vi "Beampointing_Multi_HTU_TRA_diode.vi"() -> ()   [LabVIEW 2013]
uses:
  Shared/GUI_Template/GUI_master/tcp_new_data_event.ctl
  Shared/GUI_Template/GUI_master/tcp new data cluster.ctl
  Ctrs/beam detection.ctl
  GUI_Beampointing_single_TRA/Ctrs/move.ctl
  General GUIs/Device GUIs/GUI_Cameras/Controls/Crosshair type def.ctl
  <vilib>/Utility/file.llb/Read From Spreadsheet File (string).vi
  <userlib>/_OpenG.lib/array/array.llb/Filter 1D Array with Scalar (String)__ogtk.vi
  <vilib>/Analysis/NI_AALBase.lvlib
  <vilib>/vision/NI_Vision_Development_Module.lvlib
  <vilib>/Utility/file.llb/Write To Spreadsheet File (string).vi
panel:
  in  "Position.Axis 5::98":dbl=3.9798 caption="Motor Axis 1" min=0.0 max=6.0 format="%#_6f"
  in  "Position.Axis 6::98":dbl=1.14981 caption="Motor Axis 1" min=0.0 max=6.0 format="%#_6f"
  in  "Position.Axis 5::99":dbl=-0.0 caption="Motor Axis 1" min=0.0 max=6.0 format="%#_6f"
  in  "Position.Axis 6::99":dbl=-0.0 caption="Motor Axis 1" min=0.0 max=6.0 format="%#_6f"
  in  "Position.Axis 6::97":dbl=2.92108 caption="Motor Axis 1" min=0.0 max=6.0 format="%#_6f"
  in  "Position.Axis 4::97":dbl=2.91162 caption="Motor Axis 1" min=0.0 max=6.0 format="%#_6f"
  in  "Position.Axis 5::97":dbl=5.23276 caption="Motor Axis 1" min=0.0 max=6.0 format="%#_6f"
  in  "Position.Axis 4::98":dbl=1.88847 caption="Motor Axis 1" min=0.0 max=6.0 format="%#_6f"
  in  "Position.Axis 3::99":dbl=3.28064 caption="Motor Axis 1" min=0.0 max=6.0 format="%#_6f"
  in  "Position.Axis 4::99":dbl=5.63109 caption="Motor Axis 1" min=0.0 max=6.0 format="%#_6f"
  out "error out 3":errorcluster
  out "Array 3":sgl[](array[numeric])=[7.892375, 6.4410686, 0.40833333, 2.2805147, 5.7728376, 8.5543, 6.1752, 41.382236, 0.0, 0.0, 0.0, 0.0]
  in  "GUIdevice 97":string="U_TRAServer02"
  in  "GUIdevice 98":string="U_TRAServer03"
  in  "Position.Axis 1::97":dbl=2.68788 caption="Motor Axis 1" min=0.0 max=6.0 format="%#_6f"
  in  "Position.Axis 2::97":dbl=2.50302 caption="Motor Axis 1" min=0.0 max=6.0 format="%#_6f"
  in  "Position.Axis 3::97":dbl=3.44716 caption="Motor Axis 1" min=0.0 max=6.0 format="%#_6f"
  in  "Position.Axis 1::98":dbl=2.61382 caption="Motor Axis 1" min=0.0 max=6.0 format="%#_6f"
  in  "Position.Axis 2::98":dbl=0.97888 caption="Motor Axis 1" min=0.0 max=6.0 format="%#_6f"
  in  "Position.Axis 3::98":dbl=5.18289 caption="Motor Axis 1" min=0.0 max=6.0 format="%#_6f"
  in  "save path":path=path "W:/BP_DATA"
  out "size(s) 6":i32=12
  out "config path":string="C:\\GEECS\\Developers Version\\source\\Bella center GUIs\\GUI_Beampointing_multi\\20190502_HTU_diode.cfg"
  out "motor refs 7":refnum<vi>[](array[refnum])
  out "Moving Y":string
  out "Moving X":string
  out "particles":T1(array[cluster])=[{"Area"=1173.0, "Number of Holes"=0.0, "Bounding Rect"={"Left"=82.0, "Top"=87.0, "Right"=120.0, "Bottom"=129.0}, "Center of Mass"={"X"=99.91133844842285, "Y"=109.06734867860187}, "Orientation"=119.37802063554284, "Dimensions"={"Width"=38.0, "Height"=42.0}}]
  out "motor refs 6":refnum<vi>[](array[refnum])
  out "millisecond timer value":u32=1735081648
  out "motor refs 5":refnum<vi>[](array[refnum])
  out "appended path":path=path "C:/GEECS/Developers Version/source/Bella center GUIs/GUI_Beampointing_multi/defaultDevices_ HTU_diode.txt"
  out "motor refs 4":refnum<vi>[](array[refnum])
  in  "active Axis ref 3":cluster{"Ref X":refnum<vi>, "Ref Y":refnum<vi>}
  out "motor refs 3":refnum<vi>[](array[refnum])
  in  "active man refs":cluster{"Ref X":refnum<vi>, "Ref Y":refnum<vi>}
  out "motor refs 2":refnum<vi>[](array[refnum])
  in  "Numeric":dbl=1.0
  out "Current State":string="Exit"
  in  "output cluster 2":T5 {"detection para"."smal para"."Measurement Parameter" items=["Center of Mass X", "Center of Mass Y", "First Pixel X", "First Pixel Y", "Bounding Rect Left", "Bounding Rect Top", "Bounding Rect Right", "Bounding Rect Bottom", "Max Feret Diameter Start X", "Max Feret Diameter Start Y", "Max Feret Diameter End X", "Max Feret Diameter End Y", "Max Horiz. Segment Length Left", "Max Horiz. Segment Length Right", "Max Horiz. Segment Length Row", "-", "Bounding Rect Width", "Bounding Rect Height", "Bounding Rect Diagonal", "Perimeter", "Convex Hull Perimeter", "Holes' Perimeter", "Max Feret Diameter", "Equivalent Ellipse Major Axis", "Equivalent Ellipse Minor Axis", "Equivalent Ellipse Minor Axis (Feret)", "Equivalent Rect Long Side", "Equivalent Rect Short Side", "Equivalent Rect Diagonal", "Equivalent Rect Short Side (Feret)", "Average Horiz. Segment Length", "Average Vert. Segment Length", "Hydraulic Radius", "Waddel Disk Diameter", "-", "Area", "Holes' Area", "Particle & Holes' Area", "Convex Hull Area", "Image Area", "-", "Number of Holes", "Number of Horiz. Segments", "Number of Vert. Segments", "-", "Orientation", "Max Feret Diameter Orientation", "-", "% Area/Image Area", "% Area/(Particle & Holes' Area)", "Ratio of Equivalent Ellipse Axes", "Ratio of Equivalent Rect Sides", "-", "Elongation Factor", "Compactness Factor", "Heywood Circularity Factor", "Type Factor", "-", "Sum X", "Sum Y", "Sum XX", "Sum XY", "Sum YY", "Sum XXX", "Sum XXY", "Sum XYY", "Sum YYY", "-", "Moment of Inertia XX", "Moment of Inertia XY", "Moment of Inertia YY", "Moment of Inertia XXX", "Moment of Inertia XXY", "Moment of Inertia XYY", "Moment of Inertia YYY", "Norm. Moment of Inertia XX", "Norm. Moment of Inertia XY", "Norm. Moment of Inertia YY", "Norm. Moment of Inertia XXX", "Norm. Moment of Inertia XXY", "Norm. Moment of Inertia XYY", "Norm. Moment of Inertia YYY", "Hu Moment 1", "Hu Moment 2", "Hu Moment 3", "Hu Moment 4", "Hu Moment 5", "Hu Moment 6", "Hu Moment 7"]; "detection para"."smal para"."Range Lower Value" format="%.2f"; "detection para"."smal para"."Range Upper Value" format="%.2f"; "detection para"."detection method" items=["clustering", "entropy", "metric", "moments", "inter-class variance"]; "detection para"."Filter" items=["No Filter", "Median Filter", "Low Pass Filter"]}
  out "CCDs":string[](array[string])=["UC_TubeIn", "UC_CompIn", "UC_DMSurface", "UC_BCaveIn", "UC_OAPin1", "UC_OAPin2", "UC_Beamline_In", "UC_Beamline_Out", "", "", "", ""]
  in  "GUIdevice 12":string
  in  "GUIdevice 11":string
  in  "GUIdevice 10":string
  in  "GUIdevice 9":string
  out "error out 2":errorcluster
  in  "active cams":string[](array[string])
  in  "Motor Y":dbl[][](array[numeric])
  in  "Motor X":dbl[][](array[numeric])
  out "Names":string[](array[string])=["TubeIn", "CompIn", "U_TRA1_56", "BCaveIn", "OAPIn1", "DMIn", "OAPin2", "U_TRA2_34", "Beamline_In"]
  in  "Offset X stats":dbl[][](array[numeric])
  in  "Offset Y stats":dbl[][](array[numeric])
  out "Box":T6(array[cluster])=[{"Left"=82.0, "Top"=87.0, "Right"=120.0, "Bottom"=129.0}, {"Left"=147.0, "Top"=140.0, "Right"=258.0, "Bottom"=261.0}, {"Left"=55.0, "Top"=59.0, "Right"=64.0, "Bottom"=71.0}, {"Left"=153.0, "Top"=123.0, "Right"=189.0, "Bottom"=158.0}, {"Left"=160.0, "Top"=192.0, "Right"=208.0, "Bottom"=240.0}, {"Left"=48.0, "Top"=38.0, "Right"=70.0, "Bottom"=57.0}, {"Left"=63.0, "Top"=115.0, "Right"=156.0, "Bottom"=205.0}, {"Left"=176.0, "Top"=170.0, "Right"=237.0, "Bottom"=233.0}]
  in  "Tab Cams":enum32{"Config ", "Main", "History"}(tab)=enum."Main"
  in  "associated motors":T7={"Motor CCD 1"=0, "Motor CCD 2"=1, "Motor CCD 3"=5, "Motor CCD 4"=3, "Motor CCD 5"=4, "Motor CCD 6"=6, "Motor CCD 7"=8, "Motor CCD 8"=7, "Motor CCD 9"=0, "Motor CCD 10"=0, "Motor CCD 11"=0, "Motor CCD 12"=0} {"Motor CCD 12" items=["TubeIn", "CompIn", "U_TRA1_56", "BCaveIn", "OAPIn1", "DMIn", "OAPin2", "U_TRA2_34", "Beamline_In"]; "Motor CCD 11" items=["TubeIn", "CompIn", "U_TRA1_56", "BCaveIn", "OAPIn1", "DMIn", "OAPin2", "U_TRA2_34", "Beamline_In"]; "Motor CCD 10" items=["TubeIn", "CompIn", "U_TRA1_56", "BCaveIn", "OAPIn1", "DMIn", "OAPin2", "U_TRA2_34", "Beamline_In"]; "Motor CCD 9" items=["TubeIn", "CompIn", "U_TRA1_56", "BCaveIn", "OAPIn1", "DMIn", "OAPin2", "U_TRA2_34", "Beamline_In"]; "Motor CCD 8" items=["TubeIn", "CompIn", "U_TRA1_56", "BCaveIn", "OAPIn1", "DMIn", "OAPin2", "U_TRA2_34", "Beamline_In"]; "Motor CCD 7" items=["TubeIn", "CompIn", "U_TRA1_56", "BCaveIn", "OAPIn1", "DMIn", "OAPin2", "U_TRA2_34", "Beamline_In"]; "Motor CCD 6" items=["TubeIn", "CompIn", "U_TRA1_56", "BCaveIn", "OAPIn1", "DMIn", "OAPin2", "U_TRA2_34", "Beamline_In"]; "Motor CCD 5" items=["TubeIn", "CompIn", "U_TRA1_56", "BCaveIn", "OAPIn1", "DMIn", "OAPin2", "U_TRA2_34", "Beamline_In"]; "Motor CCD 4" items=["TubeIn", "CompIn", "U_TRA1_56", "BCaveIn", "OAPIn1", "DMIn", "OAPin2", "U_TRA2_34", "Beamline_In"]; "Motor CCD 3" items=["TubeIn", "CompIn", "U_TRA1_56", "BCaveIn", "OAPIn1", "DMIn", "OAPin2", "U_TRA2_34", "Beamline_In"]; "Motor CCD 2" items=["TubeIn", "CompIn", "U_TRA1_56", "BCaveIn", "OAPIn1", "DMIn", "OAPin2", "U_TRA2_34", "Beamline_In"]; "Motor CCD 1" items=["TubeIn", "CompIn", "U_TRA1_56", "BCaveIn", "OAPIn1", "DMIn", "OAPin2", "U_TRA2_34", "Beamline_In"]}
  out "Cameras":T8={"[0]"="UC_TubeIn", "[1]"="UC_CompIn", "[2]"="UC_DMSurface", "[3]"="UC_BCaveIn", "[4]"="UC_OAPin1", "[5]"="UC_OAPin2", "[6]"="UC_Beamline_In", "[7]"="UC_Beamline_Out", "[8]"="", "[8] 2"="", "[8] 3"="", "[8] 4"=""}
  out "Status":cluster{i32, i32, "Centroid X":dbl[][]}(graph)
  in  "Exposure:12":dbl=0.095 min=0.0001 max=1.0 format="%#_6f"
  in  "Triggerdelay::12":dbl=0.003 min=0.0 max=0.09 format="%#_6f"
  in  "Exposure::11":dbl=0.095 min=0.0001 max=1.0 format="%#_6f"
  in  "Triggerdelay::11":dbl=0.003 min=0.0 max=0.09 format="%#_6f"
  in  "Exposure::10":dbl=0.095 min=0.0001 max=1.0 format="%#_6f"
  in  "Triggerdelay::10":dbl=0.003 min=0.0 max=0.09 format="%#_6f"
  in  "Exposure::9":dbl=0.095 min=2e-05 max=1.0 format="%#_6f"
  in  "Triggerdelay::9":dbl=0.003 min=30.0 max=1000000.0 format="%#_6f"
  in  "Trigger::9":bool
  in  "Trigger::10":bool caption="Trigger:10"
  in  "Trigger::11":bool
  in  "Trigger::12":bool
  in  "Target.Y::9":dbl=45.0 caption="T9y" min=0.0 max=2000.0 format="%#_6f"
  in  "Target.X::9":dbl=47.0 caption="Tx9" min=0.0 max=2000.0 format="%#_6f"
  in  "Target.Y::10":dbl=45.0 caption="T10y" min=0.0 max=2000.0 format="%#_6f"
  in  "Target.X::10":dbl=47.0 caption="T10x" min=0.0 max=2000.0 format="%#_6f"
  in  "Target.Y::11":dbl=45.0 caption="T11y" min=0.0 max=2000.0 format="%#_6f"
  in  "Target.X::11":dbl=47.0 caption="T11x" min=0.0 max=2000.0 format="%#_6f"
  in  "Target.Y::12":dbl=45.0 caption="T12y" min=0.0 max=2000.0 format="%#_6f"
  in  "Target.X::12":dbl=47.0 caption="T12x" min=0.0 max=2000.0 format="%#_6f"
  in  "Exposure::8":dbl=0.080003 min=0.0001 max=1.0 format="%#_6f"
  in  "Triggerdelay::8":dbl=150001.049042 min=20.0 max=500000.0 format="%#_6f"
  in  "Trigger::8":bool=TRUE
  in  "Target.Y::8":dbl=200.0 caption="T8y" min=0.0 max=2000.0 format="%#_6f"
  in  "Target.X::8":dbl=205.0 caption="T8x" min=0.0 max=2000.0 format="%#_6f"
  in  "Target.Y::7":dbl=162.0 caption="T7x" min=0.0 max=2000.0 format="%#_6f"
  in  "Target.X::7":dbl=110.0 caption="T7y" min=0.0 max=2000.0 format="%#_6f"
  in  "Target.Y::6":dbl=47.0 caption="T6y" min=0.0 max=2000.0 format="%#_6f"
  in  "Target.X::6":dbl=58.0 caption="T6x" min=0.0 max=2000.0 format="%#_6f"
  in  "Target.Y::5":dbl=215.0 caption="T5y" min=0.0 max=2000.0 format="%#_6f"
  in  "Target.X::5":dbl=183.0 caption="T5x" min=0.0 max=2000.0 format="%#_6f"
  in  "Target.Y::4":dbl=140.0 caption="T4y" min=0.0 max=2000.0 format="%#_6f"
  in  "Target.X::4":dbl=171.0 caption="T4x" min=0.0 max=2000.0 format="%#_6f"
  in  "Target.Y::3":dbl=65.0 caption="T3y" min=0.0 max=2000.0 format="%#_6f"
  in  "Target.X::3":dbl=59.0 caption="T3x" min=0.0 max=2000.0 format="%#_6f"
  in  "Target.Y::2":dbl=200.0 caption="T2y" min=0.0 max=2000.0 format="%#_6f"
  in  "Target.X::2":dbl=203.0 caption="T2x" min=0.0 max=2000.0 format="%#_6f"
  in  "Target.Y::1":dbl=109.0 caption="T1y" min=0.0 max=2000.0 format="%#_6f"
  in  "Target.X::1":dbl=100.0 caption="T1x" min=0.0 max=2000.0 format="%#_6f"
  in  "Exposure::7":dbl=0.049982 min=0.0001 max=1.0 format="%#_6f"
  in  "Triggerdelay::7":dbl=50000.13113 min=0.0 max=900000.0 format="%#_6f"
  in  "Trigger::7":bool=TRUE
  in  "Exposure::6":dbl=0.3 min=0.0001 max=1.0 format="%#_6f"
  in  "Triggerdelay::6":dbl=50000.0 min=1.0 max=900000.0 format="%#_6f"
  in  "Trigger::6":bool=TRUE
  in  "Exposure::5":dbl=0.2 min=0.0001 max=1.0 format="%#_6f"
  in  "Triggerdelay::5":dbl=50000.0 min=0.0 max=100000.0 format="%#_6f"
  in  "Trigger::5":bool=TRUE
  in  "Exposure::4":dbl=10000.0 min=10.0 max=1000000.0 format="%#_6f"
  in  "Triggerdelay::4":dbl=50000.0 min=10.0 max=1000000.0 format="%#_6f"
  in  "Trigger::4":bool=TRUE
  in  "Exposure::3":dbl=200000.0 min=20.0 max=1000000.0 format="%#_6f"
  in  "Triggerdelay::3":dbl=50000.0 min=10.0 max=500000.0 format="%#_6f"
  in  "Trigger::3":bool=TRUE
  in  "Exposure::2":dbl=0.01 min=2e-05 max=1.0 format="%#_6f"
  in  "Triggerdelay::2":dbl=50000.0 min=0.0 max=100000.0 format="%#_6f"
  in  "Trigger::2":bool=TRUE
  out "image::1":T9(plugin-control) caption="UC_TubeIn"
  out "image::2":T9(plugin-control) caption="UC_CompIn"
  out "image::3":T9(plugin-control) caption="UC_DMSurface"
  out "image::4":T9(plugin-control) caption="UC_BCaveIn"
  out "image::5":T9(plugin-control) caption="UC_OAPin1"
  out "image::6":T9(plugin-control) caption="UC_OAPin2"
  out "image::7":T9(plugin-control) caption="UC_Beamline_In"
  out "image::8":T9(plugin-control) caption="UC_Beamline_Out"
  in  "Exposure::1":dbl=3000.0 min=50.0 max=500000.0 format="%#_6f"
  in  "Triggerdelay::1":dbl=50000.0 min=0.01 max=999000.0 format="%#_6f"
  in  "Trigger::1":bool=TRUE
  in  "UDP error message":string
  out "required Y":bool[](array[boolean])=[FALSE, FALSE, FALSE, FALSE, TRUE, FALSE, TRUE, FALSE]
  out "required X":bool[](array[boolean])=[FALSE, FALSE, FALSE, TRUE, TRUE, FALSE, TRUE, FALSE]
  out "detected":bool[](array[boolean])=[TRUE, TRUE, TRUE, TRUE, TRUE, TRUE, TRUE, TRUE]
  out "name array":string[](array[string])=["UC_TubeIn", "UC_CompIn", "UC_DMSurface", "UC_BCaveIn", "UC_OAPin1", "UC_OAPin2", "UC_Beamline_In", "UC_Beamline_Out"]
  out "image::9":T9(plugin-control) caption="UC_ModeImager"
  out "image::10":T9(plugin-control)
  out "image::11":T9(plugin-control)
  out "image::12":T9(plugin-control)
  out "speedmode X":bool[](array[boolean])=[FALSE, FALSE, TRUE, FALSE, FALSE, FALSE, FALSE, FALSE]
  out "speedmode Y":bool[](array[boolean])=[FALSE, FALSE, TRUE, FALSE, FALSE, FALSE, FALSE, FALSE]
  out "CCD 9":cluster{timestamp[], dbl[]}[](graph)
  out "CCD 10":cluster{timestamp[], dbl[]}[](graph)
  out "CCD 11":cluster{timestamp[], dbl[]}[](graph)
  out "CCD 12":cluster{timestamp[], dbl[]}[](graph)
  out "CCD 5":cluster{timestamp[], dbl[]}[](graph)
  out "CCD 6":cluster{timestamp[], dbl[]}[](graph)
  out "CCD 7":cluster{timestamp[], dbl[]}[](graph)
  out "CCD 8":cluster{timestamp[], dbl[]}[](graph)
  out "CCD 2":cluster{timestamp[], dbl[]}[](graph)
  out "CCD 1":cluster{timestamp[], dbl[]}[](graph)
  out "CCD 3":cluster{timestamp[], dbl[]}[](graph)
  out "CCD 4":cluster{timestamp[], dbl[]}[](graph)
  in  "History Size":i32=500
  out "History Index":i32=1
  in  "Feedback Global":bool
  in  "detection para":T3[](array[typedef])=[{"Filter"=1, "Filter Para"={"X Size"=5, "Y Size"=5, "% Tolerance"=1}, "detection method"=4, "smal para"=[{"Measurement Parameter"=35, "Range Lower Value"=0.0, "Range Upper Value"=0.0, "Range"=TRUE, "Measurement Type"=FALSE}], "Remove small Objects"=TRUE, "Restrict to round Objects"=FALSE}, {"Filter"=1, "Filter Para"={"X Size"=5, "Y Size"=5, "% Tolerance"=1}, "detection method"=4, "smal para"=[{"Measurement Parameter"=35, "Range Lower Value"=0.0, "Range Upper Value"=500.0, "Range"=FALSE, "Measurement Type"=FALSE}], "Remove small Objects"=TRUE, "Restrict to round Objects"=FALSE}, {"Filter"=1, "Filter Para"={"X Size"=5, "Y Size"=5, "% Tolerance"=1}, "detection method"=4, "smal para"=[{"Measurement Parameter"=35, "Range Lower Value"=0.0, "Range Upper Value"=500.0, "Range"=TRUE, "Measurement Type"=FALSE}], "Remove small Objects"=TRUE, "Restrict to round Objects"=FALSE}, {"Filter"=1, "Filter Para"={"X Size"=5, "Y Size"=5, "% Tolerance"=1}, "detection method"=4, "smal para"=[{"Measurement Parameter"=35, "Range Lower Value"=0.0, "Range Upper Value"=500.0, "Range"=TRUE, "Measurement Type"=FALSE}], "Remove small Objects"=TRUE, "Restrict to round Objects"=FALSE}, {"Filter"=1, "Filter Para"={"X Size"=5, "Y Size"=5, "% Tolerance"=1}, "detection method"=4, "smal para"=[{"Measurement Parameter"=35, "Range Lower Value"=0.0, "Range Upper Value"=500.0, "Range"=TRUE, "Measurement Type"=FALSE}], "Remove small Objects"=TRUE, "Restrict to round Objects"=FALSE}, {"Filter"=1, "Filter Para"={"X Size"=5, "Y Size"=5, "% Tolerance"=1}, "detection method"=4, "smal para"=[{"Measurement Parameter"=35, "Range Lower Value"=0.0, "Range Upper Value"=500.0, "Range"=TRUE, "Measurement Type"=FALSE}], "Remove small Objects"=TRUE, "Restrict to round Objects"=FALSE}, {"Filter"=1, "Filter Para"={"X Size"=5, "Y Size"=5, "% Tolerance"=1}, "detection method"=4, "smal para"=[{"Measurement Parameter"=35, "Range Lower Value"=0.0, "Range Upper Value"=500.0, "Range"=TRUE, "Measurement Type"=FALSE}], "Remove small Objects"=TRUE, "Restrict to round Objects"=FALSE}, {"Filter"=1, "Filter Para"={"X Size"=5, "Y Size"=5, "% Tolerance"=1}, "detection method"=3, "smal para"=[{"Measurement Parameter"=35, "Range Lower Value"=0.0, "Range Upper Value"=0.0, "Range"=FALSE, "Measurement Type"=FALSE}], "Remove small Objects"=TRUE, "Restrict to round Objects"=FALSE}, {"Filter"=1, "Filter Para"={"X Size"=5, "Y Size"=5, "% Tolerance"=1}, "detection method"=4, "smal para"=[{"Measurement Parameter"=35, "Range Lower Value"=0.0, "Range Upper Value"=0.0, "Range"=FALSE, "Measurement Type"=FALSE}], "Remove small Objects"=TRUE, "Restrict to round Objects"=FALSE}, {"Filter"=1, "Filter Para"={"X Size"=5, "Y Size"=5, "% Tolerance"=1}, "detection method"=4, "smal para"=[{"Measurement Parameter"=35, "Range Lower Value"=0.0, "Range Upper Value"=500.0, "Range"=TRUE, "Measurement Type"=FALSE}], "Remove small Objects"=TRUE, "Restrict to round Objects"=FALSE}, {"Filter"=1, "Filter Para"={"X Size"=5, "Y Size"=5, "% Tolerance"=1}, "detection method"=4, "smal para"=[{"Measurement Parameter"=35, "Range Lower Value"=0.0, "Range Upper Value"=500.0, "Range"=TRUE, "Measurement Type"=FALSE}], "Remove small Objects"=TRUE, "Restrict to round Objects"=FALSE}, {"Filter"=1, "Filter Para"={"X Size"=5, "Y Size"=5, "% Tolerance"=1}, "detection method"=4, "smal para"=[{"Measurement Parameter"=35, "Range Lower Value"=0.0, "Range Upper Value"=500.0, "Range"=TRUE, "Measurement Type"=FALSE}], "Remove small Objects"=TRUE, "Restrict to round Objects"=FALSE}] {"smal para"."Measurement Parameter" items=["Center of Mass X", "Center of Mass Y", "First Pixel X", "First Pixel Y", "Bounding Rect Left", "Bounding Rect Top", "Bounding Rect Right", "Bounding Rect Bottom", "Max Feret Diameter Start X", "Max Feret Diameter Start Y", "Max Feret Diameter End X", "Max Feret Diameter End Y", "Max Horiz. Segment Length Left", "Max Horiz. Segment Length Right", "Max Horiz. Segment Length Row", "-", "Bounding Rect Width", "Bounding Rect Height", "Bounding Rect Diagonal", "Perimeter", "Convex Hull Perimeter", "Holes' Perimeter", "Max Feret Diameter", "Equivalent Ellipse Major Axis", "Equivalent Ellipse Minor Axis", "Equivalent Ellipse Minor Axis (Feret)", "Equivalent Rect Long Side", "Equivalent Rect Short Side", "Equivalent Rect Diagonal", "Equivalent Rect Short Side (Feret)", "Average Horiz. Segment Length", "Average Vert. Segment Length", "Hydraulic Radius", "Waddel Disk Diameter", "-", "Area", "Holes' Area", "Particle & Holes' Area", "Convex Hull Area", "Image Area", "-", "Number of Holes", "Number of Horiz. Segments", "Number of Vert. Segments", "-", "Orientation", "Max Feret Diameter Orientation", "-", "% Area/Image Area", "% Area/(Particle & Holes' Area)", "Ratio of Equivalent Ellipse Axes", "Ratio of Equivalent Rect Sides", "-", "Elongation Factor", "Compactness Factor", "Heywood Circularity Factor", "Type Factor", "-", "Sum X", "Sum Y", "Sum XX", "Sum XY", "Sum YY", "Sum XXX", "Sum XXY", "Sum XYY", "Sum YYY", "-", "Moment of Inertia XX", "Moment of Inertia XY", "Moment of Inertia YY", "Moment of Inertia XXX", "Moment of Inertia XXY", "Moment of Inertia XYY", "Moment of Inertia YYY", "Norm. Moment of Inertia XX", "Norm. Moment of Inertia XY", "Norm. Moment of Inertia YY", "Norm. Moment of Inertia XXX", "Norm. Moment of Inertia XXY", "Norm. Moment of Inertia XYY", "Norm. Moment of Inertia YYY", "Hu Moment 1", "Hu Moment 2", "Hu Moment 3", "Hu Moment 4", "Hu Moment 5", "Hu Moment 6", "Hu Moment 7"]; "smal para"."Range Lower Value" format="%.2f"; "smal para"."Range Upper Value" format="%.2f"; "detection method" items=["clustering", "entropy", "metric", "moments", "inter-class variance"]; "Filter" items=["No Filter", "Median Filter", "Low Pass Filter"]}
  in  "GUIdevice 8":string="UC_Beamline_Out"
  in  "Tab Control":T10(tab)
  in  "alarms":bool
  in  "new tdms":bool
  in  "Save Stats":bool
  in  "Save Config":bool
  in  "Load Config":bool
  in  "update speed [ms]":i32=1000
  in  "img to avg":i32=10 min=3 max=200
  in  "Reset History":bool
  in  "autodetect":bool
  in  "Detection Rate":dbl=0.9 min=0.001 max=1.0
  in  "Center":bool
  in  "Align":bool=TRUE
  in  "Speedmode":dbl=10.0 min=1.0 max=20.0
  in  "device ini":bool
  in  "average centroid":bool
  in  "beam detection para":T3={"Filter"=1, "Filter Para"={"X Size"=5, "Y Size"=5, "% Tolerance"=10}, "detection method"=4, "smal para"=[{"Measurement Parameter"=35, "Range Lower Value"=500.0, "Range Upper Value"=2000.0, "Range"=FALSE, "Measurement Type"=FALSE}], "Remove small Objects"=TRUE, "Restrict to round Objects"=FALSE} {"smal para"."Measurement Parameter" items=["Center of Mass X", "Center of Mass Y", "First Pixel X", "First Pixel Y", "Bounding Rect Left", "Bounding Rect Top", "Bounding Rect Right", "Bounding Rect Bottom", "Max Feret Diameter Start X", "Max Feret Diameter Start Y", "Max Feret Diameter End X", "Max Feret Diameter End Y", "Max Horiz. Segment Length Left", "Max Horiz. Segment Length Right", "Max Horiz. Segment Length Row", "-", "Bounding Rect Width", "Bounding Rect Height", "Bounding Rect Diagonal", "Perimeter", "Convex Hull Perimeter", "Holes' Perimeter", "Max Feret Diameter", "Equivalent Ellipse Major Axis", "Equivalent Ellipse Minor Axis", "Equivalent Ellipse Minor Axis (Feret)", "Equivalent Rect Long Side", "Equivalent Rect Short Side", "Equivalent Rect Diagonal", "Equivalent Rect Short Side (Feret)", "Average Horiz. Segment Length", "Average Vert. Segment Length", "Hydraulic Radius", "Waddel Disk Diameter", "-", "Area", "Holes' Area", "Particle & Holes' Area", "Convex Hull Area", "Image Area", "-", "Number of Holes", "Number of Horiz. Segments", "Number of Vert. Segments", "-", "Orientation", "Max Feret Diameter Orientation", "-", "% Area/Image Area", "% Area/(Particle & Holes' Area)", "Ratio of Equivalent Ellipse Axes", "Ratio of Equivalent Rect Sides", "-", "Elongation Factor", "Compactness Factor", "Heywood Circularity Factor", "Type Factor", "-", "Sum X", "Sum Y", "Sum XX", "Sum XY", "Sum YY", "Sum XXX", "Sum XXY", "Sum XYY", "Sum YYY", "-", "Moment of Inertia XX", "Moment of Inertia XY", "Moment of Inertia YY", "Moment of Inertia XXX", "Moment of Inertia XXY", "Moment of Inertia XYY", "Moment of Inertia YYY", "Norm. Moment of Inertia XX", "Norm. Moment of Inertia XY", "Norm. Moment of Inertia YY", "Norm. Moment of Inertia XXX", "Norm. Moment of Inertia XXY", "Norm. Moment of Inertia XYY", "Norm. Moment of Inertia YYY", "Hu Moment 1", "Hu Moment 2", "Hu Moment 3", "Hu Moment 4", "Hu Moment 5", "Hu Moment 6", "Hu Moment 7"]; "smal para"."Range Lower Value" format="%.2f"; "smal para"."Range Upper Value" format="%.2f"; "detection method" items=["clustering", "entropy", "metric", "moments", "inter-class variance"]; "Filter" items=["No Filter", "Median Filter", "Low Pass Filter"]}
  in  "move config":T2={"Tolerance [%]"=0.5, "Stepsize"=0.001, "Invert Axis"=FALSE, "Invert Direction X"=TRUE, "Invert Direction Y"=FALSE, "enable feedback"=TRUE, "Set Centriod Target"=FALSE}
  in  "Position 2":dbl=1.53813 caption="Stepsize" min=0.0 max=999999.0 format="%_6f"
  in  "Position 1":dbl=1.96058 caption="Stepsize" min=0.0 max=999999.0 format="%_6f"
  in  "Right":bool caption="RelativeMove.Axis 1.CCW::1"
  in  "Left":bool caption="RelativeMove.Axis 1.CW::1"
  in  "Down":bool caption="RelativeMove.Axis. 2.CCW::1"
  in  "Up":bool caption="RelativeMove.Axis 2.CW::1"
  in  "StepSize":dbl=1.0 caption="Stepsize" min=0.0 max=1.0 step=0.001 format="%#_6p"
  in  "active axis refs 2":T11(array[cluster])
  in  "active Axis ref":cluster{"Ref X":refnum<vi>, "Ref Y":refnum<vi>}
  in  "CCDs":u16(ring) items=["UC_TubeIn", "UC_CompIn", "UC_DMSurface", "UC_BCaveIn", "UC_OAPin1", "UC_OAPin2", "UC_Beamline_In", "UC_Beamline_Out", "UC_ModeImager", "", "", ""]
  out "motor refs":refnum<vi>[](array[refnum])
  in  "Position.Axis 2::99":dbl=1.53813 caption="Motor Axis 1" min=0.0 max=6.0 format="%#_6f"
  in  "Position.Axis 1::99":dbl=1.96058 caption="Motor Axis 1" min=0.0 max=6.0 format="%#_6f"
  in  "GUIdevice 99":string="U_TRAServer01"
  in  "move properties":T2[](array[typedef])=[{"Tolerance [%]"=0.1, "Stepsize"=0.0001, "Invert Axis"=TRUE, "Invert Direction X"=FALSE, "Invert Direction Y"=TRUE, "enable feedback"=FALSE, "Set Centriod Target"=FALSE}, {"Tolerance [%]"=0.1, "Stepsize"=0.0001, "Invert Axis"=TRUE, "Invert Direction X"=FALSE, "Invert Direction Y"=TRUE, "enable feedback"=FALSE, "Set Centriod Target"=FALSE}, {"Tolerance [%]"=0.1, "Stepsize"=0.0001, "Invert Axis"=TRUE, "Invert Direction X"=FALSE, "Invert Direction Y"=TRUE, "enable feedback"=FALSE, "Set Centriod Target"=FALSE}, {"Tolerance [%]"=0.1, "Stepsize"=0.0001, "Invert Axis"=TRUE, "Invert Direction X"=FALSE, "Invert Direction Y"=TRUE, "enable feedback"=FALSE, "Set Centriod Target"=FALSE}, {"Tolerance [%]"=0.1, "Stepsize"=0.0001, "Invert Axis"=TRUE, "Invert Direction X"=FALSE, "Invert Direction Y"=TRUE, "enable feedback"=FALSE, "Set Centriod Target"=FALSE}, {"Tolerance [%]"=0.1, "Stepsize"=0.0001, "Invert Axis"=TRUE, "Invert Direction X"=FALSE, "Invert Direction Y"=TRUE, "enable feedback"=FALSE, "Set Centriod Target"=FALSE}, {"Tolerance [%]"=0.1, "Stepsize"=0.0001, "Invert Axis"=TRUE, "Invert Direction X"=FALSE, "Invert Direction Y"=TRUE, "enable feedback"=FALSE, "Set Centriod Target"=FALSE}, {"Tolerance [%]"=0.1, "Stepsize"=0.0001, "Invert Axis"=TRUE, "Invert Direction X"=FALSE, "Invert Direction Y"=TRUE, "enable feedback"=FALSE, "Set Centriod Target"=FALSE}, {"Tolerance [%]"=0.1, "Stepsize"=0.0001, "Invert Axis"=TRUE, "Invert Direction X"=FALSE, "Invert Direction Y"=TRUE, "enable feedback"=FALSE, "Set Centriod Target"=FALSE}, {"Tolerance [%]"=0.1, "Stepsize"=0.0001, "Invert Axis"=TRUE, "Invert Direction X"=FALSE, "Invert Direction Y"=TRUE, "enable feedback"=FALSE, "Set Centriod Target"=FALSE}, {"Tolerance [%]"=0.1, "Stepsize"=0.0001, "Invert Axis"=TRUE, "Invert Direction X"=FALSE, "Invert Direction Y"=TRUE, "enable feedback"=FALSE, "Set Centriod Target"=FALSE}, {"Tolerance [%]"=0.1, "Stepsize"=0.0001, "Invert Axis"=TRUE, "Invert Direction X"=FALSE, "Invert Direction Y"=TRUE, "enable feedback"=FALSE, "Set Centriod Target"=FALSE}, {"Tolerance [%]"=0.1, "Stepsize"=0.0001, "Invert Axis"=TRUE, "Invert Direction X"=FALSE, "Invert Direction Y"=TRUE, "enable feedback"=FALSE, "Set Centriod Target"=FALSE}]
  in  "Time":timestamp[][](array[timestamp])
  in  "Mean Size":dbl[][](array[numeric])
  in  "Size":dbl[][](array[numeric])
  in  "active CCDs":i32(listbox)=1
  in  "Offset Y":dbl[][](array[numeric])
  in  "Offset X":dbl[][](array[numeric])
  in  "Mean Centroid X":dbl[][](array[numeric])
  in  "Mean Centroid Y":dbl[][](array[numeric])
  in  "Centroid Y":dbl[][](array[numeric])
  in  "Centroid X":dbl[][](array[numeric])
  in  "GUIdevice 7":string="UC_Beamline_In"
  in  "GUIdevice 6":string="UC_OAPin2"
  in  "GUIdevice 5":string="UC_OAPin1"
  in  "GUIdevice 4":string="UC_BCaveIn"
  in  "GUIdevice 3":string="UC_DMSurface"
  in  "GUIdevice 2":string="UC_CompIn"
  in  "insert tag":bool=TRUE
  in  "stop":bool
  in  "GUIdevice 1":string="UC_TubeIn"
  out "tcp data event":T12
  out "error IO 2":errorcluster
  # "max"
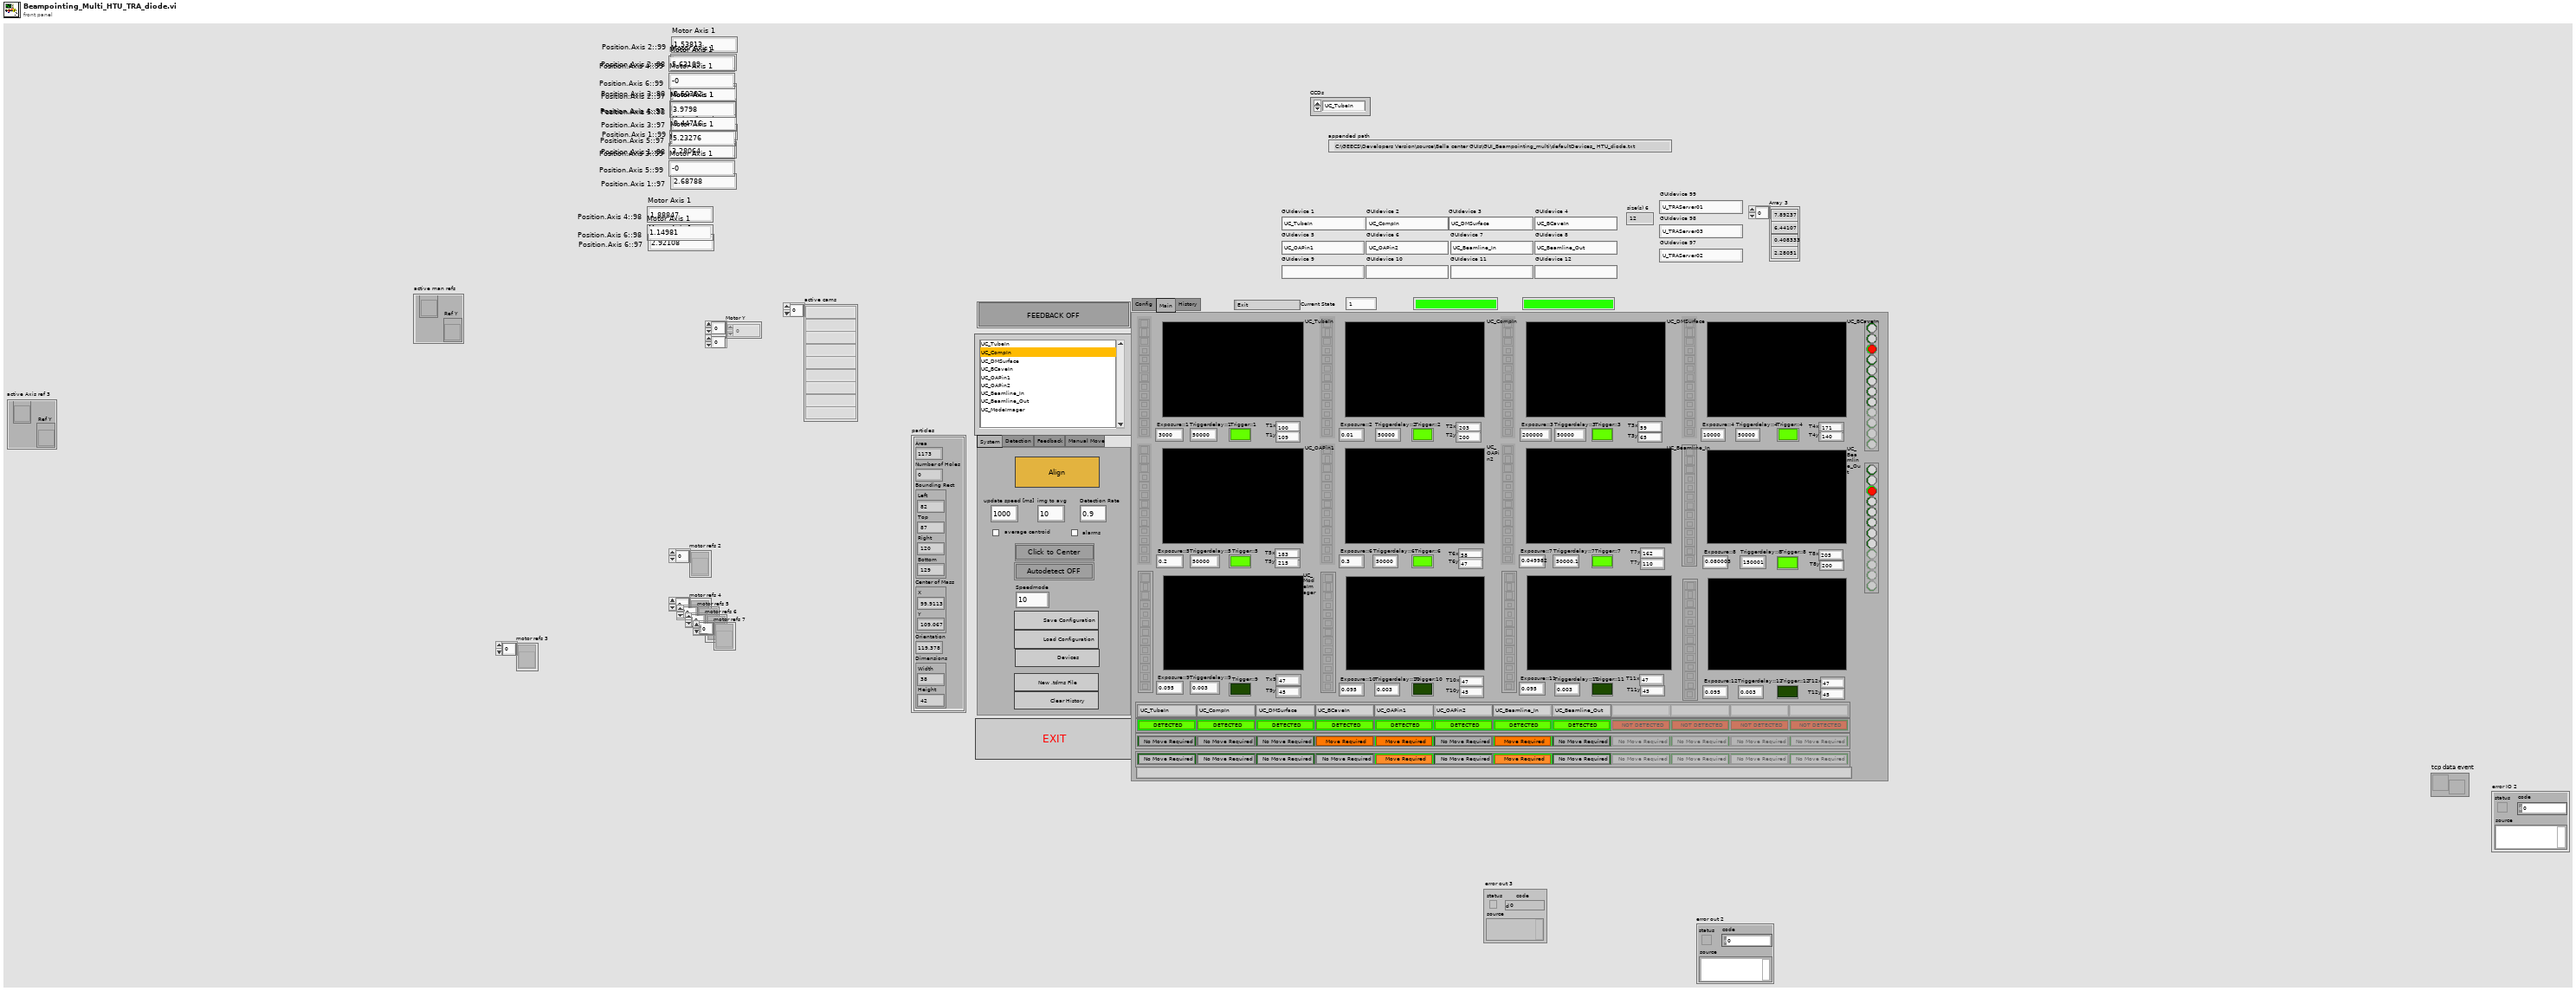
[diagram p1: front panel]
types:
  T1 = cluster{"Area":dbl, "Number of Holes":dbl, "Bounding Rect":cluster{"Left":dbl, "Top":dbl, "Right":dbl, "Bottom":dbl}, "Center of Mass":cluster{"X":dbl, "Y":dbl}, "Orientation":dbl, "Dimensions":cluster{"Width":dbl, "Height":dbl}}[]
  T2 = typedef "move.ctl" = cluster{"Tolerance [%]":dbl, "Stepsize":dbl, "Invert Axis":bool, "Invert Direction X":bool, "Invert Direction Y":bool, "enable feedback":bool, "Set Centriod Target":bool}
  T3 = typedef "beam detection.ctl" = cluster{"Filter":u16, "Filter Para":cluster{"X Size":i32, "Y Size":i32, "% Tolerance":i32}, "detection method":i32, "smal para":cluster{"Measurement Parameter":T4, "Range Lower Value":dbl, "Range Upper Value":dbl, "Range":bool, "Measurement Type":bool}[], "Remove small Objects":bool, "Restrict to round Objects":bool}
  T4 = typedef "Particle Parameters" = i32
  T5 = cluster{"CCDs":string[], "move properties":T2[], "detection para":T3[], "thresholds":cluster{"Lower value":sgl, "Upper value":sgl}[], "Value":cluster{"Motor CCD 1":u16, "Motor CCD 2":u16, "Motor CCD 3":u16, "Motor CCD 4":u16, "Motor CCD 5":u16, "Motor CCD 6":u16, "Motor CCD 7":u16, "Motor CCD 8":u16, "Motor CCD 9":u16, "Motor CCD 10":u16, "Motor CCD 11":u16, "Motor CCD 12":u16}}
  T6 = cluster{"Left":dbl, "Top":dbl, "Right":dbl, "Bottom":dbl}[]
  T7 = cluster{"Motor CCD 1":u16, "Motor CCD 2":u16, "Motor CCD 3":u16, "Motor CCD 4":u16, "Motor CCD 5":u16, "Motor CCD 6":u16, "Motor CCD 7":u16, "Motor CCD 8":u16, "Motor CCD 9":u16, "Motor CCD 10":u16, "Motor CCD 11":u16, "Motor CCD 12":u16}
  T8 = cluster{"[0]":string, "[1]":string, "[2]":string, "[3]":string, "[4]":string, "[5]":string, "[6]":string, "[7]":string, "[8]":string, "[8] 2":string, "[8] 3":string, "[8] 4":string}
  T9 = typedef "IMAQ Image.ctl" = refnum<image>
  T10 = enum32{"System", "Detection", "Feedback", "Manual Move"}
  T11 = cluster{"Ref X":refnum<vi>, "Ref Y":refnum<vi>}[]
  T12 = typedef "tcp_new_data_event.ctl" = refnum<user-event>
  T13 = typedef "tcp new data cluster.ctl" = cluster{"EventEnum":enum16{"new data", "connection status update"}, "Device name":string}
  T14 = enum32{"invalid app kind", "Development System", "Run Time System", "Student Edition", "Embedded LabVIEW", "Evaluation", "Custom"}
  T15 = enum16{"open", "open or create", "create or replace", "create", "open (read-only)"}
  T16 = enum32{"Invalid", "Standard", "Closed", "Hidden", "Minimized", "Maximized"}
  T17 = enum16{"open", "replace", "create", "open or create", "replace or create", "replace or create with confirmation"}
  T18 = enum8{"Enabled", "Disabled", "Disabled and Grayed Out"}
  T19 = typedef "Image Type" = u32
  T20 = cluster{"[0]":string, "[1]":string, "[2]":string, "[3]":string, "[4]":string, "[5]":string, "[6]":string, "[7]":string, "[8]":string, "[9]":string, "[10]":string, "[11]":string}
  T21 = cluster{"Target.X::1":refnum<vi>, "Target.Y::1":refnum<vi>}
  T22 = cluster{"Target.X::2":refnum<vi>, "Target.Y::2":refnum<vi>}
  T23 = cluster{"Target.X::3":refnum<vi>, "Target.Y::3":refnum<vi>}
  T24 = cluster{"Target.X::4":refnum<vi>, "Target.Y::4":refnum<vi>}
  T25 = cluster{"Target.X::5":refnum<vi>, "Target.Y::5":refnum<vi>}
  T26 = cluster{"Target.X::6":refnum<vi>, "Target.Y::6":refnum<vi>}
  T27 = cluster{"Target.X::7":refnum<vi>, "Target.Y::7":refnum<vi>}
  T28 = cluster{"Target.X::8":refnum<vi>, "Target.Y::8":refnum<vi>}
  T29 = cluster{"Target.X::12":refnum<vi>, "Target.Y::12":refnum<vi>}
  T30 = cluster{"Target.X::9":refnum<vi>, "Target.Y::9":refnum<vi>}
  T31 = cluster{"Target.X::10":refnum<vi>, "Target.Y::10":refnum<vi>}
  T32 = cluster{"Target.X::11":refnum<vi>, "Target.Y::11":refnum<vi>}
  T33 = cluster{"Target.X::12":refnum<vi>, "Target.Y::12":refnum<vi>}[]
  T34 = cluster{"Left":dbl, "Top":dbl, "Right":dbl, "Bottom":dbl}
  T35 = cluster{"Core":cluster{"Current VI Reference":refnum<vi>, "Close Panel on Exit?":bool}, "detection para":T3[], "thresholds":cluster{"Lower value":sgl, "Upper value":sgl}[], "Centroid X":dbl[][], "Centroid Y":dbl[][], "img to avg":i32, "Mean Centroid X":dbl[][], "Mean Centroid Y":dbl[][], "Offset X":dbl[][], "Offset Y":dbl[][], "Offset X stats ":dbl[][], "Offset Y stats ":dbl[][], "Size":dbl[][], "Mean Size":dbl[][], "Time":timestamp[][], "move properties":T2[], "active axis refs 2":cluster{"Ref X":refnum<vi>, "Ref Y":refnum<vi>}[], "active ccd":i32, "Feedback global":bool, "Motor X":dbl[][], "Motor Y":dbl[][], "active cams":string[], "Data Value Reference out":refnum<k34>, "active man refs":cluster{"Ref X":refnum<vi>, "Ref Y":refnum<vi>}, "detected":bool[], "speedmode X":bool[], "speedmode Y":bool[], "steps speed X":dbl[], "steps speed Y":dbl[]}
  T36 = cluster{"Current VI Reference":refnum<vi>, "Close Panel on Exit?":bool}
  T37 = cluster{"appended array":timestamp[], "appended array":dbl[]}
  T38 = cluster{"appended array":timestamp[], "appended array":dbl[]}[]
  T39 = typedef "Crosshair type def.ctl" = cluster{"Draw":bool, "Target":cluster{"x":dbl, "y":dbl}, "Size":cluster{"x":dbl, "y":dbl}, "Angle":dbl, "Color":u32, "Thickness":u8, "CrosshairLabel":string}
  T40 = cluster{"Left":i32, "Top":i32, "Right":i32, "Bottom":i32}
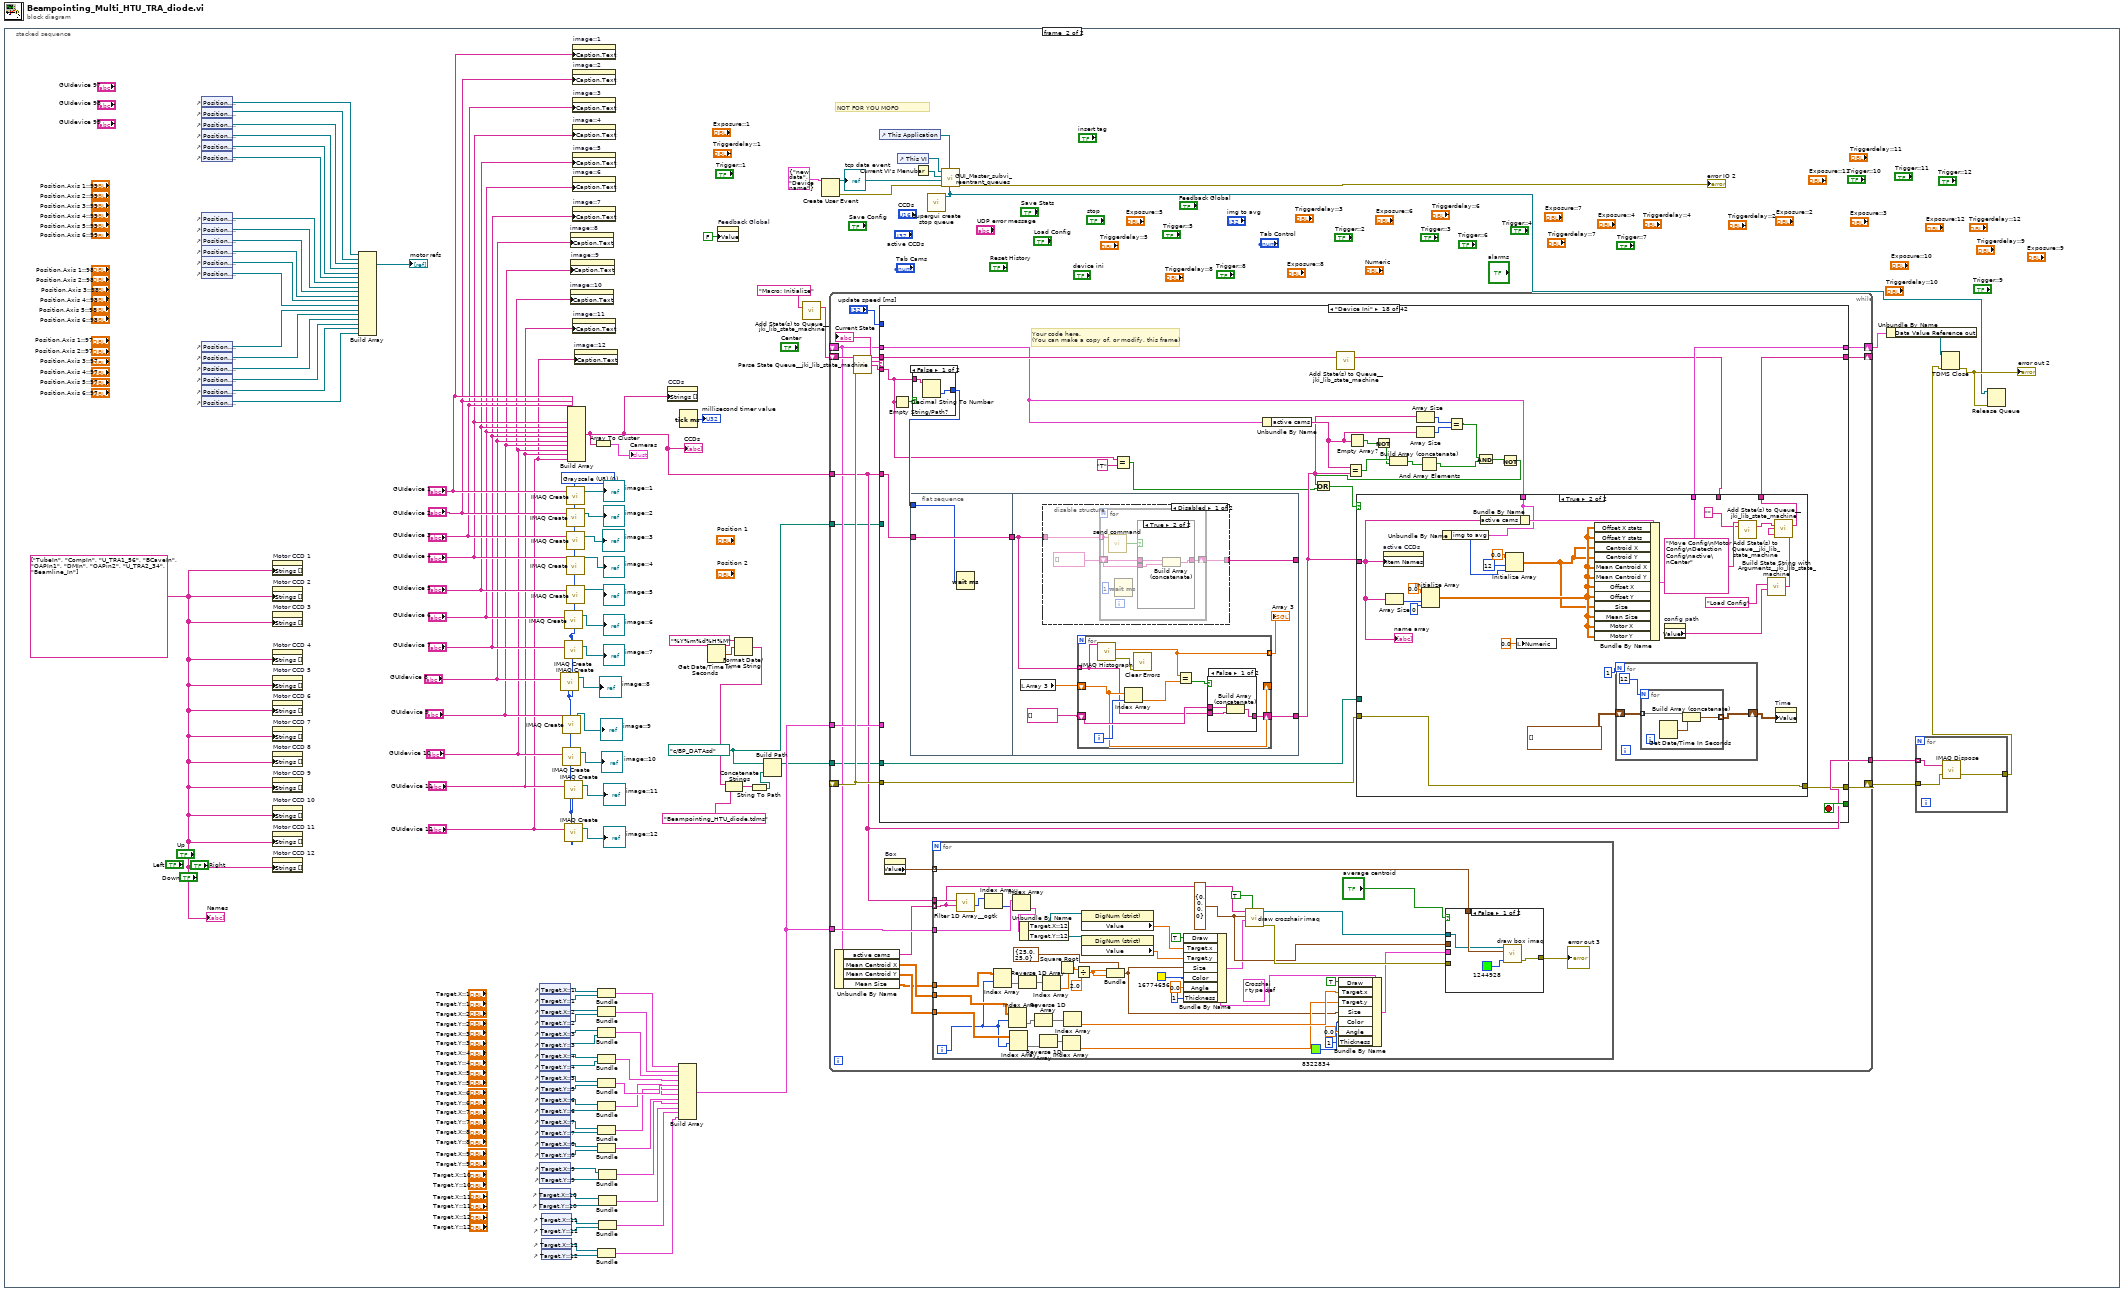
[diagram p0: block diagram]
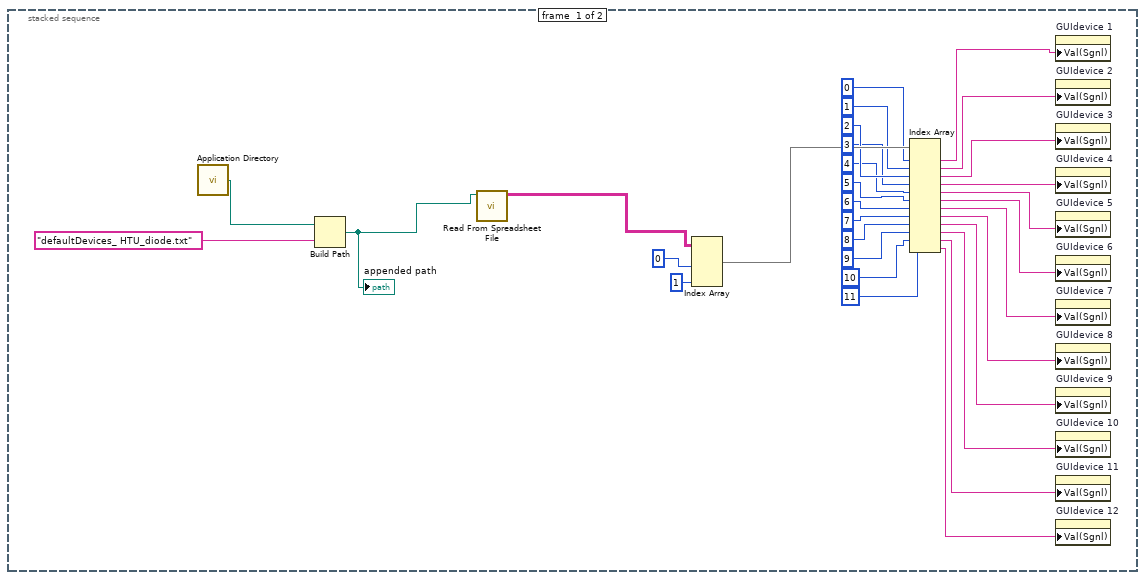
[diagram p2: hidden frame]
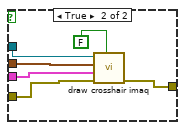
[diagram p3: hidden frame]
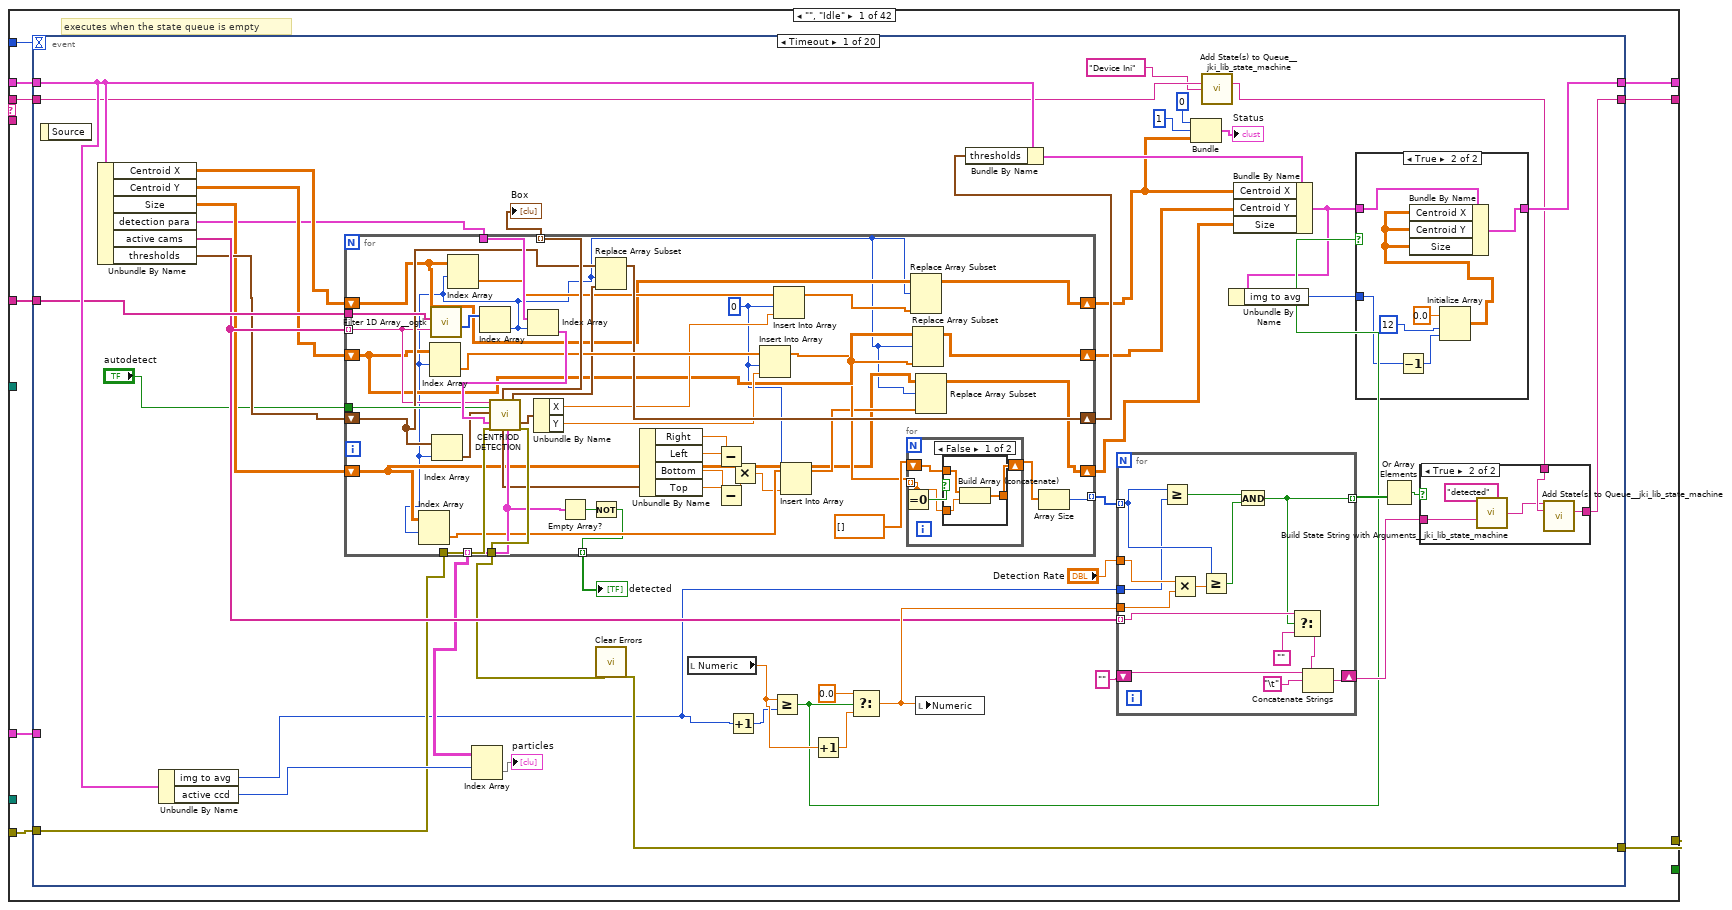
[diagram p4: hidden frame]
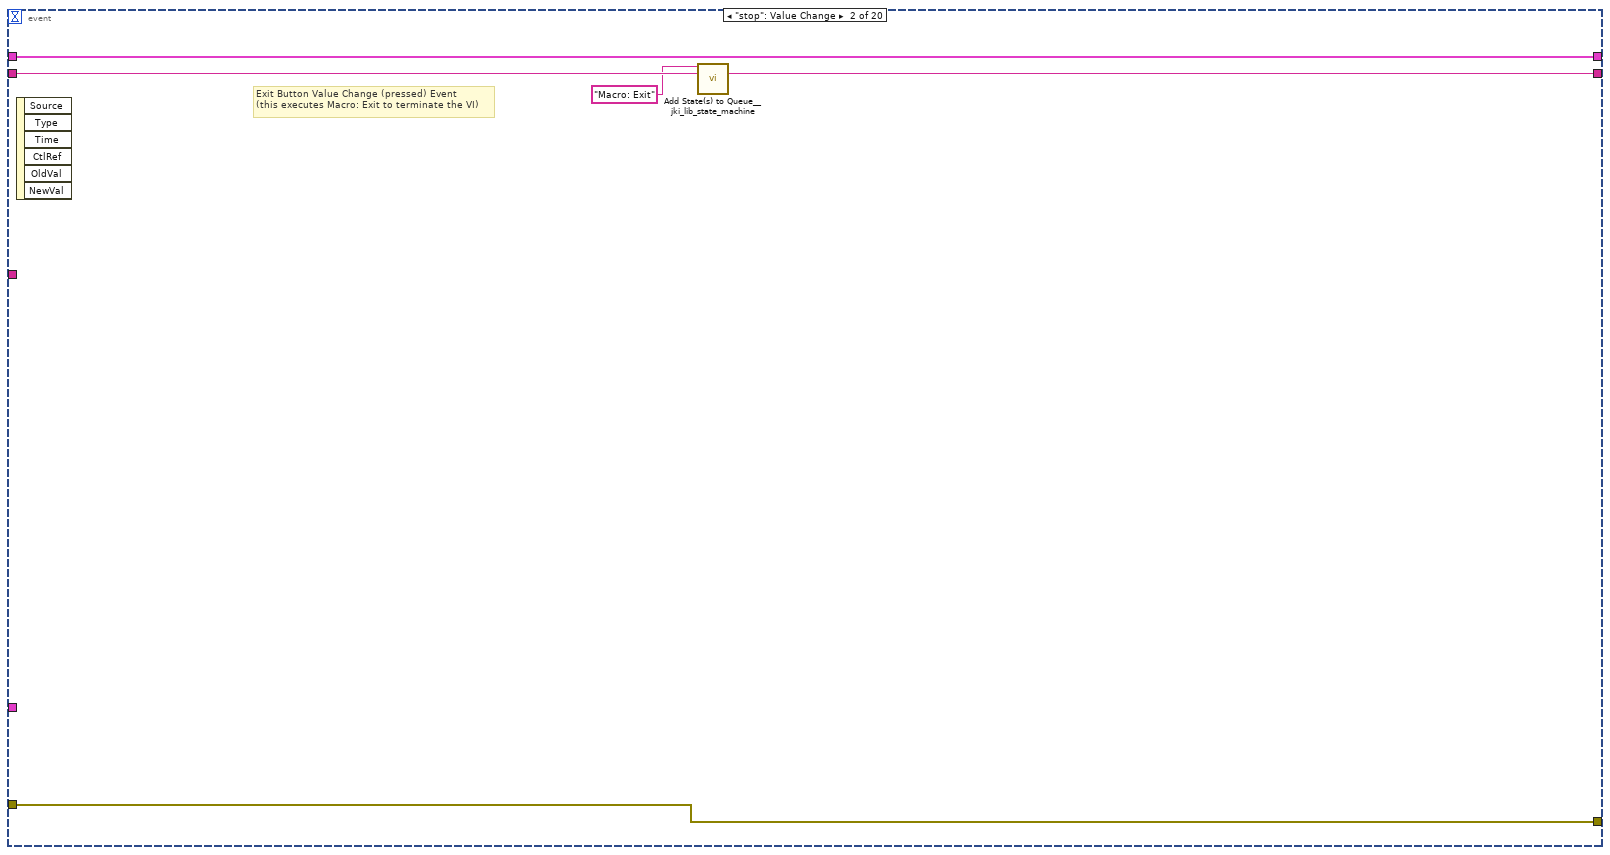
[diagram p8: hidden frame]
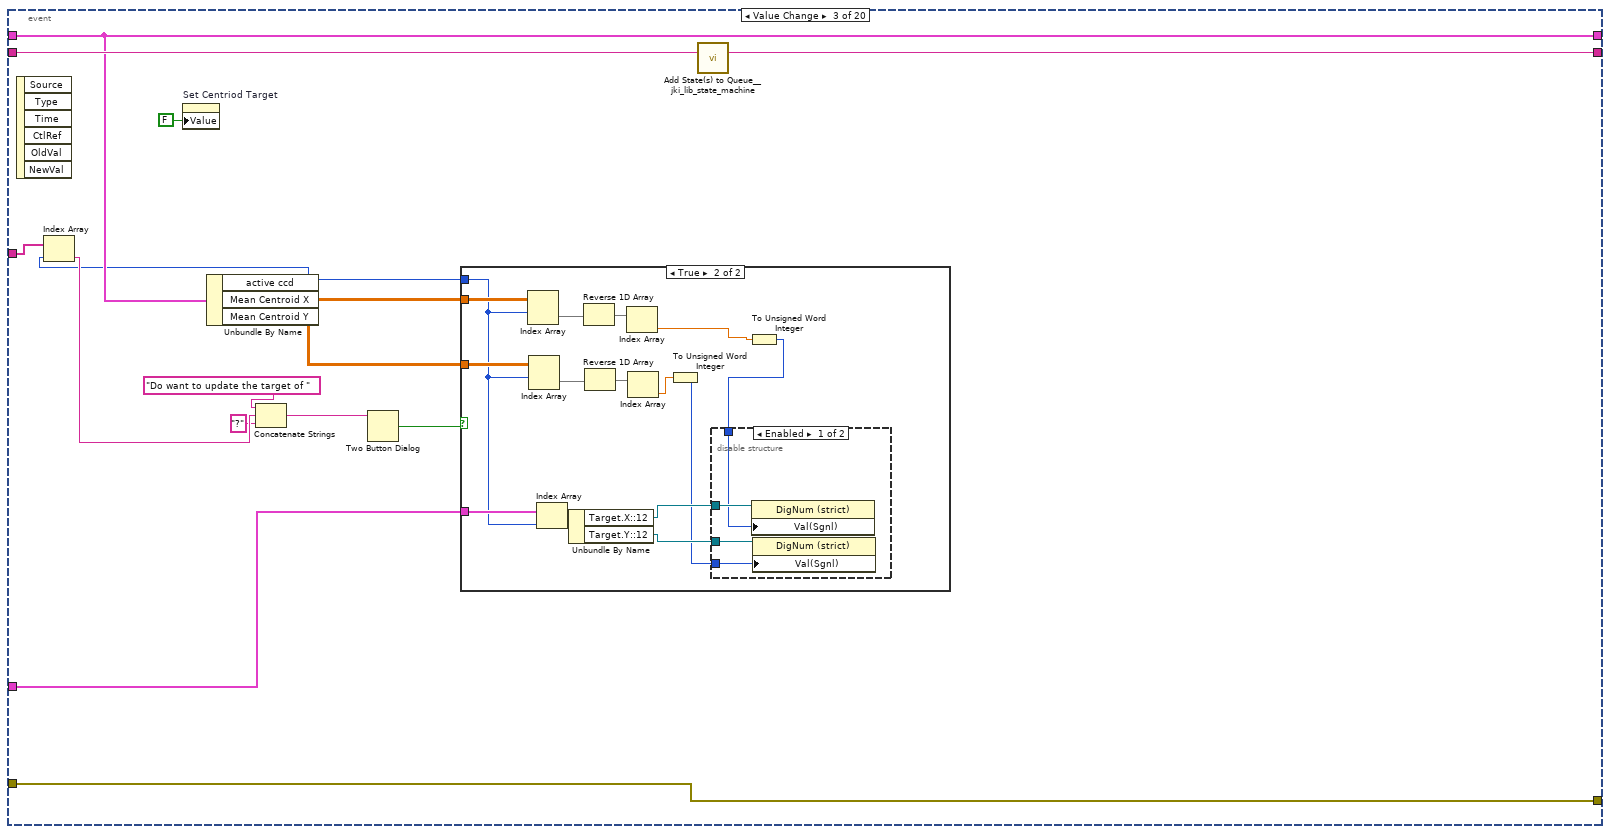
[diagram p9: hidden frame]
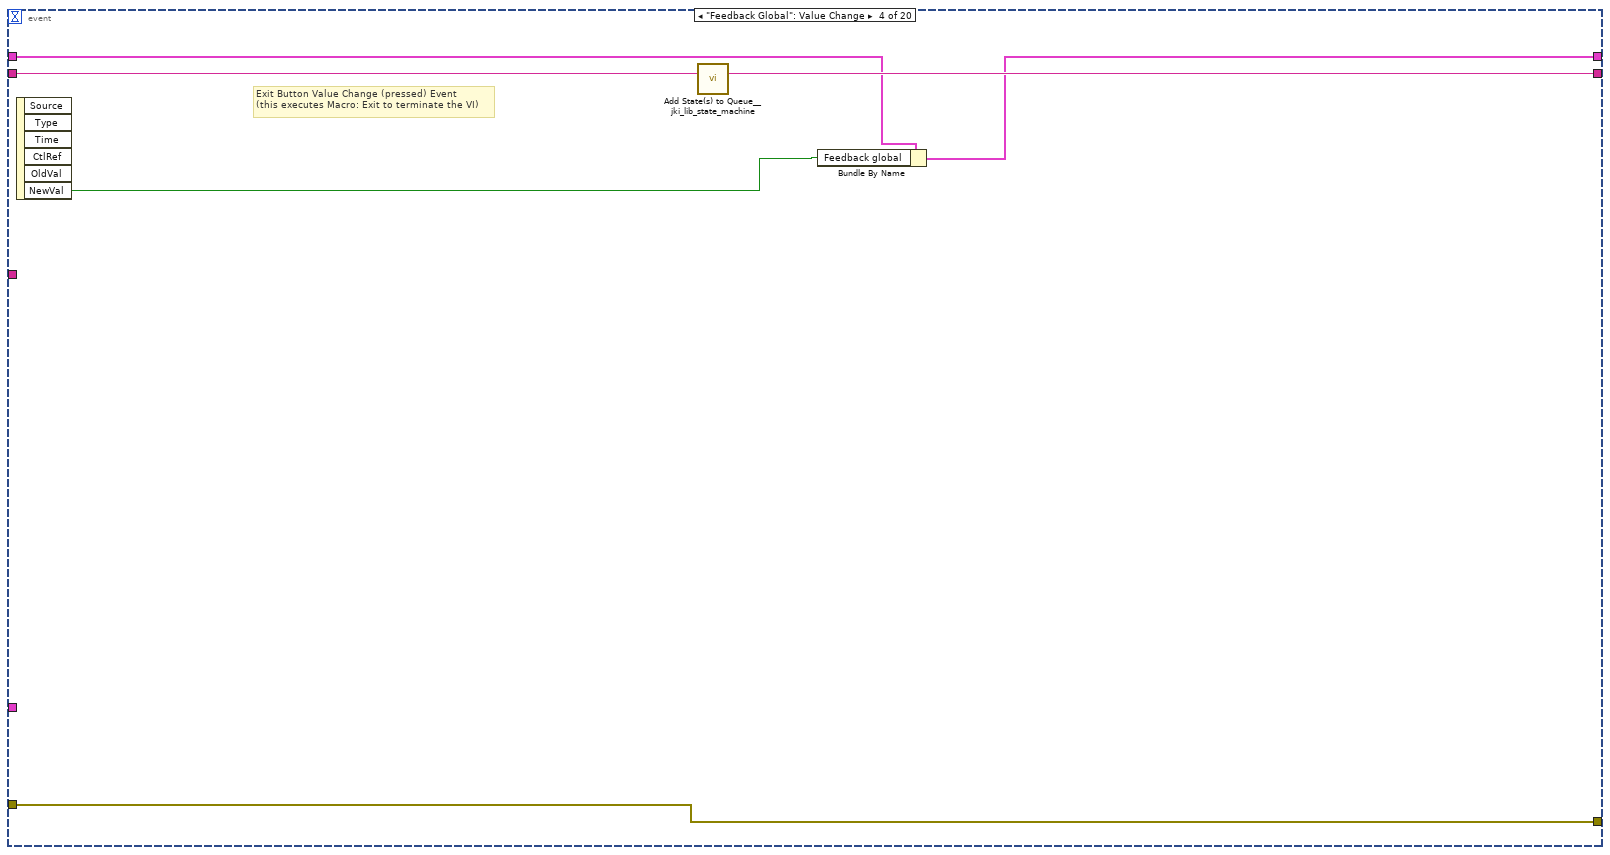
[diagram p12: hidden frame]
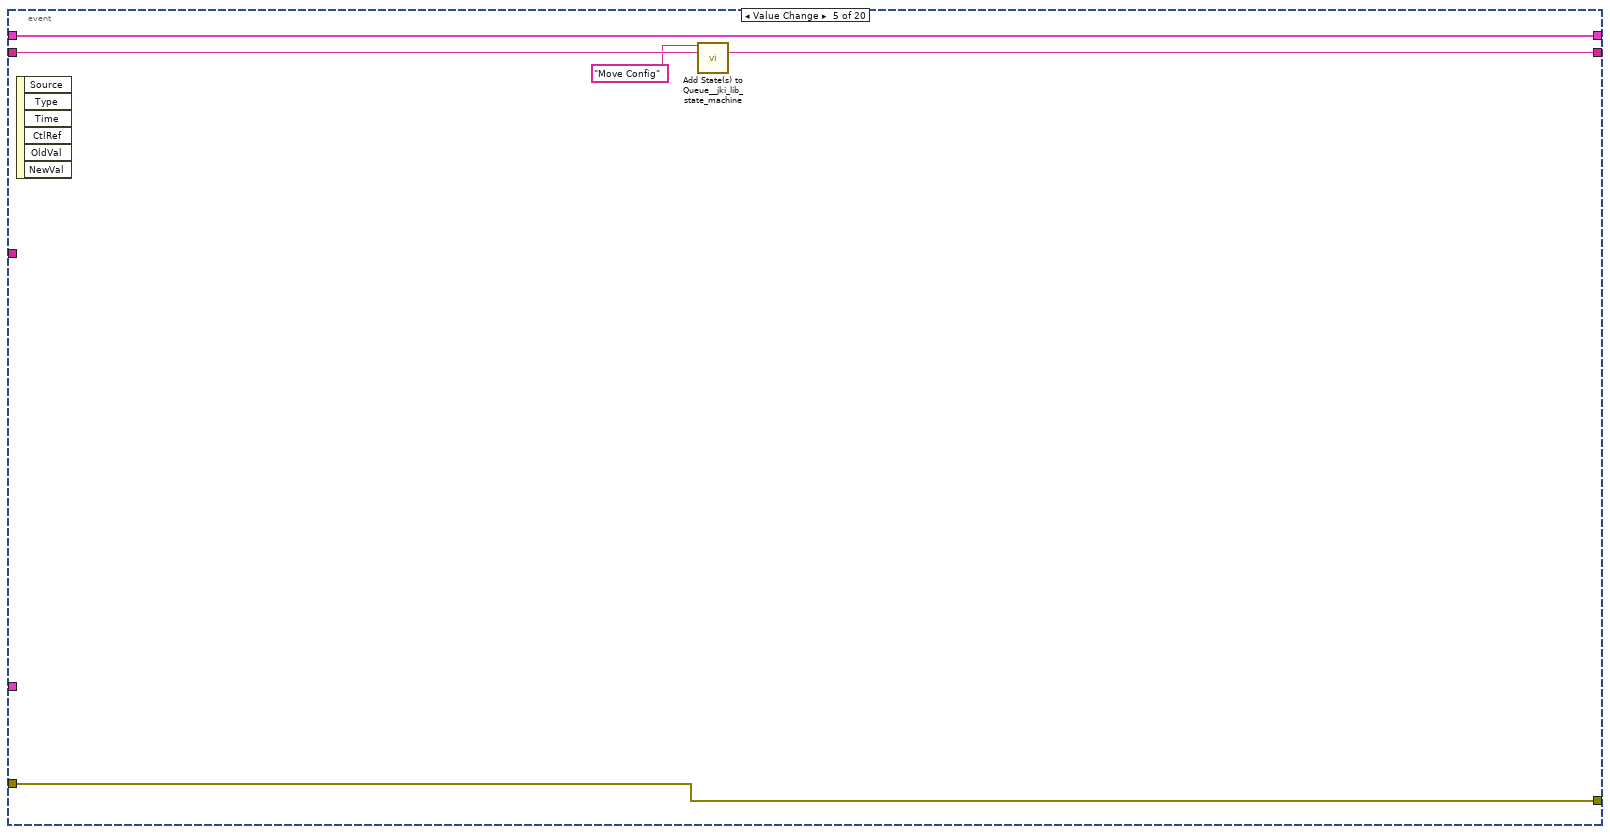
[diagram p13: hidden frame]
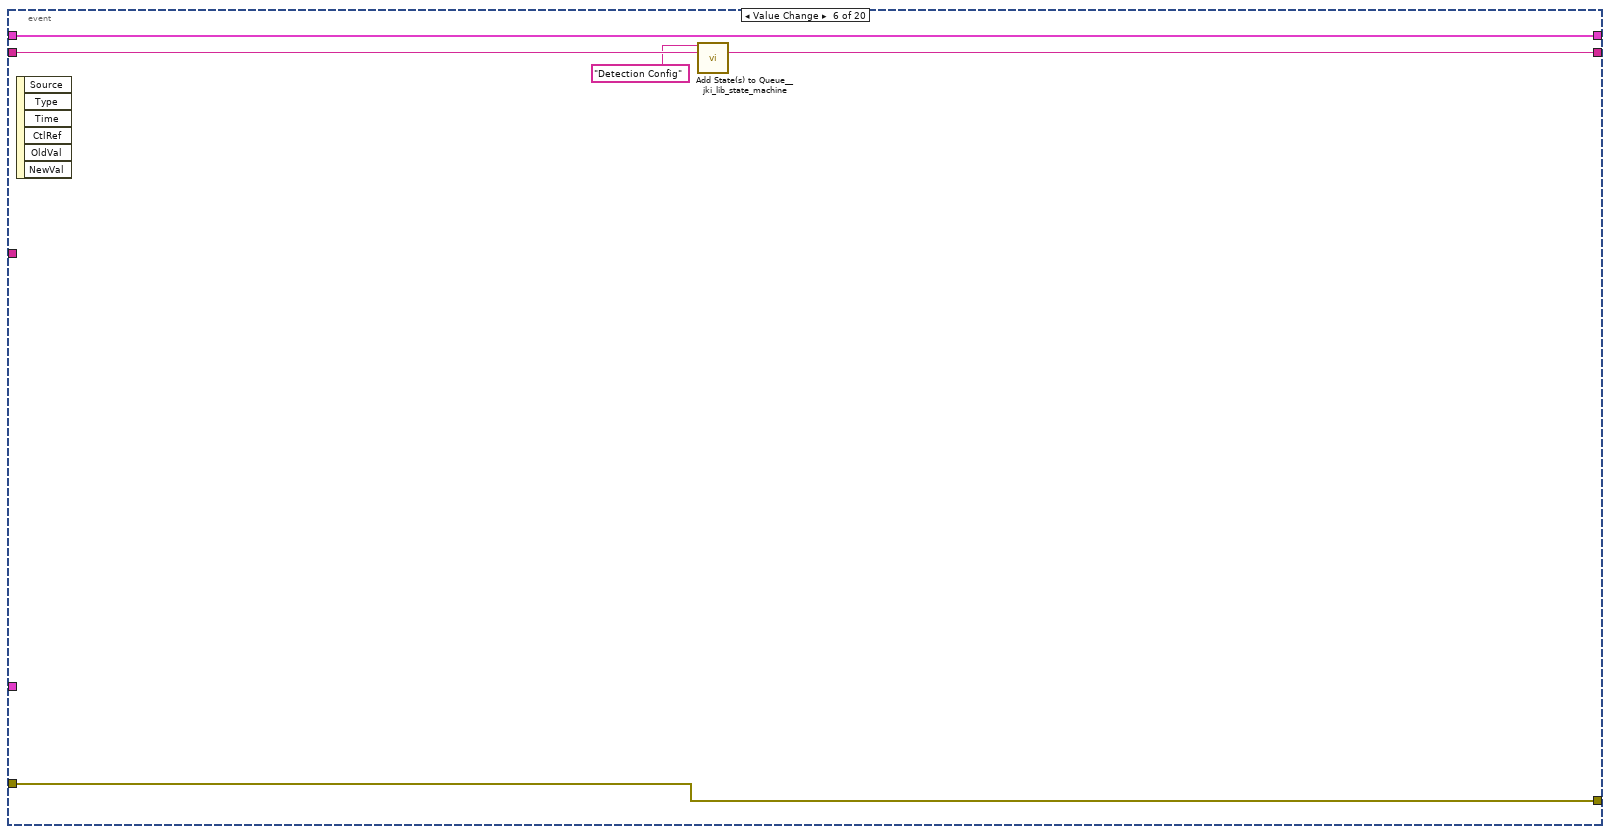
[diagram p14: hidden frame]
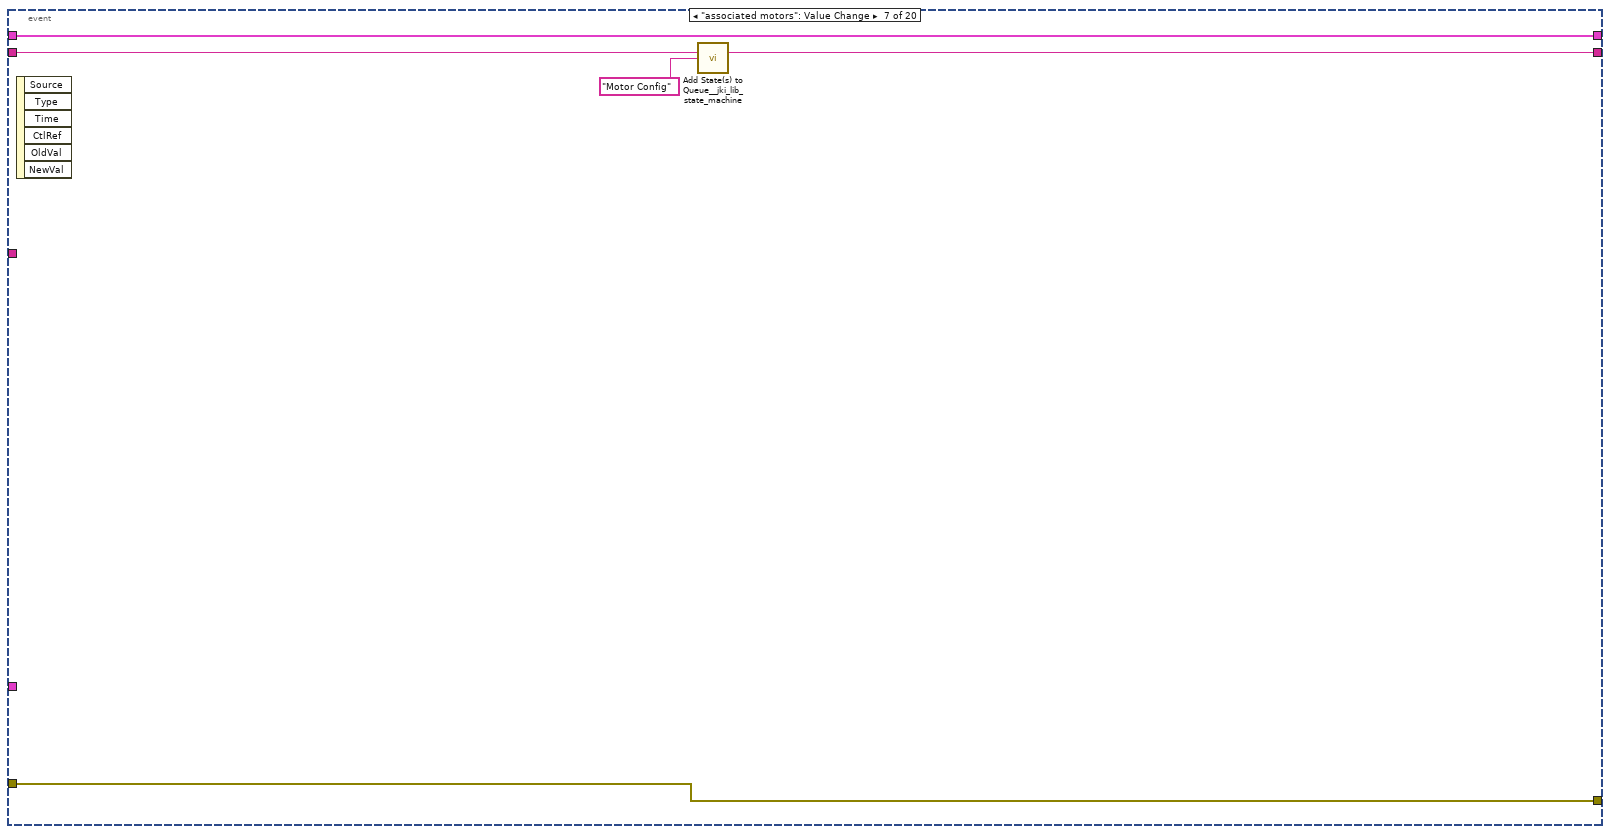
[diagram p15: hidden frame]
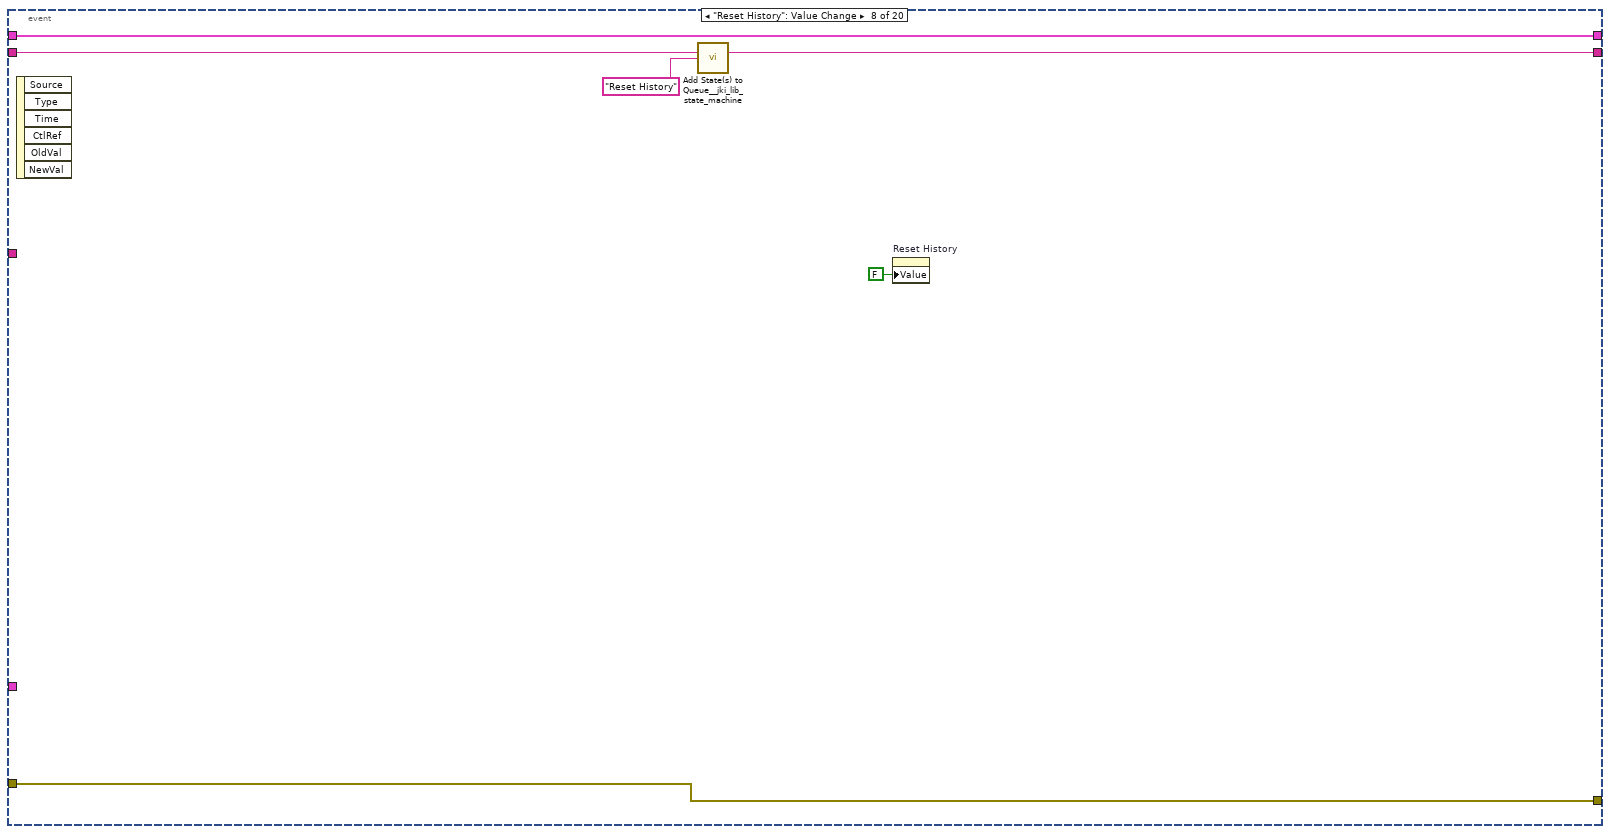
[diagram p16: hidden frame]
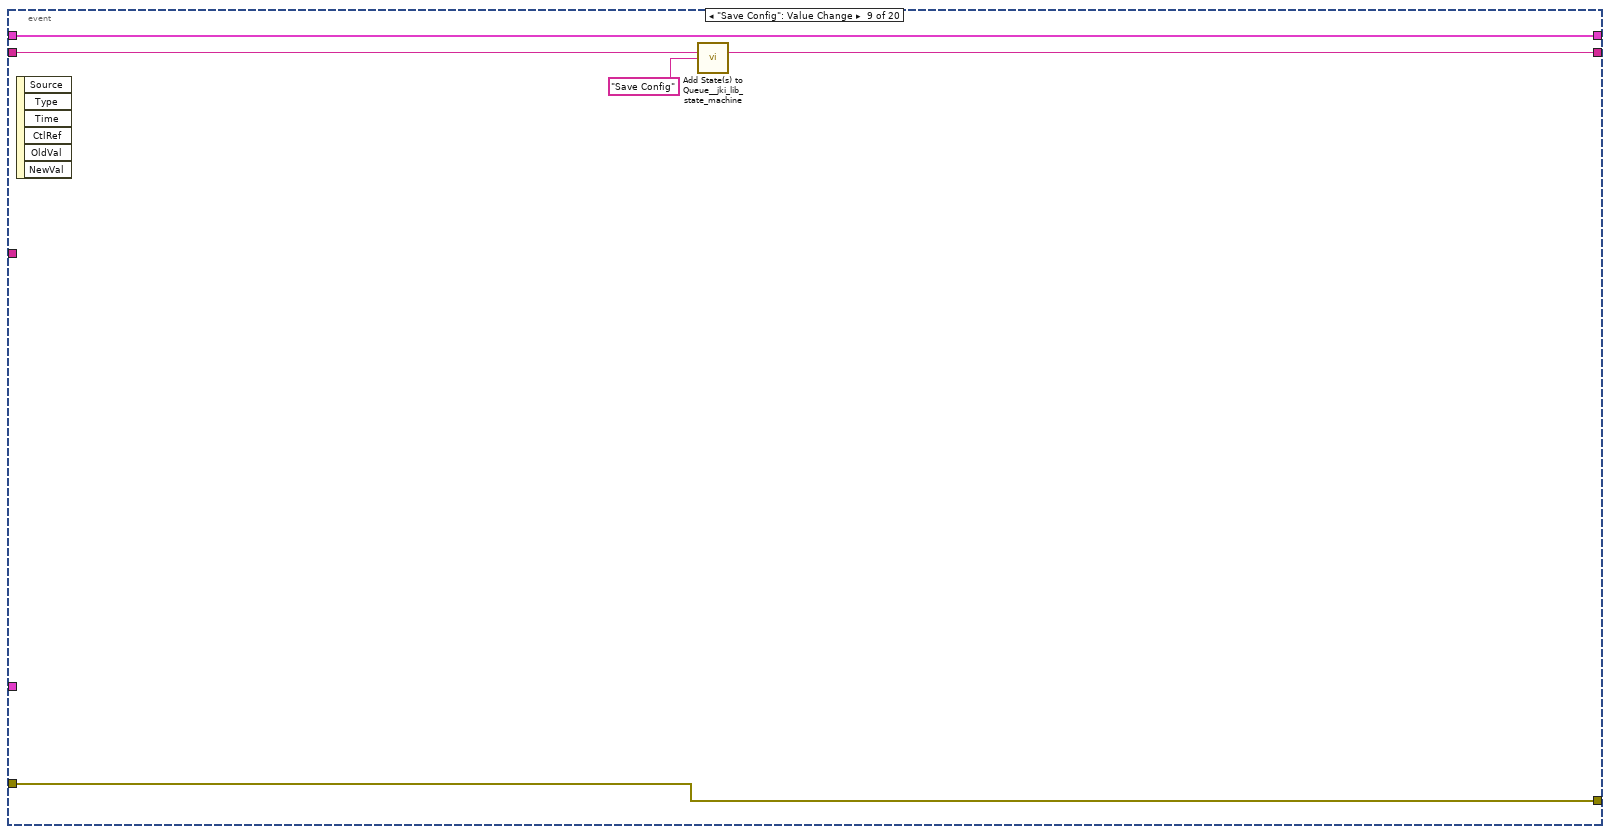
[diagram p17: hidden frame]
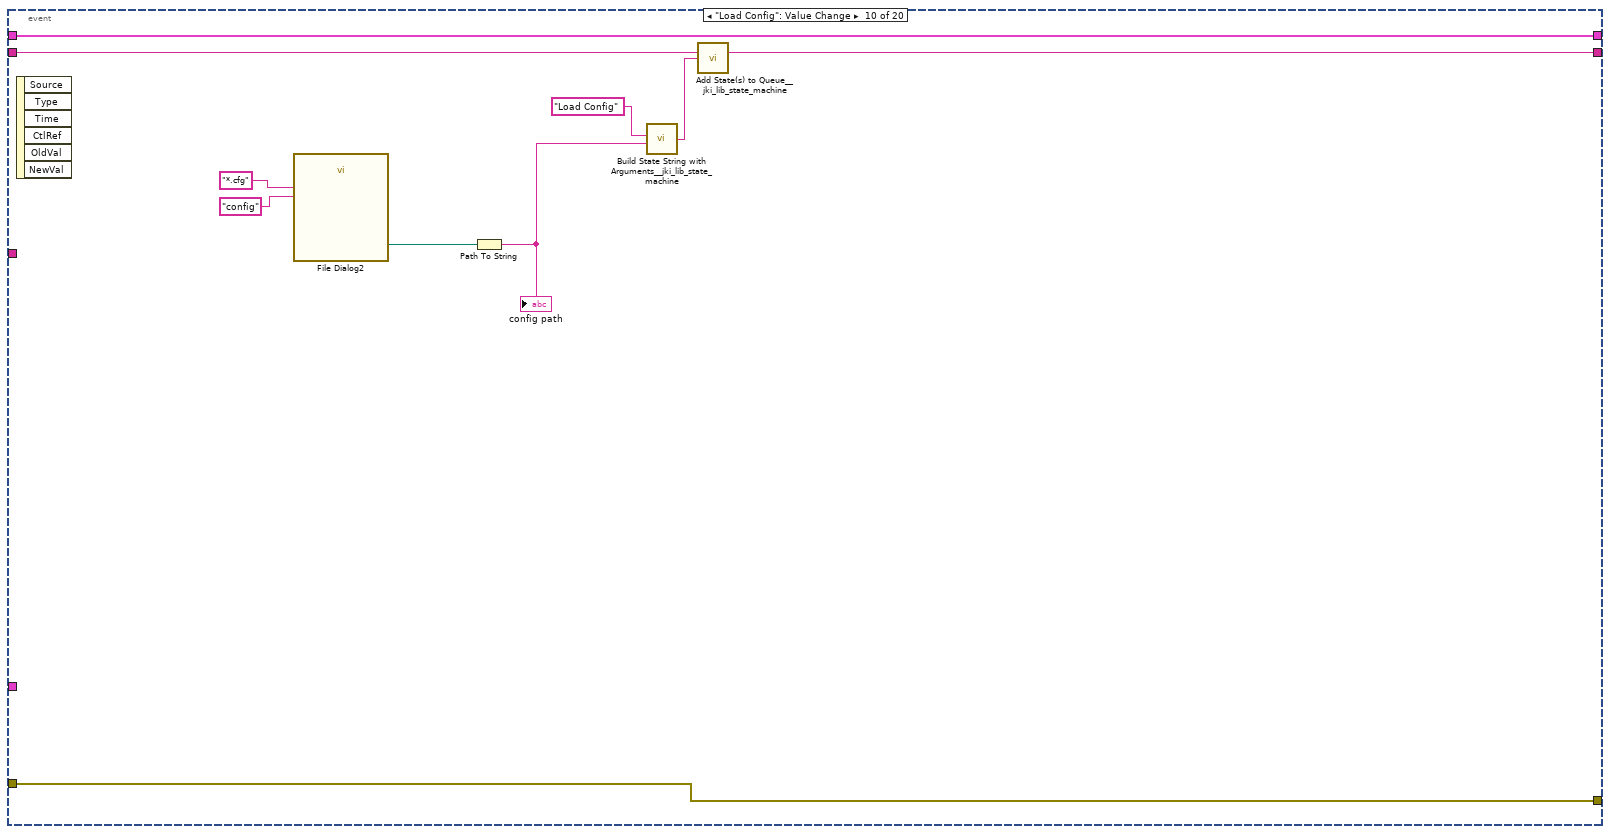
[diagram p18: hidden frame]
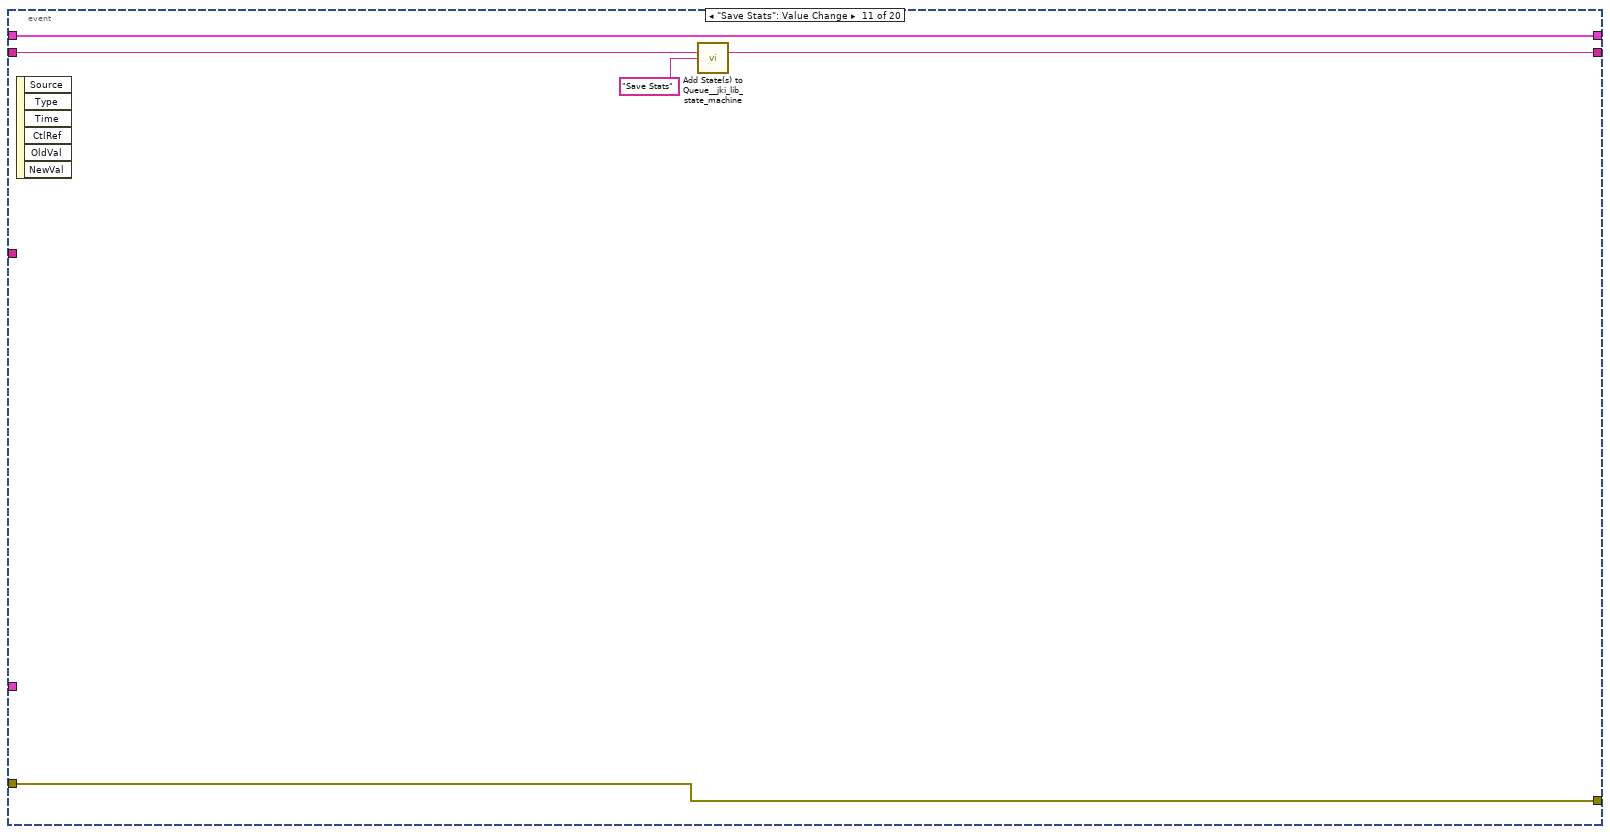
[diagram p19: hidden frame]
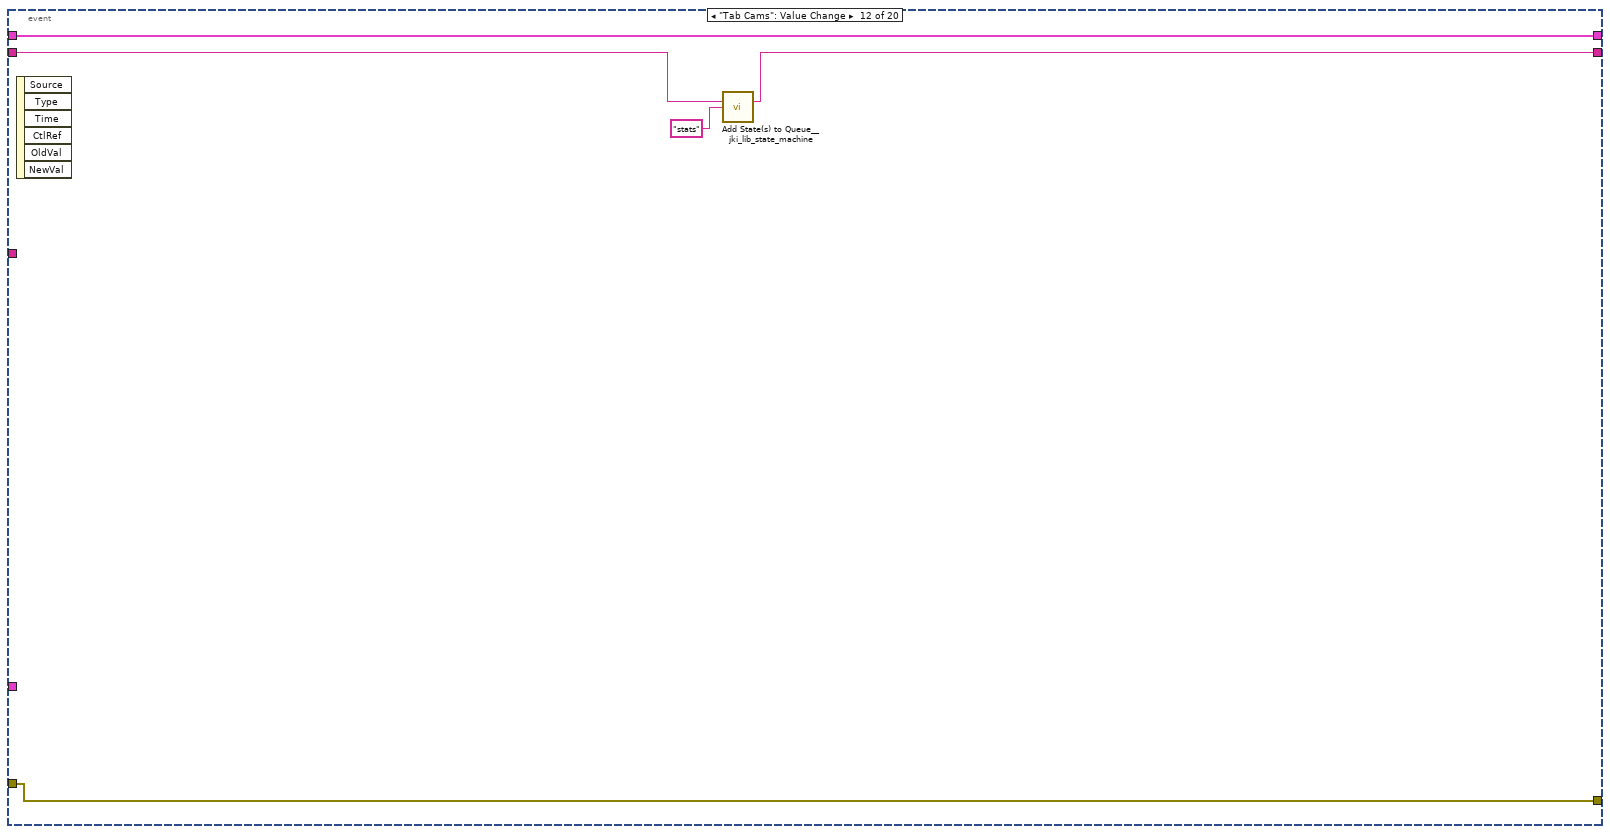
[diagram p20: hidden frame]
diagram:
  n1 = stacked-sequence {
    frame #0 {
      n2 = call <vilib>:"Application Directory.vi"() -> ("Application Directory"=w31:path)
      n3 = Build Path(base path=w31, name or relative path="defaultDevices_ HTU_diode.txt") -> (appended path=w29:path)
      "appended path" <- w29
      n4 = call-poly <vilib>:"Read From Spreadsheet File.vi"("file path (dialog if empty)"=w29) -> ("all rows"=w28:string[][])  [unwired: 6 in, 4 out]
      n5 = Index Array(array=w28, index (col) #1=0 ("disabled index (col)"), index (col) #2=1 ("index (col)")) -> (element #1=w25:string[])  [unwired: 2 in, 1 out]
      n6 = Index Array(array=w25, index #1=0 ("index"), index #2=1 ("index"), index #3=2 ("index"), index #4=3 ("index"), index #5=4 ("index"), index #6=5 ("index"), index #7=6 ("index"), index #8=7 ("index"), index #9=8 ("index"), index #10=9 ("index"), index #11=10 ("index"), index #12=11 ("index")) -> (element #1=w12:string, element #2=w11:string, element #3=w10:string, element #4=w9:string, element #5=w8:string, element #6=w7:string, element #7=w6:string, element #8=w5:string, element #9=w4:string, element #10=w3:string, element #11=w2:string, element #12=w1:string)
      n7 = property on="GUIdevice 1" class="Str"("Val(Sgnl)"=w12) -> ()  [unwired: 2 in, 2 out]
      n8 = property on="GUIdevice 2" class="Str"("Val(Sgnl)"=w11) -> ()  [unwired: 2 in, 2 out]
      n9 = property on="GUIdevice 3" class="Str"("Val(Sgnl)"=w10) -> ()  [unwired: 2 in, 2 out]
      n10 = property on="GUIdevice 4" class="Str"("Val(Sgnl)"=w9) -> ()  [unwired: 2 in, 2 out]
      n11 = property on="GUIdevice 5" class="Str"("Val(Sgnl)"=w8) -> ()  [unwired: 2 in, 2 out]
      n12 = property on="GUIdevice 6" class="Str"("Val(Sgnl)"=w7) -> ()  [unwired: 2 in, 2 out]
      n13 = property on="GUIdevice 7" class="Str"("Val(Sgnl)"=w6) -> ()  [unwired: 2 in, 2 out]
      n14 = property on="GUIdevice 8" class="Str"("Val(Sgnl)"=w5) -> ()  [unwired: 2 in, 2 out]
      n15 = property on="GUIdevice 9" class="Str"("Val(Sgnl)"=w4) -> ()  [unwired: 2 in, 2 out]
      n16 = property on="GUIdevice 10" class="Str"("Val(Sgnl)"=w3) -> ()  [unwired: 2 in, 2 out]
      n17 = property on="GUIdevice 11" class="Str"("Val(Sgnl)"=w2) -> ()  [unwired: 2 in, 2 out]
      n18 = property on="GUIdevice 12" class="Str"("Val(Sgnl)"=w1) -> ()  [unwired: 2 in, 2 out]
    }
    frame #1 {
      w50 = path "c:/BP_DATAsd" ("base path")
      w52 = string[] ["TubeIn", "CompIn", "U_TRA1_56", "BCaveIn", "OAPIn1", "DMIn", "OAPin2", "U_TRA2_34", "Beamline_In"] ("elements")
      w56 = T19 0 items=["Grayscale (U8)", "Grayscale (I16)", "Grayscale (SGL)", "Complex (CSG)", "RGB (U32)", "HSL (U32)", "RGB (U64)", "Grayscale (U16)"] ("Image Type")
      # "NOT FOR YOU MOFO"
      n19 = control-ref of="Position.Axis 1::99"() -> (w125:refnum<vi>)
      n20 = control-ref of="Position.Axis 2::99"() -> (w124:refnum<vi>)
      n21 = control-ref of="Position.Axis 3::99"() -> (w41:refnum<vi>)
      n22 = control-ref of="Position.Axis 4::99"() -> (w40:refnum<vi>)
      n23 = control-ref of="Position.Axis 5::99"() -> (w39:refnum<vi>)
      n24 = control-ref of="Position.Axis 6::99"() -> (w38:refnum<vi>)
      n25 = control-ref of="Position.Axis 1::98"() -> (w49:refnum<vi>)
      n26 = control-ref of="Position.Axis 2::98"() -> (w48:refnum<vi>)
      n27 = control-ref of="Position.Axis 3::98"() -> (w47:refnum<vi>)
      n28 = control-ref of="Position.Axis 4::98"() -> (w37:refnum<vi>)
      n29 = control-ref of="Position.Axis 5::98"() -> (w36:refnum<vi>)
      n30 = control-ref of="Position.Axis 6::98"() -> (w35:refnum<vi>)
      n31 = control-ref of="Position.Axis 1::97"() -> (w46:refnum<vi>)
      n32 = control-ref of="Position.Axis 2::97"() -> (w45:refnum<vi>)
      n33 = control-ref of="Position.Axis 3::97"() -> (w44:refnum<vi>)
      n34 = control-ref of="Position.Axis 4::97"() -> (w34:refnum<vi>)
      n35 = control-ref of="Position.Axis 5::97"() -> (w33:refnum<vi>)
      n36 = control-ref of="Position.Axis 6::97"() -> (w32:refnum<vi>)
      n37 = property on="Motor CCD 1" class="Ring (strict)"("Strings []"=w52) -> ()  [unwired: 2 in, 2 out]
      n38 = property on="Motor CCD 2" class="Ring (strict)"("Strings []"=w52) -> ()  [unwired: 2 in, 2 out]
      n39 = property on="Motor CCD 3" class="Ring (strict)"("Strings []"=w52) -> ()  [unwired: 2 in, 2 out]
      n40 = property on="Motor CCD 4" class="Ring (strict)"("Strings []"=w52) -> ()  [unwired: 2 in, 2 out]
      n41 = property on="Motor CCD 5" class="Ring (strict)"("Strings []"=w52) -> ()  [unwired: 2 in, 2 out]
      n42 = property on="Motor CCD 6" class="Ring (strict)"("Strings []"=w52) -> ()  [unwired: 2 in, 2 out]
      n43 = property on="Motor CCD 7" class="Ring (strict)"("Strings []"=w52) -> ()  [unwired: 2 in, 2 out]
      n44 = property on="Motor CCD 8" class="Ring (strict)"("Strings []"=w52) -> ()  [unwired: 2 in, 2 out]
      n45 = property on="Motor CCD 9" class="Ring (strict)"("Strings []"=w52) -> ()  [unwired: 2 in, 2 out]
      n46 = property on="Motor CCD 10" class="Ring (strict)"("Strings []"=w52) -> ()  [unwired: 2 in, 2 out]
      n47 = property on="Motor CCD 11" class="Ring (strict)"("Strings []"=w52) -> ()  [unwired: 2 in, 2 out]
      n48 = property on="Motor CCD 12" class="Ring (strict)"("Strings []"=w52) -> ()  [unwired: 2 in, 2 out]
      n49 = Build Array(w125, w124, w41, w40, w39, w38, w49, w48, w47, w37, w36, w35, w46, w45, w44, w34, w33, w32) -> (→"motor refs":refnum<vi>[])
      n50 = control-ref of="Target.X::1"() -> (w110:refnum<vi>)
      n51 = control-ref of="Target.Y::1"() -> (w109:refnum<vi>)
      n52 = control-ref of="Target.X::2"() -> (w108:refnum<vi>)
      n53 = control-ref of="Target.Y::2"() -> (w107:refnum<vi>)
      n54 = control-ref of="Target.X::3"() -> (w106:refnum<vi>)
      n55 = control-ref of="Target.Y::3"() -> (w105:refnum<vi>)
      n56 = control-ref of="Target.X::4"() -> (w104:refnum<vi>)
      n57 = control-ref of="Target.Y::4"() -> (w103:refnum<vi>)
      n58 = control-ref of="Target.X::5"() -> (w102:refnum<vi>)
      n59 = control-ref of="Target.Y::5"() -> (w101:refnum<vi>)
      n60 = control-ref of="Target.X::6"() -> (w100:refnum<vi>)
      n61 = control-ref of="Target.Y::6"() -> (w99:refnum<vi>)
      n62 = control-ref of="Target.X::7"() -> (w98:refnum<vi>)
      n63 = control-ref of="Target.Y::7"() -> (w97:refnum<vi>)
      n64 = control-ref of="Target.X::8"() -> (w96:refnum<vi>)
      n65 = control-ref of="Target.Y::8"() -> (w95:refnum<vi>)
      n66 = control-ref of="Target.X::9"() -> (w73:refnum<vi>)
      n67 = control-ref of="Target.Y::9"() -> (w72:refnum<vi>)
      n68 = control-ref of="Target.X::10"() -> (w71:refnum<vi>)
      n69 = control-ref of="Target.Y::10"() -> (w70:refnum<vi>)
      n70 = control-ref of="Target.X::11"() -> (w69:refnum<vi>)
      n71 = control-ref of="Target.Y::11"() -> (w68:refnum<vi>)
      n72 = control-ref of="Target.X::12"() -> (w67:refnum<vi>)
      n73 = control-ref of="Target.Y::12"() -> (w66:refnum<vi>)
      n74 = call "IMAQ Create"("Image Name"="GUIdevice 8", "Image Type"=w56) -> ("New Image"=→"image::8":T9)  [unwired: 3 in, 1 out]
      n75 = call "IMAQ Create"("Image Name"="GUIdevice 9", "Image Type"=w56) -> ("New Image"=→"image::9":T9)  [unwired: 3 in, 1 out]
      n76 = call "IMAQ Create"("Image Name"="GUIdevice 10", "Image Type"=w56) -> ("New Image"=→"image::10":T9)  [unwired: 3 in, 1 out]
      n77 = call "IMAQ Create"("Image Name"="GUIdevice 6", "Image Type"=w56) -> ("New Image"=→"image::6":T9)  [unwired: 3 in, 1 out]
      n78 = call "IMAQ Create"("Image Name"="GUIdevice 7", "Image Type"=w56) -> ("New Image"=→"image::7":T9)  [unwired: 3 in, 1 out]
      n79 = call "IMAQ Create"("Image Name"="GUIdevice 11", "Image Type"=w56) -> ("New Image"=→"image::11":T9)  [unwired: 3 in, 1 out]
      n80 = call "IMAQ Create"("Image Name"="GUIdevice 12", "Image Type"=w56) -> ("New Image"=→"image::12":T9)  [unwired: 3 in, 1 out]
      n81 = call "IMAQ Create"("Image Name"="GUIdevice 2") -> ("New Image"=→"image::2":T9)  [unwired: 4 in, 1 out]
      n82 = call "IMAQ Create"("Image Name"="GUIdevice 4", "Image Type"=w56) -> ("New Image"=→"image::4":T9)  [unwired: 3 in, 1 out]
      n83 = call "IMAQ Create"("Image Name"="GUIdevice 1", "Image Type"=w56) -> ("New Image"=→"image::1":T9)  [unwired: 3 in, 1 out]
      n84 = call "IMAQ Create"("Image Name"="GUIdevice 3", "Image Type"=w56) -> ("New Image"=→"image::3":T9)  [unwired: 3 in, 1 out]
      n85 = call "IMAQ Create"("Image Name"="GUIdevice 5", "Image Type"=w56) -> ("New Image"=→"image::5":T9)  [unwired: 3 in, 1 out]
      n86 = Build Array("GUIdevice 1", "GUIdevice 2", "GUIdevice 3", "GUIdevice 4", "GUIdevice 5", "GUIdevice 6", "GUIdevice 7", "GUIdevice 8", "GUIdevice 9", "GUIdevice 10", "GUIdevice 11", "GUIdevice 12") -> (w84:string[])
      "CCDs" <- w84
      n87 = property on="image::8" class="ImageControl"("Caption.Text"="GUIdevice 8") -> ()  [unwired: 2 in, 2 out]
      n88 = property on="image::10" class="ImageControl"("Caption.Text"="GUIdevice 10") -> ()  [unwired: 2 in, 2 out]
      n89 = property on="image::9" class="ImageControl"("Caption.Text"="GUIdevice 9") -> ()  [unwired: 2 in, 2 out]
      n90 = property on="image::1" class="ImageControl"("Caption.Text"="GUIdevice 1") -> ()  [unwired: 2 in, 2 out]
      n91 = property on="image::2" class="ImageControl"("Caption.Text"="GUIdevice 2") -> ()  [unwired: 2 in, 2 out]
      n92 = property on="image::3" class="ImageControl"("Caption.Text"="GUIdevice 3") -> ()  [unwired: 2 in, 2 out]
      n93 = property on="image::4" class="ImageControl"("Caption.Text"="GUIdevice 4") -> ()  [unwired: 2 in, 2 out]
      n94 = property on="image::5" class="ImageControl"("Caption.Text"="GUIdevice 5") -> ()  [unwired: 2 in, 2 out]
      n95 = property on="image::6" class="ImageControl"("Caption.Text"="GUIdevice 6") -> ()  [unwired: 2 in, 2 out]
      n96 = property on="image::7" class="ImageControl"("Caption.Text"="GUIdevice 7") -> ()  [unwired: 2 in, 2 out]
      n97 = property on="image::11" class="ImageControl"("Caption.Text"="GUIdevice 11") -> ()  [unwired: 2 in, 2 out]
      n98 = property on="image::12" class="ImageControl"("Caption.Text"="GUIdevice 12") -> ()  [unwired: 2 in, 2 out]
      n99 = Array To Cluster(array=w84) -> (cluster=→"Cameras":T20)
      n100 = Bundle("Target.X::1"=w110, "Target.Y::1"=w109) -> (w94:T21)  [unwired: 1 in]
      n101 = Bundle("Target.X::2"=w108, "Target.Y::2"=w107) -> (w93:T22)  [unwired: 1 in]
      n102 = Bundle("Target.X::3"=w106, "Target.Y::3"=w105) -> (w92:T23)  [unwired: 1 in]
      n103 = Bundle("Target.X::4"=w104, "Target.Y::4"=w103) -> (w85:T24)  [unwired: 1 in]
      n104 = Bundle("Target.X::5"=w102, "Target.Y::5"=w101) -> (w91:T25)  [unwired: 1 in]
      n105 = Bundle("Target.X::6"=w100, "Target.Y::6"=w99) -> (w90:T26)  [unwired: 1 in]
      n106 = Bundle("Target.X::7"=w98, "Target.Y::7"=w97) -> (w89:T27)  [unwired: 1 in]
      n107 = Bundle("Target.X::8"=w96, "Target.Y::8"=w95) -> (w88:T28)  [unwired: 1 in]
      n108 = Bundle("Target.X::12"=w67, "Target.Y::12"=w66) -> (w62:T29)  [unwired: 1 in]
      n109 = Bundle("Target.X::9"=w73, "Target.Y::9"=w72) -> (w65:T30)  [unwired: 1 in]
      n110 = Bundle("Target.X::10"=w71, "Target.Y::10"=w70) -> (w64:T31)  [unwired: 1 in]
      n111 = Bundle("Target.X::11"=w69, "Target.Y::11"=w68) -> (w63:T32)  [unwired: 1 in]
      n112 = property on="CCDs" class="Ring (strict)"("Strings []"=w84) -> ()  [unwired: 2 in, 2 out]
      n113 = Build Array(w94, w93, w92, w85, w91, w90, w89, w88, w65, w64, w63, w62) -> (w87:T33)
      n114 = Tick Count (ms)() -> (millisecond timer value=→"millisecond timer value":u32)
      n115 = Get Date/Time In Seconds() -> (seconds since 1Jan1904=w75:timestamp)
      n116 = property on="Feedback Global" class="Bool (strict)"("Value"=FALSE ("Feedback Global")) -> ()  [unwired: 2 in, 2 out]
      n117 = Format Date/Time String(time format string (%c)="%Y%m%d%H%M", seconds (now)=w75) -> (date/time string=w74:string)  [unwired: 1 in]
      n118 = Concatenate Strings(w74, "Beampointing_HTU_diode.tdms" ("string")) -> (w78:string)
      n119 = String To Path(string=w78) -> (path=w77:path)
      n120 = Build Path(base path=w50, name or relative path=w77) -> (appended path=w80:path)
      n121 = call <vilib>:"Add State(s) to Queue__jki_lib_state_machine.vi"("State(s) in (\"\")"="Macro: Initialize") -> ("States Out"=w127:string)  [unwired: 14 in]
      n122 = Create User Event(user event datatype=T13 {"EventEnum"=enum."new data", "Device name"="Device name"} ("New Event")) -> (user event=w135:refnum<user-event>, error out=w137:errorcluster)  [unwired: 1 in]
      "tcp data event" <- w135
      n123 = while "JKI - String-Based Queued State Machine (Basic) v1.0" {
        shift-right: [w158] -> w83
        shift-left: _ -> [w151]
        shift-right: [w161] -> w111
        shift-left: _ -> [w157]
        shift-right: [w160] -> _
        shift-left: w127 -> [w162]
        tunnel: w87 -> [w155]
        tunnel: w84 -> [w153]
        tunnel: [w153] -> w112
        tunnel: w87 -> [w154]
        tunnel: w80 -> [w149]
        tunnel: w50 -> [w148]
        stop <- w159 stop-if-true
        n124 = Unbundle By Name(w151) -> ("active cams"=w150:string[], "Mean Centroid X"=w147:dbl[][], "Mean Centroid Y"=w146:dbl[][], "Mean Size"=w145:dbl[][])
        n125 = call <vilib>:"Parse State Queue__jki_lib_state_machine.vi"("State Queue"=w162, "Error In (no error)"=w157) -> ("Remaining States"=w164:string, "Current State"=w165:string, "Arguments"=w163:string)  [unwired: 11 in]
        "Current State" <- w165
        n126 = case shown="\"Device Ini\"" w165 {
          selector: w165 -> [_ _ w513 _ _ _ _ _ _ _ _ _ _ _ _ _ _ _ _ _ _ _ _ _ _ _ _ _ _ _ _ _ _ _ _ _ _ _ _ _ _ _]
          tunnel: w164 -> [w230 w512 w517 w535 w541 w546 w550 w591 w607 w611 w615 w621 w632 w656 w665 w675 w679 w707 w828 w880 w910 w919 w941 w962 w966 w985 w1130 w1298 w1378 w1442 w1517 w1593 w1617 w1632 w1706 w1758 w1768 w1808 w1903 w1929 w1943 w1966]
          tunnel: w163 -> [_ _ _ _ _ _ _ _ _ _ _ w616 w627 _ _ _ _ w683 w781 _ w895 _ _ _ _ w986 _ w1278 w1364 w1428 w1497 w1587 _ _ _ _ _ _ _ _ w1947 _]
          tunnel: w151 -> [w228 w509 w515 w525 w538 w544 w547 _ w602 w608 w613 w619 w626 w653 w662 w667 w676 w698 w818 w878 w891 w915 w933 w955 w963 w974 w1113 w1274 w1374 w1438 w1488 w1589 w1614 w1629 w1702 w1755 w1765 w1782 w1901 w1926 w1946 w1957]
          tunnel: [w227 w510 w519 w533 errorcluster {"status"=FALSE, "code"=0, "source"=""} ("error out") w543 w548 w558 w604 w609 w612 w617 w629 w654 w663 w673 w677 w701 w784 w869 w899 w917 w939 w960 w964 w1015 w1143 w1296 w1376 w1440 w1515 w1582 w1615 w1630 w1703 w1756 w1766 w1775 w1865 w1927 w1941 w1964] -> w161
          tunnel: w157 -> [w226 w510 w518 w533 w537 w543 w548 w559 w605 w609 w612 w618 w630 w654 w663 w673 w677 w702 w782 w870 w898 w917 w939 w960 w964 w1015 w1143 w1296 w1376 w1440 w1515 w1583 w1615 w1630 w1704 w1756 w1766 w1776 w1899 w1927 w1941 w1964]
          tunnel: [w229 w511 w516 w534 w540 w545 w549 w590 w606 w610 w614 w620 w631 w655 w664 w674 w678 w692 w827 w879 w909 w918 w940 w961 w965 w968 w1144 w1297 w1377 w1441 w1516 w1592 w1616 w1631 w1705 w1757 w1767 w1807 w1902 w1928 w1942 w1965] -> w160
          tunnel: [_ _ _ _ _ TRUE _ _ _ _ _ _ _ _ _ _ _ _ _ _ _ _ _ _ _ _ _ _ _ _ _ _ _ _ _ _ _ _ _ _ _ _] -> w159
          tunnel: [w223 w509 w515 w524 w538 w544 w547 w560 w602 w608 w613 w619 w626 w653 w662 w667 w676 w704 w817 w878 w904 w914 w932 w954 w963 w967 w1114 w1274 w1374 w1438 w1488 w1591 w1614 w1629 w1702 w1754 w1765 w1782 w1900 w1926 w1945 w1956] -> w158
          tunnel: "update speed [ms]" -> [w225 _ _ _ _ _ _ _ _ _ _ _ _ _ _ _ _ _ _ _ _ _ _ _ _ _ _ _ _ _ _ _ _ _ _ _ _ _ _ _ _ _]
          tunnel: w155 -> [w222 _ _ _ _ _ _ _ _ _ _ _ _ _ _ _ _ _ _ _ _ _ _ _ _ w1007 _ _ _ _ _ _ _ _ _ _ _ _ _ w1911 _ _]
          tunnel: w153 -> [w224 _ _ _ _ _ _ w555 _ _ _ _ _ _ _ _ _ w706 w816 _ w905 _ _ _ _ w978 w1115 w1295 _ _ w1514 w1588 _ w1619 _ _ _ w1781 _ _ _ _]
          tunnel: w149 -> [_ _ _ _ _ _ _ w557 _ _ _ _ _ _ _ _ _ w703 _ _ _ _ _ _ _ _ _ _ _ _ _ _ _ _ _ _ _ _ _ _ _ _]
          tunnel: w148 -> [_ _ _ _ _ _ _ _ _ _ _ _ _ _ _ _ _ _ _ _ _ _ _ _ _ _ _ _ _ _ _ _ _ _ _ _ _ _ w1871 _ _ _]
          frame "", "Idle" {
            # "executes when the state queue is empty"
            n127 = event shown="[0] Timeout" {
              selector: _ -> [_ _ _ _ _ _ _ _ _ _ _ _ _ _ _ _ _ _ _ _]
              dyn-events: _ -> [_ _ _ _ _ _ _ _ _ _ _ _ _ _ _ _ _ _ _ _]
              timeout: w225 -> [_ _ _ _ _ _ _ _ _ _ _ _ _ _ _ _ _ _ _ _]
              tunnel: w230 -> [w235 w359 w374 w399 w404 w409 w414 w420 w425 w435 w440 w442 w454 w466 w478 w483 w488 w494 w498 w508]
              tunnel: [w260 w358 w373 w398 w403 w408 w413 w419 w424 w434 w439 w441 w453 w465 w477 w482 w487 w493 w497 w507] -> w229
              tunnel: w228 -> [w256 w356 w370 w395 w401 w406 w411 w417 w422 w432 w437 w445 w447 w464 w476 w481 w486 w492 w499 w505]
              tunnel: [w271 w357 w372 w397 w402 w407 w412 w418 w423 w433 w438 w444 w452 w459 w471 w480 w485 w491 w496 w506] -> w227
              tunnel: w226 -> [w247 w357 w372 w397 w402 w407 w412 w418 w423 w433 w438 w444 w452 w460 w472 w480 w485 w491 w496 w506]
              tunnel: [w259 w356 w370 w394 w401 w406 w411 w417 w422 w432 w437 w445 w447 w464 w476 w481 w486 w492 w499 w505] -> w223
              tunnel: w224 -> [w252 _ w366 _ _ _ _ _ _ _ _ _ _ _ _ _ _ _ _ _]
              tunnel: w222 -> [_ _ w368 _ _ _ _ _ _ _ _ _ _ _ _ _ _ _ _ _]
              event Timeout {
                n128 = event-data() -> ()  [unwired: 1 in, 1 out]
                n129 = Unbundle By Name(w256) -> ("Centroid X"=w253:dbl[][], "Centroid Y"=w250:dbl[][], "Size"=w248:dbl[][], "detection para"=w243:T3[], "active cams"=w251:string[], "thresholds"=w249:cluster{"Lower value":sgl, "Upper value":sgl}[])
                n130 = Unbundle By Name(w256) -> ("img to avg"=w232:i32, "active ccd"=w255:i32)
                n131 = for {
                  tunnel: w251 -> [w292] mode=indexing
                  tunnel: [w293] -> w239 mode=indexing
                  tunnel: w252 -> [w315]
                  tunnel: w243 -> [w313]
                  tunnel: [w276] -> w238 mode=indexing
                  tunnel: [w311] -> w246 mode=indexing
                  tunnel: [w309] -> w254 mode=indexing
                  tunnel: "autodetect" -> [w303]
                  tunnel: w247 -> [w316]
                  tunnel: [w317] -> w245
                  shift-right: [w300] -> w242
                  shift-left: w249 -> [w302]
                  shift-right: [w287] -> w231
                  shift-left: w253 -> [w289]
                  shift-right: [w283] -> w241
                  shift-left: w250 -> [w285]
                  shift-right: [w277] -> w240
                  shift-left: w248 -> [w279]
                  w281 = 0 ("index")
                  n132 = call-poly <userlib>:"Filter 1D Array__ogtk.vi"("items to filter"=w292, "array"=w315) -> ("filtered item indices"=w314:i32[])  [unwired: 4 in, 1 out]
                  n133 = Index Array(array=w314) -> (element=w278:i32)  [unwired: 1 in]
                  n134 = Index Array(array=w279, index (row)=w278) -> (element=w307:dbl[])  [unwired: 1 in]
                  n135 = Index Array(array=w285, index (row)=w278) -> (element=w308:dbl[])  [unwired: 1 in]
                  n136 = Index Array(array=w302, index=w278) -> (element=w306:cluster{"Lower value":sgl, "Upper value":sgl})
                  n137 = Index Array(array=w289, index (row)=w278) -> (element=w291:dbl[])  [unwired: 1 in]
                  n138 = Index Array(array=w313, index=w278) -> (element=w310:T3)
                  n139 = call "CENTRIOD DETECTION.vi"("Refnum in"=w292, "auto threshold"=w303, "Threshold Range In"=w306, "beam detection para"=w310, "error in (no error)"=w316) -> ("Bounding Rect"=w309:T34, "Particle Reports (Pixels)"=w311:T1, "Threshold Range Out"=w301:cluster{"Lower value":sgl, "Upper value":sgl}, "Centriod"=w318:cluster{"X":dbl, "Y":dbl}, "error out"=w317:errorcluster)  [unwired: 7 in, 3 out]
                  n140 = Unbundle By Name(w318) -> ("X"=w290:dbl, "Y"=w286:dbl)
                  n141 = Empty Array?(array=w311) -> (empty?=w312:bool)
                  n142 = Not(x=w312) -> (.not. x?=w276:bool)
                  n143 = Replace Array Subset(array=w302, new element=w301, index=w278) -> (w300:cluster{"Lower value":sgl, "Upper value":sgl}[])
                  n144 = Unbundle By Name(w309) -> ("Right"=w299:dbl, "Left"=w298:dbl, "Bottom"=w297:dbl, "Top"=w296:dbl)
                  n145 = Subtract(x=w299, y=w298) -> (x-y=w294:dbl)
                  n146 = Subtract(x=w297, y=w296) -> (x-y=w295:dbl)
                  n147 = Multiply(x=w294, y=w295) -> (x*y=w282:dbl)
                  n148 = Insert Into Array(array=w308, index=w281, new element=w286) -> (w284:dbl[])
                  n149 = Insert Into Array(array=w291, index=w281, new element=w290) -> (w288:dbl[])
                  n150 = Insert Into Array(array=w307, index=w281, new element=w282) -> (w280:dbl[])
                  n151 = for {
                    shift-right: [w319] -> w304
                    shift-left: dbl[] [] ("Array 4") -> [w322]
                    tunnel: w284 -> [w320] mode=indexing
                    n152 = Equal To 0?(x=w320) -> (x = 0?=w321:bool)
                    n153 = case shown="False" w321 {
                      tunnel: w322 -> [w325 w326]
                      tunnel: w320 -> [w324 _]
                      tunnel: [w323 w326] -> w319
                      frame False {
                        n154 = Build Array (concatenate)(w325, w324) -> (w323:dbl[])
                      }
                      frame True {
                      }
                    }
                  }
                  n155 = Replace Array Subset(array=w289, new element=w288, index (row)=w278) -> (w287:dbl[][])  [unwired: 1 in]
                  n156 = Replace Array Subset(array=w285, new element=w284, index (row)=w278) -> (w283:dbl[][])  [unwired: 1 in]
                  n157 = Replace Array Subset(array=w279, new element=w280, index (row)=w278) -> (w277:dbl[][])  [unwired: 1 in]
                  n158 = Array Size(array=w304) -> (size(s)=w293:i32)
                }
                "detected" <- w238
                "Box" <- w254
                n159 = Index Array(array=w246, index (row)=w255) -> (element=→"particles":T1)  [unwired: 1 in]
                n160 = call <vilib>:"Clear Errors.vi"("error in (no error)"=w245) -> ("error out"=w271:errorcluster)  [unwired: 6 in]
                n161 = local read "Numeric"() -> (w264:dbl)
                n162 = Increment(x=w232) -> (x+1=w261:i32)
                n163 = Greater Or Equal?(x=w264, y=w261) -> (x >= y?=w258:bool)
                n164 = Increment(x=w264) -> (x+1=w263:dbl)
                n165 = Select(t=0.0, s=w258, f=w263) -> (s? t:f=w262:dbl)
                n166 = local write "Numeric"(w262) -> ()
                n167 = Bundle By Name(cluster=w256, "thresholds"=w242) -> (w267:T35)
                n168 = for {
                  tunnel: w239 -> [w348] mode=indexing
                  tunnel: w251 -> [w354] mode=indexing
                  shift-right: [w349] -> w272
                  shift-left: "" ("GUIdevice 7") -> [w352]
                  tunnel: [w343] -> w274 mode=indexing
                  tunnel: "Detection Rate" -> [w347]
                  tunnel: w262 -> [w345]
                  tunnel: w232 -> [w341]
                  n169 = Greater Or Equal?(x=w348, y=w341) -> (x >= y?=w344:bool)
                  n170 = Multiply(x=w347, y=w345) -> (x*y=w346:dbl)
                  n171 = Greater Or Equal?(x=w348, y=w346) -> (x >= y?=w342:bool)
                  n172 = And(x=w344, y=w342) -> (x .and. y?=w343:bool)
                  n173 = Select(t=w354, s=w343, f="") -> (s? t:f=w350:string)
                  n174 = Concatenate Strings(w352, "\t", w350) -> (w349:string)
                }
                n175 = Bundle(0, 1, "Centroid X"=w231) -> (→"Status":cluster{i32, i32, "Centroid X":dbl[][]})  [unwired: 1 in]
                n176 = call <vilib>:"Add State(s) to Queue__jki_lib_state_machine.vi"("State(s) in (\"\")"=w235, "State(s) at Back (\"\")"="Device Ini" ("State(s) at Back (\"\")")) -> ("States Out"=w234:string)  [unwired: 13 in]
                n177 = Bundle By Name(cluster=w267, "Centroid X"=w231, "Centroid Y"=w241, "Size"=w240) -> (w237:T35)
                n178 = Unbundle By Name(w237) -> ("img to avg"=w236:i32)
                n179 = case shown="True" w258 {
                  tunnel: w237 -> [w327 w334]
                  tunnel: [w327 w333] -> w259
                  tunnel: w236 -> [_ w329]
                  frame False {
                  }
                  frame True {
                    n180 = Decrement(x=w329) -> (x-1=w332:i32)
                    n181 = Initialize Array(0.0 ("element"), 12 ("dimension size"), w332) -> (w328:dbl[][])
                    n182 = Bundle By Name(cluster=w334, "Centroid X"=w328, "Centroid Y"=w328, "Size"=w328) -> (w333:T35)
                  }
                }
                n183 = Or Array Elements(Boolean array=w274) -> (logical OR=w273:bool)
                n184 = case shown="True" w273 {
                  tunnel: w272 -> [_ w339]
                  tunnel: w234 -> [w335 w338]
                  tunnel: [w335 w337] -> w260
                  frame False {
                  }
                  frame True {
                    n185 = call <vilib>:"Build State String with Arguments__jki_lib_state_machine.vi"("Arguments (\"\")"=w339, "State"="detected") -> ("State with Arguments"=w336:string)  [unwired: 4 in]
                    n186 = call <vilib>:"Add State(s) to Queue__jki_lib_state_machine.vi"("State(s) in Front (\"\")"=w336, "State(s) in (\"\")"=w338) -> ("States Out"=w337:string)  [unwired: 13 in]
                  }
                }
              }
              event "stop": Value Change {
                # "Exit Button Value Change (pressed) Event\n(this executes Macro: Exit to terminate the VI)"
                n187 = event-data() -> ()  [unwired: 1 in, 6 out]
                n188 = call <vilib>:"Add State(s) to Queue__jki_lib_state_machine.vi"("State(s) in Front (\"\")"="Macro: Exit", "State(s) in (\"\")"=w359) -> ("States Out"=w358:string)  [unwired: 13 in]
              }
              event Value Change {
                n189 = event-data() -> ()  [unwired: 1 in, 6 out]
                n190 = property on="Set Centriod Target" class="Bool (strict)"("Value"=FALSE) -> ()  [unwired: 2 in, 2 out]
                n191 = Unbundle By Name(w370) -> ("active ccd"=w362:i32, "Mean Centroid X"=w361:dbl[][], "Mean Centroid Y"=w360:dbl[][])
                n192 = Index Array(array=w366, index=w362) -> (element=w365:string)
                n193 = Concatenate Strings("Do want to update the target of " ("message"), w365, "?" ("string")) -> (w363:string)
                n194 = Two Button Dialog(message=w363) -> (T button?=w369:bool)  [unwired: 2 in]
                n195 = case shown="True" w369 {
                  tunnel: w368 -> [_ w383]
                  tunnel: w362 -> [_ w382]
                  tunnel: w361 -> [_ w389]
                  tunnel: w360 -> [_ w384]
                  frame False {
                  }
                  frame True {
                    n196 = Index Array(array=w389, index (row)=w382) -> (element=w388:dbl[])  [unwired: 1 in]
                    n197 = Index Array(array=w384, index (row)=w382) -> (element=w385:dbl[])  [unwired: 1 in]
                    n198 = Index Array(array=w383, index=w382) -> (element=w381:T29)
                    n199 = Unbundle By Name(w381) -> ("Target.X::12"=w380:refnum<vi>, "Target.Y::12"=w379:refnum<vi>)
                    n200 = Reverse 1D Array(array=w388) -> (reversed array=w387:dbl[])
                    n201 = Reverse 1D Array(array=w385) -> (reversed array=w386:dbl[])
                    n202 = Index Array(array=w387) -> (element=w378:dbl)  [unwired: 1 in]
                    n203 = Index Array(array=w386) -> (element=w376:dbl)  [unwired: 1 in]
                    n204 = To Unsigned Word Integer(number=w376) -> (unsigned 16bit integer=w375:u16)
                    n205 = To Unsigned Word Integer(number=w378) -> (unsigned 16bit integer=w377:u16)
                    n206 = disable-structure shown="Enabled" {
                      disable-tunnel: w380 -> [w393 _]
                      disable-tunnel: w377 -> [w392 _]
                      disable-tunnel: w379 -> [w391 _]
                      disable-tunnel: w375 -> [w390 _]
                      frame Enabled {
                        n207 = property class="DigNum (strict)"(reference=w393, "Val(Sgnl)"=w392) -> ()  [unwired: 1 in, 2 out]
                        n208 = property class="DigNum (strict)"(reference=w391, "Val(Sgnl)"=w390) -> ()  [unwired: 1 in, 2 out]
                      }
                      frame Disabled {
                      }
                    }
                  }
                }
                n209 = call <vilib>:"Add State(s) to Queue__jki_lib_state_machine.vi"("State(s) in (\"\")"=w374) -> ("States Out"=w373:string)  [unwired: 14 in]
              }
              event "Feedback Global": Value Change {
                # "Exit Button Value Change (pressed) Event\n(this executes Macro: Exit to terminate the VI)"
                n210 = event-data() -> ("NewVal"=w396:bool)  [unwired: 1 in, 5 out]
                n211 = call <vilib>:"Add State(s) to Queue__jki_lib_state_machine.vi"("State(s) in (\"\")"=w399) -> ("States Out"=w398:string)  [unwired: 14 in]
                n212 = Bundle By Name(cluster=w395, "Feedback global"=w396) -> (w394:T35)
              }
              event Value Change {
                n213 = event-data() -> ()  [unwired: 1 in, 6 out]
                n214 = call <vilib>:"Add State(s) to Queue__jki_lib_state_machine.vi"("State(s) in Front (\"\")"="Move Config", "State(s) in (\"\")"=w404) -> ("States Out"=w403:string)  [unwired: 13 in]
              }
              event Value Change {
                n215 = event-data() -> ()  [unwired: 1 in, 6 out]
                n216 = call <vilib>:"Add State(s) to Queue__jki_lib_state_machine.vi"("State(s) in Front (\"\")"="Detection Config", "State(s) in (\"\")"=w409) -> ("States Out"=w408:string)  [unwired: 13 in]
              }
              event "associated motors": Value Change {
                n217 = event-data() -> ()  [unwired: 1 in, 6 out]
                n218 = call <vilib>:"Add State(s) to Queue__jki_lib_state_machine.vi"("State(s) in (\"\")"=w414, "State(s) at Back (\"\")"="Motor Config" ("State(s) at Back (\"\")")) -> ("States Out"=w413:string)  [unwired: 13 in]
              }
              event "Reset History": Value Change {
                n219 = event-data() -> ()  [unwired: 1 in, 6 out]
                n220 = call <vilib>:"Add State(s) to Queue__jki_lib_state_machine.vi"("State(s) in (\"\")"=w420, "State(s) at Back (\"\")"="Reset History" ("State(s) at Back (\"\")")) -> ("States Out"=w419:string)  [unwired: 13 in]
                n221 = property on="Reset History" class="Bool (strict)"("Value"=FALSE ("Reset History")) -> ()  [unwired: 2 in, 2 out]
              }
              event "Save Config": Value Change {
                n222 = event-data() -> ()  [unwired: 1 in, 6 out]
                n223 = call <vilib>:"Add State(s) to Queue__jki_lib_state_machine.vi"("State(s) in (\"\")"=w425, "State(s) at Back (\"\")"="Save Config" ("State(s) at Back (\"\")")) -> ("States Out"=w424:string)  [unwired: 13 in]
              }
              event "Load Config": Value Change {
                n224 = event-data() -> ()  [unwired: 1 in, 6 out]
                n225 = call "File Dialog2"("pattern (all files)"="*.cfg", "pattern label"="config") -> ("selected path"=w429:path)  [unwired: 10 in, 3 out]
                n226 = Path To String(path=w429) -> (string=w427:string)
                "config path" <- w427
                n227 = call <vilib>:"Build State String with Arguments__jki_lib_state_machine.vi"("Arguments (\"\")"=w427, "State"="Load Config" ("State(s) at Back (\"\")")) -> ("State with Arguments"=w426:string)  [unwired: 4 in]
                n228 = call <vilib>:"Add State(s) to Queue__jki_lib_state_machine.vi"("State(s) in (\"\")"=w435, "State(s) at Back (\"\")"=w426) -> ("States Out"=w434:string)  [unwired: 13 in]
              }
              event "Save Stats": Value Change {
                n229 = event-data() -> ()  [unwired: 1 in, 6 out]
                n230 = call <vilib>:"Add State(s) to Queue__jki_lib_state_machine.vi"("State(s) in (\"\")"=w440, "State(s) at Back (\"\")"="Save Stats" ("State(s) at Back (\"\")")) -> ("States Out"=w439:string)  [unwired: 13 in]
              }
              event "Tab Cams": Value Change {
                n231 = event-data() -> ()  [unwired: 1 in, 6 out]
                n232 = call <vilib>:"Add State(s) to Queue__jki_lib_state_machine.vi"("State(s) in (\"\")"=w442, "State(s) at Back (\"\")"="stats" ("State")) -> ("States Out"=w441:string)  [unwired: 13 in]
              }
              event "active CCDs": Value Change {
                n233 = event-data() -> ("NewVal"=w451:i32)  [unwired: 1 in, 5 out]
                n234 = Unbundle By Name(w447) -> ("active cams"=w446:string[])
                n235 = Index Array(array=w446, index=w451) -> (element=w449:string)
                n236 = call <vilib>:"Build State String with Arguments__jki_lib_state_machine.vi"("Arguments (\"\")"=w449, "State"="active" ("State(s) at Back (\"\")")) -> ("State with Arguments"=w448:string)  [unwired: 4 in]
                n237 = call <vilib>:"Add State(s) to Queue__jki_lib_state_machine.vi"("State(s) in (\"\")"=w454, "State(s) at Back (\"\")"=w448) -> ("States Out"=w453:string)  [unwired: 13 in]
              }
              event "Left", "Right": Value Change {
                n238 = event-data() -> ("CtlRef"=w463:refnum<vi>)  [unwired: 1 in, 5 out]
                n239 = property class="Bool (strict)"(reference=w463, error in=w460) -> (reference out=w462:refnum<vi>, error out=w461:errorcluster, "Label.Text"=w457:string)
                n240 = property class="Bool (strict)"(reference=w462, error in=w461, "Value"=FALSE) -> (error out=w459:errorcluster)  [unwired: 1 out]
                n241 = call <vilib>:"Build State String with Arguments__jki_lib_state_machine.vi"("Arguments (\"\")"=w457, "State"="ManMove X") -> ("State with Arguments"=w456:string)  [unwired: 4 in]
                n242 = call <vilib>:"Add State(s) to Queue__jki_lib_state_machine.vi"("State(s) in (\"\")"=w466, "State(s) at Back (\"\")"=w456) -> ("States Out"=w465:string)  [unwired: 13 in]
              }
              event "Up", "Down": Value Change {
                n243 = event-data() -> ("CtlRef"=w475:refnum<vi>)  [unwired: 1 in, 5 out]
                n244 = property class="Bool (strict)"(reference=w475, error in=w472) -> (reference out=w474:refnum<vi>, error out=w473:errorcluster, "Label.Text"=w469:string)
                n245 = property class="Bool (strict)"(reference=w474, error in=w473, "Value"=FALSE) -> (error out=w471:errorcluster)  [unwired: 1 out]
                n246 = call <vilib>:"Build State String with Arguments__jki_lib_state_machine.vi"("Arguments (\"\")"=w469, "State"="ManMove Y") -> ("State with Arguments"=w468:string)  [unwired: 4 in]
                n247 = call <vilib>:"Add State(s) to Queue__jki_lib_state_machine.vi"("State(s) in (\"\")"=w478, "State(s) at Back (\"\")"=w468) -> ("States Out"=w477:string)  [unwired: 13 in]
              }
              event "Center": Value Change {
                n248 = event-data() -> ()  [unwired: 1 in, 6 out]
                n249 = call <vilib>:"Add State(s) to Queue__jki_lib_state_machine.vi"("State(s) in (\"\")"=w483, "State(s) at Back (\"\")"="Center" ("State(s) at Back (\"\")")) -> ("States Out"=w482:string)  [unwired: 13 in]
              }
              event "new tdms": Value Change {
                n250 = event-data() -> ()  [unwired: 1 in, 6 out]
                n251 = call <vilib>:"Add State(s) to Queue__jki_lib_state_machine.vi"("State(s) in (\"\")"=w488, "State(s) at Back (\"\")"="newtdms" ("State(s) at Back (\"\")")) -> ("States Out"=w487:string)  [unwired: 13 in]
              }
              event "device ini": Value Change {
                n252 = event-data() -> ()  [unwired: 1 in, 6 out]
                n253 = property on="device ini" class="Bool (strict)"("Value"=FALSE ("test")) -> ()  [unwired: 2 in, 2 out]
                n254 = call <vilib>:"Add State(s) to Queue__jki_lib_state_machine.vi"("State(s) in (\"\")"=w494, "State(s) at Back (\"\")"="Device Ini" ("State(s) at Back (\"\")")) -> ("States Out"=w493:string)  [unwired: 13 in]
              }
              event "img to avg": Value Change {
                n255 = event-data() -> ("NewVal"=w500:i32)  [unwired: 1 in, 5 out]
                n256 = Number To Decimal String(number=w500) -> (decimal integer string=w502:string)  [unwired: 1 in]
                n257 = call <vilib>:"Build State String with Arguments__jki_lib_state_machine.vi"("Arguments (\"\")"=w502, "State"="ImgToAvg" ("State(s) at Back (\"\")")) -> ("State with Arguments"=w495:string)  [unwired: 4 in]
                n258 = call <vilib>:"Add State(s) to Queue__jki_lib_state_machine.vi"("State(s) in Front (\"\")"=w495, "State(s) in (\"\")"=w498) -> ("States Out"=w497:string)  [unwired: 13 in]
              }
              event Panel Close? {
                # "Discard the event because we'll close the front panel ourselves in Macro: Exit"
                # "Close Panel button (pressed) Event\n(this executes Macro: Exit to terminate the VI)"
                n259 = event-data() -> ()  [unwired: 1 in, 1 out]
                n260 = call <vilib>:"Add State(s) to Queue__jki_lib_state_machine.vi"("State(s) in Front (\"\")"="Macro: Exit", "State(s) in (\"\")"=w508) -> ("States Out"=w507:string)  [unwired: 13 in]
                n261 = event-data("Discard?"=TRUE) -> ()  [unwired: 1 in, 1 out]
              }
            }
          }
          frame "---------- Core ----------" {
            # "Do not put any code in this frame.\n(it is a separator no-op)"
            n262 = call <vilib>:"Add State(s) to Queue__jki_lib_state_machine.vi"("State(s) in (\"\")"=w512) -> ("States Out"=w511:string)  [unwired: 14 in]
          }
          frame Default {
            w522 = 42 items=["No error", "Argument error", "Memory is full", "Out of zone", "End of file", "File already open", "Generic file I/O error", "File not found", "File permission error", "Disk is full", "Duplicate path", "Too many files open", "System feature not enabled", "Resource file not found", "Cannot add resource", "Resource not found", "Image not found", "Image memory error", "Pen does not exist", "Config type invalid", "Config token not found", "Config parse error", "Config memory error", "Bad external code format", "Bad external code offset", "External code not present", "Null window", "Destroy window error", "Null menu", "Print aborted", "Bad print record", "Print driver error", "Windows error during printing", "Memory error during printing", "Print dialog error", "Generic print error", "Invalid device refnum", "Device not found", "Device parameter error", "Device unit error", "Cannot open device", "Device call aborted", "Generic error", "Cancelled by user", "Object ID too low", "Object ID too high", "Object not in heap", "Unknown heap", "Unknown object (invalid DefProc)", "Unknown object (DefProc not in table)", "Message out of range", "Invalid (null) method", "Unknown message", "Manager call not supported", "Bad address", "Network operation in progress", "Network operation timed out", "Connection is busy", "Network attribute not supported", "Network error", "Address in use", "System out of memory", "Connection aborted", "Connection refused", "Not connected", "Already connected", "Connection closed", "Initialization error (interapplication manager)", "Bad occurrence", "Wait on unbound occurrence handler", "Occurrence queue overflow", "Datalog type conflict", "Unused", "Unrecognized type (interapplication manager)", "Memory corrupt", "Failed to make temporary DLL", "Old CIN version", "Drag socket not found", "Failed to load drop-object", "Failed to register OLE object", "Failed to release OLE object", "Format specifier type mismatch", "Unknown format specifier", "Too few format specifiers", "Too many format specifiers", "Scan failed", "Newer CIN version", "Error converting to variant", "Runtime menu error", "Password tampered", "Variant attribute not found", "Incompatible variant data type", "Event data is not available", "Event Store is not present", "Occurrence is not found", "Event Queue is not created", "Event info is not available", "Refnum passed is NULL", "Error retrieving Class GUID", "Error retrieving CoClass GUID", "Error retrieving TypeLib GUID.", "Bad built application magic bytes.", "Specific driver is different from the specific driver associated with the Logical Name.", "There is no session opened to the class driver.", "Max Error", "MAX - Error with config objects", "MAX - Error loading configuration", "MAX - Group not supported"]
            # "Current State"
            # "Do not delete, rename, or modify this frame.\n(this is used to capture unhandled states and typos)"
            # "Handle mistyped state name (developer tool)"
            n263 = Format Into String(format string="Software Exception: Unhandled State \"%s\"." ("message"), error in=w518, w513) -> (resulting string=w521:string, error out=w520:errorcluster)  [unwired: 1 in]
            n264 = call <vilib>:"Error Cluster From Error Code.vi"("show call chain? (False)"=TRUE, "error in (no error)"=w520, "error message (\"\")"=w521, "error code (0)"=w522) -> ("error out"=w519:errorcluster)  [unwired: 5 in]
            n265 = call <vilib>:"Add State(s) to Queue__jki_lib_state_machine.vi"("State(s) in (\"\")"=w517) -> ("States Out"=w516:string)  [unwired: 14 in]
          }
          frame "Initialize Core Data" {
            # "Do not delete, rename, or modify this frame.\n(this is used to determine panel behavior on exit)"
            # "originally closed?"
            # "exe?"
            # "If panel starts closed or is an EXE, then close it when we exit"
            n266 = property class="VI"() -> ("Front Panel.Open"=w532:bool)  [unwired: 2 in, 2 out]
            n267 = property class="App"() -> ("App.Kind"=w531:T14)  [unwired: 2 in, 2 out]
            n268 = control-ref of="Current VI Reference"() -> (w526:refnum<vi>)
            n269 = Not(x=w532) -> (.not. x?=w529:bool)
            n270 = Equal?(x=w531, y=T14."Run Time System" ("Application:Kind")) -> (x = y?=w528:bool)
            n271 = Or(x=w529, y=w528) -> (x .or. y?=w527:bool)
            n272 = Bundle By Name(cluster=w525, "Core.Current VI Reference"=w526, "Core.Close Panel on Exit?"=w527) -> (w524:T35)
            n273 = call <vilib>:"Add State(s) to Queue__jki_lib_state_machine.vi"("State(s) in (\"\")"=w535) -> ("States Out"=w534:string)  [unwired: 14 in]
          }
          frame "Error Handler" {
            # "Unhandled Error -- Display it"
            # "Handle any errors here.\nYou can also output any states to clean-up after errors occur"
            # "Clear error"
            n274 = call <vilib>:"General Error Handler.vi"("error in (no error)"=w537) -> ()  [unwired: 10 in, 5 out]
            n275 = call <vilib>:"Add State(s) to Queue__jki_lib_state_machine.vi"("State(s) in Front (\"\")"="/* Post Error States", "State(s) in (\"\")"=w541) -> ("States Out"=w540:string)  [unwired: 13 in]
          }
          frame "Exit" {
            # "Do not put any code in this frame.\n(No errors that occur here will be handled.)"
            n276 = call <vilib>:"Add State(s) to Queue__jki_lib_state_machine.vi"("State(s) in (\"\")"=w546) -> ("States Out"=w545:string)  [unwired: 14 in]
          }
          frame "---------- Data ----------" {
            # "Do not put any code in this frame.\n(It is a separator no-op. You can make a copy of this frame to create a new Data frame)"
            n277 = call <vilib>:"Add State(s) to Queue__jki_lib_state_machine.vi"("State(s) in (\"\")"=w550) -> ("States Out"=w549:string)  [unwired: 14 in]
          }
          frame "Data: Initialize" {
            w551 = dbl[] [0.0, 0.0, 0.0, 0.0, 0.0, 0.0, 0.0, 0.0, 0.0, 0.0, 0.0, 0.0]  # steps speed Y
            w552 = dbl[] [0.0, 0.0, 0.0, 0.0, 0.0, 0.0, 0.0, 0.0, 0.0, 0.0, 0.0, 0.0]  # steps speed X
            w556 = bool[] [FALSE, FALSE, FALSE, FALSE, TRUE, TRUE, TRUE, FALSE, FALSE, FALSE, FALSE, FALSE]  # detected
            w566 = bool[] [FALSE, FALSE, FALSE, FALSE, FALSE, FALSE, FALSE, FALSE, FALSE, FALSE, FALSE, TRUE]  # speedmode Y
            w567 = bool[] [FALSE, FALSE, FALSE, FALSE, FALSE, FALSE, FALSE, FALSE, FALSE, FALSE, FALSE, TRUE]  # speedmode X
            w569 = cluster{"Lower value":sgl, "Upper value":sgl}[] [{"Lower value"=93.0, "Upper value"=255.0}, {"Lower value"=105.0, "Upper value"=255.0}, {"Lower value"=0.0, "Upper value"=255.0}, {"Lower value"=127.0, "Upper value"=255.0}, {"Lower value"=0.0, "Upper value"=255.0}, {"Lower value"=0.0, "Upper value"=255.0}, {"Lower value"=0.0, "Upper value"=255.0}, {"Lower value"=0.0, "Upper value"=255.0}, {"Lower value"=0.0, "Upper value"=255.0}, {"Lower value"=0.0, "Upper value"=255.0}, {"Lower value"=0.0, "Upper value"=255.0}, {"Lower value"=0.0, "Upper value"=255.0}]  # thresholds
            w576 = FALSE  # Feedback global
            w578 = 0  # active ccd
            w562 = 6  # img to avg
            w589 = T36 {"Current VI Reference"=refnum, "Close Panel on Exit?"=FALSE}  # Core
            # "Initialize the shift-register data, here.\n(data names are defined by what you wire into the bundle function)"
            n278 = disable-structure shown="Disabled" {
              disable-tunnel: w559 -> [w601 _]
              disable-tunnel: [w600 _] -> w558
              disable-tunnel: w557 -> [w599 _]
              disable-tunnel: [w598 _] -> _
              disable-tunnel: w555 -> [w592 _]
              frame Disabled {
                n279 = TDMS Open(6:FALSE ("disable buffering (T)"), 7:enum16{"1.0", "2.0"}."2.0" ("file format version (2.0)"), 8:w601, 10:T15."create or replace" ("operation"), 11:w599) -> (0:w596:errorcluster, 3:w597:refnum<k34>)  [unwired: 2 in]
                n280 = call "TDMSbuffersize.vi"("error in (no error)"=w596, "group names"=w592, "Data Value Reference in"=w597) -> ("error out"=w600:errorcluster, "Data Value Reference out"=w598:refnum<k34>)  [unwired: 7 in]
              }
              frame Enabled {
              }
            }
            n281 = call <vilib>:"Add State(s) to Queue__jki_lib_state_machine.vi"("State(s) in Front (\"\")"="newtdms" ("State(s) in Front (\"\")"), "State(s) in (\"\")"=w591) -> ("States Out"=w590:string)  [unwired: 13 in]
            n282 = Bundle("Core"=w589, "detection para"="detection para", "thresholds"=w569, "Centroid X"="Centroid X", "Centroid Y"="Centroid Y", "img to avg"=w562, "Mean Centroid X"="Mean Centroid X", "Mean Centroid Y"="Mean Centroid Y", "Offset X"="Offset X", "Offset Y"="Offset Y", "Offset X stats"="Offset X stats", "Offset Y stats"="Offset Y stats", "Size"="Size", "Mean Size"="Mean Size", "Time"="Time", "move properties"="move properties", "active axis refs 2"="active axis refs 2", "active ccd"=w578, "Feedback global"=w576, "Motor X"="Motor X", "Motor Y"="Motor Y", "active cams"="active cams", "Data Value Reference out"=refnum<k34> refnum, "active man refs"="active man refs", "detected"=w556, "speedmode X"=w567, "speedmode Y"=w566, "steps speed X"=w552, "steps speed Y"=w551) -> (w561:T35)  [unwired: 1 in]
            n283 = Initialize Array(0.0 ("element"), 12 ("dimension size"), w562) -> (w565:dbl[][])
            n284 = Bundle By Name(cluster=w561, "Centroid X"=w565, "Centroid Y"=w565, "Size"=w565) -> (w560:T35)
          }
          frame "Data: Cleanup" {
            # "Cleanup any data and references, here.\n(this is called automatically, by the Macro: Exit)"
            n285 = Unbundle By Name(w602) -> ("Core.Current VI Reference"=w603:refnum<vi>)
            n286 = Close Reference(reference=w603, error in (no error)=w605) -> (error out=w604:errorcluster)
            n287 = call <vilib>:"Add State(s) to Queue__jki_lib_state_machine.vi"("State(s) in (\"\")"=w607) -> ("States Out"=w606:string)  [unwired: 14 in]
          }
          frame "---------- UI ----------" {
            # "Do not put any code in this frame.\n(It is a separator no-op. You can make a copy of this frame to create a new UI frame)"
            n288 = call <vilib>:"Add State(s) to Queue__jki_lib_state_machine.vi"("State(s) in (\"\")"=w611) -> ("States Out"=w610:string)  [unwired: 14 in]
          }
          frame "UI: Initialize" {
            # "Initialize the User Interface, here.\n(this is called automatically, by the Macro: Init)"
            n289 = call <vilib>:"Add State(s) to Queue__jki_lib_state_machine.vi"("State(s) in (\"\")"=w615) -> ("States Out"=w614:string)  [unwired: 14 in]
          }
          frame "UI: Cursor Set" {
            # "Argument"
            # "Set and Unset Cursor Busy.\n(Usage: \"UI: Cursor Set >> Busy|Idle\")"
            n290 = case shown="\"Idle\", Default" w616 {
              tunnel: w618 -> [w623 w625]
              tunnel: [w622 w624] -> w617
              frame "Idle", Default {
                n291 = call <vilib>:"Unset Busy.vi"("error in (no error)"=w623) -> ("error out"=w622:errorcluster)  [unwired: 10 in]
              }
              frame "Busy" {
                n292 = call <vilib>:"Set Busy.vi"("error in (no error)"=w625) -> ("error out"=w624:errorcluster)  [unwired: 9 in, 1 out]
              }
            }
            n293 = call <vilib>:"Add State(s) to Queue__jki_lib_state_machine.vi"("State(s) in (\"\")"=w621) -> ("States Out"=w620:string)  [unwired: 14 in]
          }
          frame "UI: Front Panel State" {
            # "Argument"
            # "Set Front Panel Open or Closed\n(Usage: \"UI: Front Panel State >> Open|Close\")"
            n294 = Unbundle By Name(w626) -> ("Core.Current VI Reference"=w628:refnum<vi>)
            n295 = case shown="\"Open\", Default" w627 {
              tunnel: w630 -> [w636 w647]
              tunnel: [w637 w648] -> w629
              tunnel: w628 -> [_ _]
              frame "Open", Default {
                n296 = property class="VI"(error in=w636) -> (reference out=w634:refnum<vi>, error out=w635:errorcluster, "Front Panel.Open"=w633:bool)  [unwired: 1 in]
                n297 = case shown="False" w633 {
                  tunnel: [w640 w643] -> w637
                  tunnel: w635 -> [w639 w643]
                  tunnel: w634 -> [w638 _]
                  frame False {
                    n298 = invoke class="VI" method="FP.Open"(reference=w638, error in=w639, "Activate"=TRUE, "State"=T16."Standard") -> (error out=w640:errorcluster)  [unwired: 1 in, 4 out]
                  }
                  frame True {
                  }
                }
              }
              frame "Close" {
                n299 = property class="VI"(error in=w647) -> (reference out=w645:refnum<vi>, error out=w646:errorcluster, "Front Panel.Open"=w644:bool)  [unwired: 1 in]
                n300 = case shown="True" w644 {
                  tunnel: [w649 w652] -> w648
                  tunnel: w646 -> [w649 w651]
                  tunnel: w645 -> [_ w650]
                  frame False {
                  }
                  frame True {
                    n301 = invoke class="VI" method="FP.Close"(reference=w650, error in=w651) -> (error out=w652:errorcluster)  [unwired: 1 in, 2 out]
                  }
                }
              }
            }
            n302 = call <vilib>:"Add State(s) to Queue__jki_lib_state_machine.vi"("State(s) in (\"\")"=w632) -> ("States Out"=w631:string)  [unwired: 14 in]
          }
          frame "---------- Macro ----------" {
            # "Do not put any code in this frame.\n(It is a separator no-op. You can make a copy of this frame to create a new Macro frame)"
            n303 = call <vilib>:"Add State(s) to Queue__jki_lib_state_machine.vi"("State(s) in (\"\")"=w656) -> ("States Out"=w655:string)  [unwired: 14 in]
          }
          frame "Macro: Initialize" {
            # "Initialization Macro\n(This is called once, when the VI starts)"
            n304 = property on="img to avg" class="DigNum (strict)"() -> ("Value"=w658:i32)  [unwired: 2 in, 2 out]
            n305 = Number To Decimal String(number=w658) -> (decimal integer string=w660:string)  [unwired: 1 in]
            n306 = call <vilib>:"Build State String with Arguments__jki_lib_state_machine.vi"("Arguments (\"\")"=w660, "State"="ImgToAvg") -> ("State with Arguments"=w657:string)  [unwired: 4 in]
            n307 = call <vilib>:"Add State(s) to Queue__jki_lib_state_machine.vi"("State(s) in Front (\"\")"="Data: Initialize\nInitialize Core Data\nUI: Initialize\nUI: Front Panel State >> Open\nDevice Ini >> 3000", "State(s) in (\"\")"=w665, "State(s) at Back (\"\")"=w657) -> ("States Out"=w664:string)  [unwired: 12 in]
          }
          frame "Macro: Exit" {
            # "Exit Macro\n(This is called once, when the VI exits)"
            n308 = Unbundle By Name(w667) -> ("Core.Close Panel on Exit?"=w666:bool)
            n309 = Select(t="UI: Front Panel State >> Close", s=w666, f="") -> (s? t:f=w670:string)
            n310 = call <vilib>:"Add State(s) to Queue__jki_lib_state_machine.vi"("State(s) in (\"\")"=w670, "State(s) at Back (\"\")"="Data: Cleanup\nExit") -> ("States Out"=w668:string)  [unwired: 13 in]
            n311 = call <vilib>:"Add State(s) to Queue__jki_lib_state_machine.vi"("State(s) in Front (\"\")"=w668, "State(s) in (\"\")"=w675) -> ("States Out"=w674:string)  [unwired: 13 in]
          }
          frame "---------- Ini and Configure ----------" {
            # "Template Separator\n(You can make a copy of, or modify, this frame)"
            n312 = call <vilib>:"Add State(s) to Queue__jki_lib_state_machine.vi"("State(s) in (\"\")"=w679) -> ("States Out"=w678:string)  [unwired: 14 in]
          }
          frame "Device Ini" {
            # "Your code here.\n(You can make a copy of, or modify, this frame)"
            n313 = Empty String/Path?(string/path=w683) -> (empty?=w700:bool)
            n314 = flat-sequence {
              tunnel: w706 -> [w745]
              tunnel: [w745] -> w705
              tunnel: w699 -> [w744]
              tunnel: w705 -> [w751]
              tunnel: [w749] -> w686
              tunnel: [w748] -> _
              frame #0 {
                n315 = Wait (ms)(milliseconds to wait=w744) -> ()  [unwired: 1 out]
              }
              frame #1 {
                n316 = local read "Array 3"() -> (w746:sgl[])
                n317 = disable-structure shown="Disabled" {
                  disable-tunnel: w751 -> [w754 _]
                  disable-tunnel: [w752 _] -> w748
                  frame Disabled {
                    n318 = for {
                      tunnel: w754 -> [w755] mode=indexing
                      shift-right: [w757] -> w752
                      shift-left: string[] [] -> [w758]
                      n319 = call "send command.vi"("Device Name"=w755) -> ("status"=w759:bool)  [unwired: 4 in]
                      n320 = Wait (ms)(milliseconds to wait=u32 1) -> ()  [unwired: 1 out]
                      n321 = case shown="True" w759 {
                        tunnel: w758 -> [w760 w763]
                        tunnel: [w760 w762] -> w757
                        tunnel: w755 -> [_ w761]
                        frame False {
                        }
                        frame True {
                          n322 = Build Array (concatenate)(w763, w761) -> (w762:string[])
                        }
                      }
                    }
                  }
                  frame Enabled {
                  }
                }
                n323 = for {
                  tunnel: w751 -> [w766] mode=indexing
                  shift-right: [w771] -> w749
                  shift-left: string[] [] -> [w772]
                  tunnel: [w765] -> w747 mode=indexing
                  shift-right: [w769] -> _
                  shift-left: w746 -> [w769]
                  i -> [w770]
                  n324 = call "IMAQ Histograph"("Image"=w766) -> ("error out"=w764:errorcluster, "Mean Value"=w765:sgl)  [unwired: 7 in, 2 out]
                  n325 = Index Array(array=w769, index=w770) -> (element=w768:sgl)
                  n326 = call <vilib>:"Clear Errors.vi"("error in (no error)"=w764) -> ()  [unwired: 6 in, 1 out]
                  n327 = Equal?(x=w765, y=w768) -> (x = y?=w767:bool)
                  n328 = case shown="False" w767 {
                    tunnel: w772 -> [w775 w776]
                    tunnel: [w774 w776] -> w771
                    tunnel: w766 -> [w773 _]
                    frame False {
                      n329 = Build Array (concatenate)(w775, w773) -> (w774:string[])
                    }
                    frame True {
                    }
                  }
                }
                "Array 3" <- w747
              }
            }
            n330 = case shown="False" w700 {
              tunnel: w683 -> [w742 _]
              tunnel: [w741 0] -> w699
              frame False {
                n331 = Decimal String To Number(string=w742) -> (number=w741:i32)  [unwired: 2 in, 1 out]
              }
              frame True {
              }
            }
            n332 = Equal?(x=w683, y="T") -> (x = y?=w681:bool)
            n333 = Unbundle By Name(w698) -> ("active cams"=w691:string[])
            n334 = call <vilib>:"Add State(s) to Queue__jki_lib_state_machine.vi"("State(s) in (\"\")"=w707) -> ("States Out"=w693:string)  [unwired: 14 in]
            n335 = Equal?(x=w691, y=w686) -> (x = y?=w697:bool[])
            n336 = Empty Array?(array=w691) -> (empty?=w696:bool)
            n337 = Not(x=w696) -> (.not. x?=w695:bool)
            n338 = Build Array (concatenate)(w697, w695) -> (w694:bool[])
            n339 = Array Size(array=w686) -> (size(s)=w690:i32)
            n340 = Array Size(array=w691) -> (size(s)=w689:i32)
            n341 = And Array Elements(Boolean array=w694) -> (logical AND=w687:bool)
            n342 = Equal?(x=w690, y=w689) -> (x = y?=w688:bool)
            n343 = And(x=w688, y=w687) -> (x .and. y?=w685:bool)
            n344 = Not(x=w685) -> (.not. x?=w682:bool)
            n345 = Or(x=w682, y=w681) -> (x .or. y?=w680:bool)
            n346 = case shown="True" w680 {
              tunnel: [w710 w726] -> w704
              tunnel: w703 -> [_ _]
              tunnel: w702 -> [w709 w724]
              tunnel: [w709 w724] -> w701
              tunnel: w698 -> [w710 w720]
              tunnel: w686 -> [_ w721]
              tunnel: w693 -> [w708 _]
              tunnel: [w708 w714] -> w692
              frame False {
              }
              frame True {
                n347 = property on="active CCDs" class="LstBox (strict)"("Item Names"=w721) -> ()  [unwired: 2 in, 2 out]
                n348 = Array Size(array=w721) -> (size(s)=w733:i32)
                n349 = Initialize Array(0.0 ("element"), w733, 0 ("dimension size")) -> (w728:dbl[][])
                n350 = Unbundle By Name(w720) -> ("img to avg"=w719:i32)
                n351 = Bundle By Name(cluster=w720, "active cams"=w721) -> (w727:T35)
                n352 = Initialize Array(0.0 ("element"), 12 ("dimension size"), w719) -> (w718:dbl[][])
                n353 = local write "Numeric"(0.0 ("Numeric")) -> ()
                n354 = Bundle By Name(cluster=w727, "Offset X stats"=w728, "Offset Y stats"=w728, "Centroid X"=w718, "Centroid Y"=w718, "Mean Centroid X"=w728, "Mean Centroid Y"=w728, "Offset X"=w728, "Offset Y"=w728, "Size"=w718, "Mean Size"=w728, "Motor X"=w728, "Motor Y"=w728) -> (w726:T35)
                n355 = for {
                  N: 1 -> [_]
                  shift-right: [w735] -> w731
                  shift-left: timestamp[][] [] ("Time") -> [w737]
                  n356 = for {
                    N: 12 -> [_]
                    tunnel: w737 -> [w740] mode=indexing
                    tunnel: [w738] -> w735 mode=indexing
                    n357 = Get Date/Time In Seconds() -> (seconds since 1Jan1904=w739:timestamp)
                    n358 = Build Array (concatenate)(w740, w739) -> (w738:timestamp[])
                  }
                }
                n359 = property on="config path" class="Str"() -> ("Value"=w716:string)  [unwired: 2 in, 2 out]
                n360 = call <vilib>:"Add State(s) to Queue__jki_lib_state_machine.vi"("State(s) in Front (\"\")"="Move Config\nMotor Config\nDetection Config\nactive\nCenter" ("State(s) in Front (\"\")"), "State(s) in (\"\")"="" ("State(s) in (\"\")")) -> ("States Out"=w715:string)  [unwired: 13 in]
                n361 = call <vilib>:"Build State String with Arguments__jki_lib_state_machine.vi"("Arguments (\"\")"=w716, "State"="Load Config" ("State(s) in Front (\"\")")) -> ("State with Arguments"=w713:string)  [unwired: 4 in]
                n362 = call <vilib>:"Add State(s) to Queue__jki_lib_state_machine.vi"("State(s) in (\"\")"=w715, "State(s) at Back (\"\")"=w713) -> ("States Out"=w714:string)  [unwired: 13 in]
                n363 = property on="Time" class="Arr (strict)"("Value"=w731) -> ()  [unwired: 2 in, 2 out]
                "name array" <- w721
              }
            }
          }
          frame "Load Config" {
            # "Your code here.\n(You can make a copy of, or modify, this frame)"
            n364 = Unbundle By Name(w818) -> ("detection para"=w824:T3[], "move properties"=w821:T2[], "thresholds"=w814:cluster{"Lower value":sgl, "Upper value":sgl}[])
            n365 = Empty String/Path?(string/path=w781) -> (empty?=w780:bool)
            n366 = case shown="False" w780 {
              tunnel: [w834 T5 {"CCDs"=[], "move properties"=[], "detection para"=[], "thresholds"=[], "Value"={"Motor CCD 1"=0, "Motor CCD 2"=0, "Motor CCD 3"=0, "Motor CCD 4"=0, "Motor CCD 5"=0, "Motor CCD 6"=0, "Motor CCD 7"=0, "Motor CCD 8"=0, "Motor CCD 9"=0, "Motor CCD 10"=0, "Motor CCD 11"=0, "Motor CCD 12"=0}} ("output cluster 2")] -> w826
              tunnel: [w832 w841] -> w785
              tunnel: w782 -> [w831 w841]
              tunnel: w781 -> [w830 _]
              frame False {
                n367 = String To Path(string=w830) -> (path=w829:path)
                n368 = Open/Create/Replace File(file path (use dialog)=w829, error in=w831, operation (0:open)=T17."open or create") -> (refnum out=w836:refnum<file>, error out=w837:errorcluster)  [unwired: 3 in, 1 out]
                n369 = Read from Binary File(5:"output cluster 2", 8:w837, 11:w836) -> (0:w838:errorcluster, 2:w834:T5, 3:w839:refnum<file>)  [unwired: 3 in, 1 out]
                n370 = Close File(refnum=w839, error in=w838) -> (error out=w832:errorcluster)  [unwired: 1 out]
              }
              frame True {
              }
            }
            n371 = property on="Load Config" class="Bool (strict)"("Value"=FALSE ("Load Config")) -> ()  [unwired: 2 in, 2 out]
            n372 = Unbundle By Name(w826) -> ("Value"=w812:T7, "CCDs"=w825:string[], "detection para"=w823:T3[], "move properties"=w822:T2[], "thresholds"=w815:cluster{"Lower value":sgl, "Upper value":sgl}[])
            n373 = Cluster To Array(cluster=w812) -> (array=w813:u16[])
            n374 = call <vilib>:"Add State(s) to Queue__jki_lib_state_machine.vi"("State(s) in (\"\")"=w828, "State(s) at Back (\"\")"="Motor Config" ("State(s) at Back (\"\")")) -> ("States Out"=w827:string)  [unwired: 13 in]
            n375 = for {
              tunnel: w825 -> [w857]
              tunnel: w823 -> [w859]
              tunnel: w822 -> [w858]
              shift-right: [w851] -> w820
              shift-left: w824 -> [w856]
              shift-right: [w849] -> w819
              shift-left: w821 -> [w855]
              tunnel: w816 -> [w854] mode=indexing
              tunnel: w815 -> [w850]
              shift-right: [w846] -> w778
              shift-left: w814 -> [w848]
              tunnel: w813 -> [w845]
              tunnel: [w842] -> w811 mode=indexing
              i -> [w843]
              n376 = call-poly <userlib>:"Filter 1D Array__ogtk.vi"("items to filter"=w854, "array"=w857) -> ("filtered item indices"=w860:i32[])  [unwired: 4 in, 1 out]
              n377 = Index Array(array=w860) -> (element=w844:i32)  [unwired: 1 in]
              n378 = Index Array(array=w845, index=w844) -> (element=w842:u16)
              n379 = Index Array(array=w859, index=w844) -> (element=w853:T3)
              n380 = Index Array(array=w858, index=w844) -> (element=w852:T2)
              n381 = Index Array(array=w850, index=w844) -> (element=w847:cluster{"Lower value":sgl, "Upper value":sgl})
              n382 = Replace Array Subset(array=w856, new element=w853, index=w843) -> (w851:T3[])
              n383 = Replace Array Subset(array=w855, new element=w852, index=w843) -> (w849:T2[])
              n384 = Replace Array Subset(array=w848, new element=w847, index=w843) -> (w846:cluster{"Lower value":sgl, "Upper value":sgl}[])
            }
            n385 = Array Size(array=w778) -> (size(s)=→"size(s) 6":i32)
            n386 = Index Array(array=w811, index #1=0 ("index (row)"), index #2=1 ("index (row)"), index #3=2 ("index (row)"), index #4=3 ("index (row)"), index #5=4 ("index (row)"), index #6=5 ("index (row)"), index #7=6 ("index (row)"), index #8=7 ("index (row)"), index #9=8 ("index (row)"), index #10=9 ("index (row)"), index #11=10 ("index (row)"), index #12=11 ("index (row)")) -> (element #1=w798:u16, element #2=w797:u16, element #3=w796:u16, element #4=w795:u16, element #5=w794:u16, element #6=w793:u16, element #7=w792:u16, element #8=w791:u16, element #9=w790:u16, element #10=w789:u16, element #11=w788:u16, element #12=w787:u16)
            n387 = Bundle By Name(cluster=w812, "Motor CCD 1"=w798, "Motor CCD 2"=w797, "Motor CCD 3"=w796, "Motor CCD 4"=w795, "Motor CCD 5"=w794, "Motor CCD 6"=w793, "Motor CCD 7"=w792, "Motor CCD 8"=w791, "Motor CCD 9"=w790, "Motor CCD 10"=w789, "Motor CCD 11"=w788, "Motor CCD 12"=w787) -> (w786:T7)
            n388 = Bundle By Name(cluster=w818, "detection para"=w820, "move properties"=w819, "thresholds"=w778) -> (w817:T35)
            n389 = property on="associated motors" class="Clust (strict)"(error in=w785, "Val(Sgnl)"=w786) -> (error out=w784:errorcluster)  [unwired: 1 in, 1 out]
          }
          frame "Save Config" {
            # "Your code here.\n(You can make a copy of, or modify, this frame)"
            n390 = Unbundle By Name(w878) -> ("move properties"=w864:T2[], "detection para"=w873:T3[], "thresholds"=w861:cluster{"Lower value":sgl, "Upper value":sgl}[])
            n391 = property on="associated motors" class="Clust (strict)"() -> ("Value"=w872:T7)  [unwired: 2 in, 2 out]
            n392 = property on="Save Config" class="Bool (strict)"("Value"=FALSE ("Save Config")) -> ()  [unwired: 2 in, 2 out]
            n393 = local read "CCDs"() -> (w862:string[])
            n394 = call "File Dialog"("pattern (all files)"="*.cfg", "pattern label"="config") -> ("selected path"=w866:path)  [unwired: 10 in, 3 out]
            n395 = Bundle("CCDs"=w862, "move properties"=w864, "detection para"=w873, "thresholds"=w861, "Value"=w872) -> (w865:T5)  [unwired: 1 in]
            n396 = Open/Create/Replace File(file path (use dialog)=w866, error in=w870, operation (0:open)=T17."replace or create with confirmation") -> (refnum out=w874:refnum<file>, error out=w875:errorcluster)  [unwired: 3 in, 1 out]
            n397 = Write to Binary File(file (use dialog)=w874, data=w865, error in=w875) -> (refnum out=w877:refnum<file>, error out=w876:errorcluster)  [unwired: 3 in, 1 out]
            n398 = Close File(refnum=w877, error in=w876) -> (error out=w869:errorcluster)  [unwired: 1 out]
            n399 = call <vilib>:"Add State(s) to Queue__jki_lib_state_machine.vi"("State(s) in (\"\")"=w880) -> ("States Out"=w879:string)  [unwired: 14 in]
          }
          frame "active" {
            # "Your code here.\n(You can make a copy of, or modify, this frame)"
            n400 = Empty String/Path?(string/path=w895) -> (empty?=w894:bool)
            n401 = Unbundle By Name(w891) -> ("move properties"=w907:T2[], "detection para"=w903:T3[])  [unwired: 1 out]
            n402 = Unbundle By Name(w891) -> ("active axis refs 2"=w890:T11)
            n403 = call-poly <userlib>:"Filter 1D Array__ogtk.vi"("items to filter"=w895, "array"=w905) -> ("filtered item indices"=w908:i32[])  [unwired: 4 in, 1 out]
            n404 = Index Array(array=w908) -> (element=w892:i32)  [unwired: 1 in]
            n405 = Select(t=0, s=w894, f=w892) -> (s? t:f=w888:i32)
            n406 = Index Array(array=w890, index=w888) -> (element=w889:cluster{"Ref X":refnum<vi>, "Ref Y":refnum<vi>})
            n407 = Unbundle By Name(w889) -> ("Ref X"=w887:refnum<vi>, "Ref Y"=w886:refnum<vi>)
            n408 = Index Array(array=w907, index=w888) -> (element=w906:T2)
            n409 = Index Array(array=w903, index=w888) -> (element=w902:T3)
            n410 = property on="move config" class="Clust (strict)"(error in=w898, "Value"=w906) -> (error out=w896:errorcluster)  [unwired: 1 in, 1 out]
            n411 = property on="beam detection para" class="Clust (strict)"(error in=w896, "Value"=w902) -> (error out=w897:errorcluster)  [unwired: 1 in, 1 out]
            n412 = call <vilib>:"Add State(s) to Queue__jki_lib_state_machine.vi"("State(s) in (\"\")"=w910) -> ("States Out"=w909:string)  [unwired: 14 in]
            n413 = Bundle By Name(cluster="active Axis ref 3", "Ref X"=w887, "Ref Y"=w886) -> (w900:cluster{"Ref X":refnum<vi>, "Ref Y":refnum<vi>})
            n414 = property class="DigNum (strict)"(reference=w887, error in=w897) -> (error out=w883:errorcluster, "Value"=w885:dbl)  [unwired: 1 out]
            n415 = Bundle By Name(cluster=w891, "active ccd"=w888, "active man refs"=w900) -> (w904:T35)
            n416 = property on="Position 1" class="DigNum (strict)"(error in=w883, "Value"=w885) -> (error out=w882:errorcluster)  [unwired: 1 in, 1 out]
            n417 = property class="DigNum (strict)"(reference=w886, error in=w882) -> (error out=w881:errorcluster, "Value"=w884:dbl)  [unwired: 1 out]
            n418 = property on="Position 2" class="DigNum (strict)"(error in=w881, "Value"=w884) -> (error out=w899:errorcluster)  [unwired: 1 in, 1 out]
          }
          frame "Detection Config" {
            # "Your code here.\n(You can make a copy of, or modify, this frame)"
            n419 = Unbundle By Name(w915) -> ("detection para"=w911:T3[], "active ccd"=w916:i32)
            n420 = Replace Array Subset(array=w911, new element="beam detection para", index=w916) -> (w912:T3[])
            n421 = Bundle By Name(cluster=w915, "detection para"=w912) -> (w914:T35)
            n422 = call <vilib>:"Add State(s) to Queue__jki_lib_state_machine.vi"("State(s) in (\"\")"=w919) -> ("States Out"=w918:string)  [unwired: 14 in]
          }
          frame "Motor Config" {
            # "Your code here.\n(You can make a copy of, or modify, this frame)"
            n423 = Unbundle By Name("associated motors") -> ("Motor CCD 1"=w936:u16, "Motor CCD 2"=w937:u16, "Motor CCD 3"=w938:u16, "Motor CCD 4"=w931:u16, "Motor CCD 5"=w930:u16, "Motor CCD 6"=w929:u16, "Motor CCD 7"=w928:u16, "Motor CCD 8"=w927:u16, "Motor CCD 9"=w926:u16, "Motor CCD 10"=w925:u16, "Motor CCD 11"=w924:u16, "Motor CCD 12"=w923:u16)
            n424 = Build Array(w936, w937, w938, w931, w930, w929, w928, w927, w926, w925, w924, w923) -> (w922:u16[])
            n425 = local read "motor refs"() -> (w934:refnum<vi>[])
            n426 = Increment(x=w922) -> (x+1=w921:u16[])
            n427 = for {
              tunnel: w921 -> [w953] mode=indexing
              tunnel: w934 -> [w948]
              tunnel: [w942] -> w920 mode=indexing
              n428 = Multiply(x=w953, y=u16 2) -> (x*y=w949:u16)
              n429 = Subtract(x=w949, y=u16 2) -> (x-y=w947:u16)
              n430 = Subtract(x=w949, y=u16 1) -> (x-y=w946:u16)
              n431 = Index Array(array=w948, index=w947) -> (element=w945:refnum<vi>)
              n432 = Index Array(array=w948, index=w946) -> (element=w944:refnum<vi>)
              n433 = Bundle By Name(cluster="active Axis ref", "Ref X"=w945, "Ref Y"=w944) -> (w942:cluster{"Ref X":refnum<vi>, "Ref Y":refnum<vi>})
            }
            n434 = call <vilib>:"Add State(s) to Queue__jki_lib_state_machine.vi"("State(s) in (\"\")"=w941) -> ("States Out"=w940:string)  [unwired: 14 in]
            n435 = Bundle By Name(cluster=w933, "active axis refs 2"=w920) -> (w932:T35)
          }
          frame "Move Config" {
            # "Your code here.\n(You can make a copy of, or modify, this frame)"
            n436 = Unbundle By Name(w955) -> ("move properties"=w959:T2[], "active ccd"=w958:i32)
            n437 = Replace Array Subset(array=w959, new element="move config", index=w958) -> (w956:T2[])
            n438 = Bundle By Name(cluster=w955, "move properties"=w956) -> (w954:T35)
            n439 = call <vilib>:"Add State(s) to Queue__jki_lib_state_machine.vi"("State(s) in (\"\")"=w962) -> ("States Out"=w961:string)  [unwired: 14 in]
          }
          frame "----------Centroid & Move----------" {
            # "Template Separator\n(You can make a copy of, or modify, this frame)"
            n440 = call <vilib>:"Add State(s) to Queue__jki_lib_state_machine.vi"("State(s) in (\"\")"=w966) -> ("States Out"=w965:string)  [unwired: 14 in]
          }
          frame "detected" {
            n441 = Unbundle By Name(w974) -> ("Offset X"=w1006:dbl[][], "Offset Y"=w1005:dbl[][], "Size"=w1004:dbl[][], "Mean Size"=w1003:dbl[][], "Time"=w1000:timestamp[][], "Motor X"=w983:dbl[][], "active axis refs 2"=w982:T11, "Motor Y"=w981:dbl[][])
            n442 = Spreadsheet String To Array(format string="%s", spreadsheet string=w986, array type (2D Dbl)=string[] []) -> (array=w977:string[])  [unwired: 1 in]
            n443 = for {
              tunnel: w978 -> [w1019] mode=indexing
              tunnel: w977 -> [w1018]
              tunnel: [w1017] -> w976 mode=indexing
              n444 = for {
                tunnel: w1019 -> [w1022]
                tunnel: [w1021] -> w1016 mode=indexing
                tunnel: w1018 -> [w1020] mode=indexing
                n445 = Equal?(x=w1022, y=w1020) -> (x = y?=w1021:bool)
              }
              n446 = Or Array Elements(Boolean array=w1016) -> (logical OR=w1017:bool)
            }
            n447 = Unbundle By Name(w974) -> ("Mean Centroid X"=w1010:dbl[][], "Mean Centroid Y"=w1009:dbl[][], "Centroid X"=w1012:dbl[][], "Centroid Y"=w1011:dbl[][])
            n448 = call <vilib>:"Add State(s) to Queue__jki_lib_state_machine.vi"("State(s) in (\"\")"=w985) -> ("States Out"=w984:string)  [unwired: 14 in]
            n449 = for {
              tunnel: w1012 -> [w1072]
              tunnel: w1011 -> [w1071]
              tunnel: w1010 -> [w1070]
              tunnel: w1009 -> [w1069]
              tunnel: [w1068] -> w997 mode=indexing
              tunnel: [w1067] -> w1008 mode=indexing
              tunnel: w1007 -> [w1066] mode=indexing
              tunnel: w1006 -> [w1065]
              tunnel: w1005 -> [w1064]
              tunnel: [w1063] -> w975 mode=indexing
              tunnel: [w1062] -> w998 mode=indexing
              tunnel: w1004 -> [w1061]
              tunnel: w1003 -> [w1060]
              tunnel: [w1059] -> w1002 mode=indexing
              tunnel: w1000 -> [w1058]
              tunnel: [w1057] -> w999 mode=indexing
              tunnel: w983 -> [w1049]
              tunnel: w982 -> [w1048]
              tunnel: w981 -> [w1047]
              tunnel: [w1027] -> w980 mode=indexing
              tunnel: [w1026] -> w979 mode=indexing
              tunnel: w976 -> [w1025]
              i -> [w1024]
              n450 = Unbundle By Name(w1066) -> ("Target.X::12"=w1031:refnum<vi>, "Target.Y::12"=w1030:refnum<vi>)
              n451 = Index Array(array=w1049, index (row)=w1024) -> (element=w1052:dbl[])  [unwired: 1 in]
              n452 = Index Array(array=w1048, index=w1024) -> (element=w1051:cluster{"Ref X":refnum<vi>, "Ref Y":refnum<vi>})
              n453 = Index Array(array=w1047, index (row)=w1024) -> (element=w1056:dbl[])  [unwired: 1 in]
              n454 = Index Array(array=w1025, index=w1024) -> (element=w1023:bool)
              n455 = Index Array(array=w1070, index (row)=w1024) -> (element=w1043:dbl[])  [unwired: 1 in]
              n456 = Index Array(array=w1069, index (row)=w1024) -> (element=w1044:dbl[])  [unwired: 1 in]
              n457 = Index Array(array=w1072, index (row)=w1024) -> (element=w1046:dbl[])  [unwired: 1 in]
              n458 = Index Array(array=w1071, index (row)=w1024) -> (element=w1045:dbl[])  [unwired: 1 in]
              n459 = Index Array(array=w1065, index (row)=w1024) -> (element=w1039:dbl[])  [unwired: 1 in]
              n460 = Index Array(array=w1064, index (row)=w1024) -> (element=w1038:dbl[])  [unwired: 1 in]
              n461 = Index Array(array=w1061, index (row)=w1024) -> (element=w1036:dbl[])  [unwired: 1 in]
              n462 = Index Array(array=w1060, index (row)=w1024) -> (element=w1035:dbl[])  [unwired: 1 in]
              n463 = Index Array(array=w1058, index (row)=w1024) -> (element=w1032:timestamp[])  [unwired: 1 in]
              n464 = Unbundle By Name(w1051) -> ("Ref X"=w1050:refnum<vi>, "Ref Y"=w1054:refnum<vi>)
              n465 = property class="DigNum (strict)"(reference=w1031) -> ("Value"=w1029:dbl)  [unwired: 1 in, 2 out]
              n466 = property class="DigNum (strict)"(reference=w1030) -> ("Value"=w1028:dbl)  [unwired: 1 in, 2 out]
              n467 = call <vilib>:"Std Deviation and Variance.vi"("X"=w1046) -> ("mean"=w1042:dbl)  [unwired: 1 in, 2 out]
              n468 = call <vilib>:"Std Deviation and Variance.vi"("X"=w1045) -> ("mean"=w1041:dbl)  [unwired: 1 in, 2 out]
              n469 = call <vilib>:"Std Deviation and Variance.vi"("X"=w1036) -> ("mean"=w1034:dbl)  [unwired: 1 in, 2 out]
              n470 = Get Date/Time In Seconds() -> (seconds since 1Jan1904=w1033:timestamp)
              n471 = property class="DigNum (strict)"(reference=w1050) -> ("Value"=w1053:dbl)  [unwired: 1 in, 2 out]
              n472 = property class="DigNum (strict)"(reference=w1054) -> ("Value"=w1055:dbl)  [unwired: 1 in, 2 out]
              n473 = Subtract(x=w1029, y=w1042) -> (x-y=w1040:dbl)
              n474 = Subtract(x=w1028, y=w1041) -> (x-y=w1037:dbl)
              n475 = case shown="True" w1023 {
                tunnel: [w1085 w1104] -> w1068
                tunnel: [w1073 w1103] -> w1067
                tunnel: [w1074 w1102] -> w1063
                tunnel: [w1075 w1101] -> w1062
                tunnel: [w1076 w1100] -> w1059
                tunnel: [w1077 w1099] -> w1057
                tunnel: w1044 -> [w1083 w1098]
                tunnel: w1043 -> [w1084 w1097]
                tunnel: w1042 -> [_ w1096]
                tunnel: w1041 -> [_ w1095]
                tunnel: w1040 -> [_ w1094]
                tunnel: w1039 -> [w1082 w1093]
                tunnel: w1038 -> [w1081 w1092]
                tunnel: w1037 -> [_ w1091]
                tunnel: w1035 -> [w1080 w1090]
                tunnel: w1034 -> [_ w1089]
                tunnel: w1033 -> [w1078 w1088]
                tunnel: w1032 -> [w1079 w1087]
                frame False {
                  w1086 = 0.0
                  n476 = Build Array (concatenate)(w1084, w1086) -> (w1085:dbl[])
                  n477 = Build Array (concatenate)(w1083, w1086) -> (w1073:dbl[])
                  n478 = Build Array (concatenate)(w1082, w1086) -> (w1074:dbl[])
                  n479 = Build Array (concatenate)(w1081, w1086) -> (w1075:dbl[])
                  n480 = Build Array (concatenate)(w1080, w1086) -> (w1076:dbl[])
                  n481 = Build Array (concatenate)(w1079, w1078) -> (w1077:timestamp[])
                }
                frame True {
                  n482 = Build Array (concatenate)(w1097, w1096) -> (w1104:dbl[])
                  n483 = Build Array (concatenate)(w1098, w1095) -> (w1103:dbl[])
                  n484 = Build Array (concatenate)(w1093, w1094) -> (w1102:dbl[])
                  n485 = Build Array (concatenate)(w1092, w1091) -> (w1101:dbl[])
                  n486 = Build Array (concatenate)(w1090, w1089) -> (w1100:dbl[])
                  n487 = Build Array (concatenate)(w1087, w1088) -> (w1099:timestamp[])
                }
              }
              n488 = Build Array (concatenate)(w1052, w1053) -> (w1027:dbl[])
              n489 = Build Array (concatenate)(w1056, w1055) -> (w1026:dbl[])
            }
            n490 = local write "Numeric"(0.0 ("Numeric")) -> ()
            n491 = Array Size(array=w975) -> (size(s)=w996:i32[])
            n492 = Index Array(array=w996, index=1) -> (element=w994:i32)
            "History Index" <- w994
            n493 = call <vilib>:"Add State(s) to Queue__jki_lib_state_machine.vi"("State(s) in (\"\")"=w984, "State(s) at Back (\"\")"="Check Move\ntdms" ("State(s) at Back (\"\")")) -> ("States Out"=w988:string)  [unwired: 13 in]
            n494 = Unbundle By Name(w974) -> ("img to avg"=w971:i32)
            n495 = Initialize Array(0.0 ("element"), 12 ("dimension size"), w971) -> (w970:dbl[][])
            n496 = Greater?(x=w994, y="History Size") -> (0:w992:bool)
            n497 = Bundle By Name(cluster=w974, "Centroid X"=w970, "Centroid Y"=w970, "Mean Centroid X"=w997, "Mean Centroid Y"=w1008, "Offset X"=w975, "Offset Y"=w998, "Mean Size"=w1002, "Size"=w970, "Time"=w999, "Motor X"=w980, "Motor Y"=w979) -> (w967:T35)
            n498 = Select(t="history" ("State(s) at Back (\"\")"), s=w992, f="") -> (s? t:f=w989:string)
            n499 = call <vilib>:"Add State(s) to Queue__jki_lib_state_machine.vi"("State(s) in (\"\")"=w988, "State(s) at Back (\"\")"=w989) -> ("States Out"=w969:string)  [unwired: 13 in]
            n500 = call <vilib>:"Add State(s) to Queue__jki_lib_state_machine.vi"("State(s) in (\"\")"=w969) -> ("States Out"=w968:string)  [unwired: 14 in]
          }
          frame "Check Move" {
            (unwired) "Device Ini" ("State(s) in Front (\"\")")
            n501 = Unbundle By Name(w1113) -> ("move properties"=w1123:T2[], "Mean Size"=w1122:dbl[][], "move properties"=w1121:T2[], "Offset X"=w1120:dbl[][], "Offset Y"=w1119:dbl[][], "active cams"=w1118:string[])
            n502 = Unbundle By Name(w1113) -> ("steps speed X"=w1112:dbl[], "steps speed Y"=w1111:dbl[])
            n503 = for {
              tunnel: w1121 -> [w1161]
              tunnel: w1120 -> [w1159]
              tunnel: w1119 -> [w1157]
              tunnel: w1122 -> [w1165]
              tunnel: [w1176] -> w1107 mode=indexing
              tunnel: [w1172] -> w1105 mode=indexing
              tunnel: w1118 -> [w1166] mode=indexing
              tunnel: [w1194] -> w1124 mode=indexing
              tunnel: [w1193] -> w1116 mode=indexing
              tunnel: w1123 -> [w1164]
              tunnel: [w1155] -> w1108 mode=indexing
              tunnel: [w1154] -> w1106 mode=indexing
              tunnel: "Speedmode" -> [w1169]
              tunnel: w1115 -> [w1167]
              shift-right: [w1147] -> w1110
              shift-left: w1112 -> [w1152]
              shift-right: [w1146] -> w1109
              shift-left: w1111 -> [w1151]
              n504 = call-poly <userlib>:"Filter 1D Array__ogtk.vi"("items to filter"=w1166, "array"=w1167) -> ("filtered item indices"=w1168:i32[])  [unwired: 4 in, 1 out]
              n505 = Index Array(array=w1168) -> (element=w1150:i32)  [unwired: 1 in]
              n506 = Index Array(array=w1164, index=w1150) -> (element=w1163:T2)
              n507 = Index Array(array=w1165, index (row)=w1150) -> (element=w1162:dbl[])  [unwired: 1 in]
              n508 = Index Array(array=w1161, index=w1150) -> (element=w1160:T2)
              n509 = Index Array(array=w1159, index (row)=w1150) -> (element=w1158:dbl[])  [unwired: 1 in]
              n510 = Index Array(array=w1157, index (row)=w1150) -> (element=w1156:dbl[])  [unwired: 1 in]
              n511 = Unbundle By Name(w1160) -> ("Tolerance [%]"=w1187:dbl)
              n512 = Reverse 1D Array(array=w1158) -> (reversed array=w1192:dbl[])
              n513 = Reverse 1D Array(array=w1156) -> (reversed array=w1191:dbl[])
              n514 = Reverse 1D Array(array=w1162) -> (reversed array=w1186:dbl[])
              n515 = Unbundle By Name(w1163) -> ("Stepsize"=w1145:dbl, "enable feedback"=w1175:bool)
              n516 = Index Array(array=w1192) -> (element=w1190:dbl)  [unwired: 1 in]
              n517 = Index Array(array=w1191) -> (element=w1189:dbl)  [unwired: 1 in]
              n518 = Index Array(array=w1186) -> (element=w1185:dbl)  [unwired: 1 in]
              n519 = Absolute Value(x=w1190) -> (abs(x)=w1153:dbl)
              n520 = Absolute Value(x=w1189) -> (abs(x)=w1171:dbl)
              n521 = Square Root(x=w1185) -> (sqrt(x)=w1184:dbl)
              n522 = Divide(x=w1187, y=100.0) -> (x/y=w1183:dbl)
              n523 = Multiply(x=w1184, y=w1183) -> (x*y=w1170:dbl)
              n524 = Not Equal To 0?(x=w1171) -> (x != 0?=w1173:bool)
              n525 = Not Equal To 0?(x=w1153) -> (x != 0?=w1178:bool)
              n526 = Greater Or Equal?(x=w1153, y=w1170) -> (x >= y?=w1177:bool)
              n527 = Greater Or Equal?(x=w1171, y=w1170) -> (x >= y?=w1174:bool)
              n528 = call "speedmode.vi"("offset X"=w1153, "offset Y"=w1171, "beamsize x tolerance"=w1170, "Speedmode @"=w1169, "step size"=w1145) -> ("steps speed Y"=w1148:dbl, "steps speed X"=w1149:dbl, "speedmode X"=w1155:bool, "speedmode Y"=w1154:bool)  [unwired: 3 in]
              n529 = Compound Arithmetic op=AND(w1175, w1178, w1177) -> (w1176:bool)
              n530 = Compound Arithmetic op=AND(w1175, w1174, w1173) -> (w1172:bool)
              n531 = Boolean To (0,1)(Boolean=w1172) -> (0, 1=w1179:i16)
              n532 = Multiply(x=w1179, y=w1171) -> (x*y=w1180:dbl)
              n533 = Boolean To (0,1)(Boolean=w1176) -> (0, 1=w1182:i16)
              n534 = Replace Array Subset(array=w1152, new element=w1149, index=w1150) -> (w1147:dbl[])
              n535 = Replace Array Subset(array=w1151, new element=w1148, index=w1150) -> (w1146:dbl[])
              n536 = Multiply(x=w1182, y=w1153) -> (x*y=w1181:dbl)
              n537 = Bundle(w1180, "GUIdevice 8"=w1166) -> (w1193:cluster{dbl, "GUIdevice 8":string})  [unwired: 1 in]
              n538 = Bundle(w1181, "GUIdevice 8"=w1166) -> (w1194:cluster{dbl, "GUIdevice 8":string})  [unwired: 1 in]
            }
            "required X" <- w1107
            "required Y" <- w1105
            "speedmode X" <- w1108
            "speedmode Y" <- w1106
            n539 = case shown="False" "Align" {
              tunnel: w1124 -> [w1200 w1205]
              tunnel: w1116 -> [w1199 w1202]
              tunnel: [w1198 w1204] -> w1127
              tunnel: [w1197 w1201] -> w1126
              frame False {
                n540 = Sort 1D Array(array=w1199) -> (sorted array=w1196:cluster{dbl, "GUIdevice 8":string}[])
                n541 = Sort 1D Array(array=w1200) -> (sorted array=w1195:cluster{dbl, "GUIdevice 8":string}[])
                n542 = Reverse 1D Array(array=w1196) -> (reversed array=w1197:cluster{dbl, "GUIdevice 8":string}[])
                n543 = Reverse 1D Array(array=w1195) -> (reversed array=w1198:cluster{dbl, "GUIdevice 8":string}[])
              }
              frame True {
                w1203 = cluster{dbl, "GUIdevice 8":string}[] [] ("Array")
                n544 = for {
                  shift-right: [w1215] -> w1204
                  shift-left: w1203 -> [w1217]
                  tunnel: w1205 -> [w1216] mode=indexing
                  n545 = Unbundle(w1216) -> (w1219:dbl)  [unwired: 1 out]
                  n546 = Not Equal To 0?(x=w1219) -> (x != 0?=w1218:bool)
                  n547 = case shown="True" w1218 {
                    tunnel: w1217 -> [w1220 w1223]
                    tunnel: w1216 -> [_ w1222]
                    tunnel: [w1220 w1221] -> w1215
                    frame False {
                    }
                    frame True {
                      n548 = Build Array (concatenate)(w1223, w1222) -> (w1221:cluster{dbl, "GUIdevice 8":string}[])
                    }
                  }
                }
                n549 = for {
                  shift-right: [w1206] -> w1201
                  shift-left: w1203 -> [w1208]
                  tunnel: w1202 -> [w1207] mode=indexing
                  n550 = Unbundle(w1207) -> (w1210:dbl)  [unwired: 1 out]
                  n551 = Not Equal To 0?(x=w1210) -> (x != 0?=w1209:bool)
                  n552 = case shown="True" w1209 {
                    tunnel: w1208 -> [w1211 w1214]
                    tunnel: w1207 -> [_ w1213]
                    tunnel: [w1211 w1212] -> w1206
                    frame False {
                    }
                    frame True {
                      n553 = Build Array (concatenate)(w1214, w1213) -> (w1212:cluster{dbl, "GUIdevice 8":string}[])
                    }
                  }
                }
              }
            }
            n554 = call <vilib>:"Add State(s) to Queue__jki_lib_state_machine.vi"("State(s) in (\"\")"=w1130) -> ("States Out"=w1129:string)  [unwired: 14 in]
            n555 = Bundle By Name(cluster=w1113, "speedmode X"=w1108, "speedmode Y"=w1106, "steps speed X"=w1110, "steps speed Y"=w1109) -> (w1114:T35)
            n556 = Index Array(array=w1126) -> (element=w1131:cluster{dbl, "GUIdevice 8":string})  [unwired: 1 in]
            n557 = Index Array(array=w1127) -> (element=w1132:cluster{dbl, "GUIdevice 8":string})  [unwired: 1 in]
            n558 = Empty Array?(array=w1126) -> (empty?=w1134:bool)
            n559 = Unbundle(w1132) -> (w1140:dbl)  [unwired: 1 out]
            n560 = Unbundle(w1131) -> (w1136:dbl)  [unwired: 1 out]
            n561 = Unbundle By Name(w1114) -> ("Feedback global"=w1141:bool)
            n562 = Empty Array?(array=w1127) -> (empty?=w1138:bool)
            n563 = property on="autodetect" class="Bool (strict)"("Value"=FALSE ("autodetect")) -> ()  [unwired: 2 in, 2 out]
            n564 = Equal To 0?(x=w1140) -> (x = 0?=w1139:bool)
            n565 = Equal To 0?(x=w1136) -> (x = 0?=w1135:bool)
            n566 = Or(x=w1139, y=w1138) -> (x .or. y?=w1137:bool)
            n567 = Or(x=w1135, y=w1134) -> (x .or. y?=w1133:bool)
            n568 = case shown="True" w1141 {
              tunnel: w1137 -> [_ w1242]
              tunnel: w1127 -> [_ w1241]
              tunnel: w1133 -> [_ w1239]
              tunnel: w1126 -> [_ w1238]
              tunnel: w1129 -> [w1224 w1237]
              tunnel: [w1224 w1236] -> w1142
              tunnel: w1108 -> [_ w1235]
              tunnel: w1107 -> [_ w1234]
              tunnel: w1106 -> [_ w1233]
              tunnel: w1105 -> [_ w1232]
              frame False {
              }
              frame True {
                n569 = case shown="False" w1242 {
                  tunnel: w1241 -> [w1266 _]
                  tunnel: w1237 -> [w1262 w1267]
                  tunnel: [w1260 w1267] -> w1240
                  frame False {
                    n570 = Index Array(array=w1266) -> (element=w1265:cluster{dbl, "GUIdevice 8":string})  [unwired: 1 in]
                    n571 = Unbundle By Name(w1265) -> ("GUIdevice 8"=w1264:string)
                    n572 = call <vilib>:"Build State String with Arguments__jki_lib_state_machine.vi"("Arguments (\"\")"=w1264, "State"="Move X") -> ("State with Arguments"=w1261:string)  [unwired: 4 in]
                    n573 = call <vilib>:"Add State(s) to Queue__jki_lib_state_machine.vi"("State(s) in (\"\")"=w1262, "State(s) at Back (\"\")"=w1261) -> ("States Out"=w1260:string)  [unwired: 13 in]
                  }
                  frame True {
                  }
                }
                n574 = case shown="False" w1239 {
                  tunnel: w1238 -> [w1258 _]
                  tunnel: w1240 -> [w1254 w1259]
                  tunnel: [w1252 w1259] -> w1236
                  frame False {
                    n575 = Index Array(array=w1258) -> (element=w1257:cluster{dbl, "GUIdevice 8":string})  [unwired: 1 in]
                    n576 = Unbundle By Name(w1257) -> ("GUIdevice 8"=w1256:string)
                    n577 = call <vilib>:"Build State String with Arguments__jki_lib_state_machine.vi"("Arguments (\"\")"=w1256, "State"="Move Y") -> ("State with Arguments"=w1253:string)  [unwired: 4 in]
                    n578 = call <vilib>:"Add State(s) to Queue__jki_lib_state_machine.vi"("State(s) in (\"\")"=w1254, "State(s) at Back (\"\")"=w1253) -> ("States Out"=w1252:string)  [unwired: 13 in]
                  }
                  frame True {
                  }
                }
                n579 = for {
                  tunnel: w1235 -> [w1251] mode=indexing
                  tunnel: w1234 -> [w1250] mode=indexing
                  tunnel: [w1249] -> w1231 mode=indexing
                  n580 = And(x=w1251, y=w1250) -> (x .and. y?=w1249:bool)
                }
                n581 = for {
                  tunnel: w1233 -> [w1248] mode=indexing
                  tunnel: w1232 -> [w1247] mode=indexing
                  tunnel: [w1246] -> w1230 mode=indexing
                  n582 = And(x=w1248, y=w1247) -> (x .and. y?=w1246:bool)
                }
                n583 = Or Array Elements(Boolean array=w1231) -> (logical OR=w1229:bool)
                n584 = Or Array Elements(Boolean array=w1230) -> (logical OR=w1228:bool)
                n585 = Or(x=w1229, y=w1228) -> (x .or. y?=w1227:bool)
                n586 = property on="alarms" class="Bool (strict)"() -> ("Value"=w1226:bool)  [unwired: 2 in, 2 out]
                n587 = And(x=w1226, y=w1227) -> (x .and. y?=w1225:bool)
                n588 = case shown="True" w1225 {
                  frame False {
                  }
                  frame True {
                    n589 = call <vilib>:"Beep.vi"("use system alert? (T)"=FALSE, "duration (msec)"=u32 750, "frequency (Hz)"=u32 750) -> ()  [unwired: 9 in]
                  }
                }
              }
            }
            n590 = call <vilib>:"Add State(s) to Queue__jki_lib_state_machine.vi"("State(s) in (\"\")"=w1129, "State(s) at Back (\"\")"=w1142) -> ("States Out"=w1144:string)  [unwired: 13 in]
          }
          frame "Move X" {
            # "Your code here.\n(You can make a copy of, or modify, this frame)"
            n591 = Unbundle By Name(w1274) -> ("Offset X"=w1291:dbl[][])
            n592 = call-poly <userlib>:"Filter 1D Array__ogtk.vi"("items to filter"=w1278, "array"=w1295) -> ("filtered item indices"=w1282:i32[])  [unwired: 4 in, 1 out]
            n593 = Unbundle By Name(w1274) -> ("active axis refs 2"=w1294:T11, "move properties"=w1276:T2[])
            n594 = for {
              tunnel: w1282 -> [w1300] mode=indexing
              tunnel: w1276 -> [w1304]
              shift-right: [w1299] -> w1280
              shift-left: i32[] [] ("filtered item indices") -> [w1302]
              n595 = Index Array(array=w1304, index=w1300) -> (element=w1303:T2)
              n596 = Unbundle By Name(w1303) -> ("enable feedback"=w1301:bool)
              n597 = case shown="True" w1301 {
                tunnel: w1302 -> [w1305 w1308]
                tunnel: w1300 -> [_ w1307]
                tunnel: [w1305 w1306] -> w1299
                frame False {
                }
                frame True {
                  n598 = Build Array (concatenate)(w1308, w1307) -> (w1306:i32[])
                }
              }
            }
            n599 = Index Array(array=w1280) -> (element=w1271:i32)  [unwired: 1 in]
            n600 = Index Array(array=w1291, index (row)=w1271) -> (element=w1290:dbl[])  [unwired: 1 in]
            n601 = Reverse 1D Array(array=w1290) -> (reversed array=w1289:dbl[])
            n602 = Index Array(array=w1294, index=w1271) -> (element=w1293:cluster{"Ref X":refnum<vi>, "Ref Y":refnum<vi>})
            n603 = Index Array(array=w1289) -> (element=w1288:dbl)  [unwired: 1 in]
            n604 = Index Array(array=w1276, index=w1271) -> (element=w1292:T2)
            n605 = Unbundle By Name(w1293) -> ("Ref X"=w1285:refnum<vi>, "Ref Y"=w1284:refnum<vi>)
            n606 = Unbundle By Name(w1292) -> ("Invert Direction X"=w1286:bool, "Invert Axis"=w1275:bool, "enable feedback"=w1283:bool)
            n607 = Greater Or Equal To 0?(x=w1288) -> (x >= 0?=w1287:bool)
            n608 = Unbundle By Name(w1274) -> ("steps speed Y"=w1273:dbl[], "steps speed X"=w1272:dbl[])
            n609 = Index Array(array=w1272, index=w1271) -> (element=w1269:dbl)
            n610 = Index Array(array=w1273, index=w1271) -> (element=w1270:dbl)
            n611 = Select(t=w1270, s=w1275, f=w1269) -> (s? t:f=w1268:dbl)
            n612 = case shown="True" w1283 {
              tunnel: w1275 -> [_ w1314]
              tunnel: w1287 -> [_ w1313]
              tunnel: w1268 -> [_ w1312]
              tunnel: w1286 -> [_ w1311]
              tunnel: w1285 -> [_ w1310]
              tunnel: w1284 -> [_ w1309]
              frame False {
              }
              frame True {
                n613 = case shown="True" w1313 {
                  tunnel: w1311 -> [w1322 w1344]
                  tunnel: w1312 -> [w1320 w1342]
                  tunnel: w1314 -> [w1319 w1341]
                  tunnel: w1314 -> [w1318 w1340]
                  tunnel: w1310 -> [w1316 w1338]
                  tunnel: w1309 -> [w1315 w1337]
                  frame True {
                    n614 = case shown="True" w1319 {
                      tunnel: [w1333 w1335] -> w1321
                      tunnel: w1316 -> [w1334 _]
                      tunnel: w1315 -> [_ w1336]
                      frame False {
                        n615 = property class="DigNum (strict)"(reference=w1334) -> ("Value"=w1333:dbl)  [unwired: 1 in, 2 out]
                      }
                      frame True {
                        n616 = property class="DigNum (strict)"(reference=w1336) -> ("Value"=w1335:dbl)  [unwired: 1 in, 2 out]
                      }
                    }
                    n617 = case shown="True" w1322 {
                      tunnel: w1321 -> [w1329 w1332]
                      tunnel: w1320 -> [w1328 w1331]
                      tunnel: [w1327 w1330] -> w1317
                      frame False {
                        n618 = Add(x=w1329, y=w1328) -> (x+y=w1327:dbl)
                      }
                      frame True {
                        n619 = Subtract(x=w1332, y=w1331) -> (x-y=w1330:dbl)
                      }
                    }
                    n620 = case shown="True" w1318 {
                      tunnel: w1317 -> [w1323 w1325]
                      tunnel: w1316 -> [w1324 _]
                      tunnel: w1315 -> [_ w1326]
                      frame False {
                        n621 = property class="DigNum (strict)"(reference=w1324, "Val(Sgnl)"=w1323) -> ()  [unwired: 1 in, 2 out]
                      }
                      frame True {
                        n622 = property class="DigNum (strict)"(reference=w1326, "Val(Sgnl)"=w1325) -> ()  [unwired: 1 in, 2 out]
                      }
                    }
                  }
                  frame False {
                    n623 = case shown="False" w1341 {
                      tunnel: [w1355 w1357] -> w1343
                      tunnel: w1338 -> [w1356 _]
                      tunnel: w1337 -> [_ w1358]
                      frame False {
                        n624 = property class="DigNum (strict)"(reference=w1356) -> ("Value"=w1355:dbl)  [unwired: 1 in, 2 out]
                      }
                      frame True {
                        n625 = property class="DigNum (strict)"(reference=w1358) -> ("Value"=w1357:dbl)  [unwired: 1 in, 2 out]
                      }
                    }
                    n626 = case shown="False" w1344 {
                      tunnel: w1343 -> [w1351 w1354]
                      tunnel: w1342 -> [w1350 w1353]
                      tunnel: [w1349 w1352] -> w1339
                      frame False {
                        n627 = Subtract(x=w1351, y=w1350) -> (x-y=w1349:dbl)
                      }
                      frame True {
                        n628 = Add(x=w1354, y=w1353) -> (x+y=w1352:dbl)
                      }
                    }
                    n629 = case shown="False" w1340 {
                      tunnel: w1339 -> [w1345 w1347]
                      tunnel: w1338 -> [w1346 _]
                      tunnel: w1337 -> [_ w1348]
                      frame False {
                        n630 = property class="DigNum (strict)"(reference=w1346, "Val(Sgnl)"=w1345) -> ()  [unwired: 1 in, 2 out]
                      }
                      frame True {
                        n631 = property class="DigNum (strict)"(reference=w1348, "Val(Sgnl)"=w1347) -> ()  [unwired: 1 in, 2 out]
                      }
                    }
                  }
                }
              }
            }
            n632 = call <vilib>:"Build State String with Arguments__jki_lib_state_machine.vi"("Arguments (\"\")"=w1278, "State"="Wait" ("State(s) in Front (\"\")")) -> ("State with Arguments"=w1277:string)  [unwired: 4 in]
            n633 = call <vilib>:"Add State(s) to Queue__jki_lib_state_machine.vi"("State(s) in Front (\"\")"=w1277, "State(s) in (\"\")"=w1298) -> ("States Out"=w1297:string)  [unwired: 13 in]
            "Moving X" <- w1278
          }
          frame "ManMove X" {
            # "Your code here.\n(You can make a copy of, or modify, this frame)"
            n634 = Equal?(x=w1364, y="Right") -> (x = y?=w1365:bool)
            n635 = Unbundle By Name(w1374) -> ("move properties"=w1369:T2[], "active ccd"=w1362:i32, "active man refs"=w1367:cluster{"Ref X":refnum<vi>, "Ref Y":refnum<vi>}, "active cams"=w1363:string[])
            n636 = Index Array(array=w1363, index=w1362) -> (element=w1360:string)
            n637 = Index Array(array=w1369, index=w1362) -> (element=w1375:T2)
            n638 = Unbundle By Name(w1367) -> ("Ref X"=w1371:refnum<vi>, "Ref Y"=w1370:refnum<vi>)
            n639 = Unbundle By Name(w1375) -> ("Invert Direction X"=w1372:bool, "Invert Axis"=w1373:bool)
            n640 = call <vilib>:"Build State String with Arguments__jki_lib_state_machine.vi"("Arguments (\"\")"=w1360, "State"="Wait" ("State(s) in Front (\"\")")) -> ("State with Arguments"=w1359:string)  [unwired: 4 in]
            n641 = call <vilib>:"Add State(s) to Queue__jki_lib_state_machine.vi"("State(s) in Front (\"\")"=w1359, "State(s) in (\"\")"=w1378) -> ("States Out"=w1377:string)  [unwired: 13 in]
            n642 = case shown="False" w1365 {
              tunnel: w1372 -> [w1386 w1408]
              tunnel: "StepSize" -> [w1384 w1406]
              tunnel: w1373 -> [w1383 w1405]
              tunnel: w1373 -> [w1382 w1404]
              tunnel: w1371 -> [w1380 w1402]
              tunnel: w1370 -> [w1379 w1401]
              frame True {
                n643 = case shown="False" w1383 {
                  tunnel: [w1397 w1399] -> w1385
                  tunnel: w1380 -> [w1398 _]
                  tunnel: w1379 -> [_ w1400]
                  frame False {
                    n644 = property class="DigNum (strict)"(reference=w1398) -> ("Value"=w1397:dbl)  [unwired: 1 in, 2 out]
                  }
                  frame True {
                    n645 = property class="DigNum (strict)"(reference=w1400) -> ("Value"=w1399:dbl)  [unwired: 1 in, 2 out]
                  }
                }
                n646 = case shown="False" w1386 {
                  tunnel: w1385 -> [w1393 w1396]
                  tunnel: w1384 -> [w1392 w1395]
                  tunnel: [w1391 w1394] -> w1381
                  frame False {
                    n647 = Add(x=w1393, y=w1392) -> (x+y=w1391:dbl)
                  }
                  frame True {
                    n648 = Subtract(x=w1396, y=w1395) -> (x-y=w1394:dbl)
                  }
                }
                n649 = case shown="False" w1382 {
                  tunnel: w1381 -> [w1387 w1389]
                  tunnel: w1380 -> [w1388 _]
                  tunnel: w1379 -> [_ w1390]
                  frame False {
                    n650 = property class="DigNum (strict)"(reference=w1388, "Val(Sgnl)"=w1387) -> ()  [unwired: 1 in, 2 out]
                  }
                  frame True {
                    n651 = property class="DigNum (strict)"(reference=w1390, "Val(Sgnl)"=w1389) -> ()  [unwired: 1 in, 2 out]
                  }
                }
              }
              frame False {
                n652 = case shown="True" w1405 {
                  tunnel: [w1419 w1421] -> w1407
                  tunnel: w1402 -> [w1420 _]
                  tunnel: w1401 -> [_ w1422]
                  frame False {
                    n653 = property class="DigNum (strict)"(reference=w1420) -> ("Value"=w1419:dbl)  [unwired: 1 in, 2 out]
                  }
                  frame True {
                    n654 = property class="DigNum (strict)"(reference=w1422) -> ("Value"=w1421:dbl)  [unwired: 1 in, 2 out]
                  }
                }
                n655 = case shown="True" w1408 {
                  tunnel: w1407 -> [w1415 w1418]
                  tunnel: w1406 -> [w1414 w1417]
                  tunnel: [w1413 w1416] -> w1403
                  frame False {
                    n656 = Subtract(x=w1415, y=w1414) -> (x-y=w1413:dbl)
                  }
                  frame True {
                    n657 = Add(x=w1418, y=w1417) -> (x+y=w1416:dbl)
                  }
                }
                n658 = case shown="False" w1404 {
                  tunnel: w1403 -> [w1409 w1411]
                  tunnel: w1402 -> [w1410 _]
                  tunnel: w1401 -> [_ w1412]
                  frame False {
                    n659 = property class="DigNum (strict)"(reference=w1410, "Val(Sgnl)"=w1409) -> ()  [unwired: 1 in, 2 out]
                  }
                  frame True {
                    n660 = property class="DigNum (strict)"(reference=w1412, "Val(Sgnl)"=w1411) -> ()  [unwired: 1 in, 2 out]
                  }
                }
              }
            }
          }
          frame "ManMove Y" {
            # "Your code here.\n(You can make a copy of, or modify, this frame)"
            n661 = Equal?(x=w1428, y="Down") -> (x = y?=w1432:bool)
            n662 = Unbundle By Name(w1438) -> ("active cams"=w1427:string[], "move properties"=w1437:T2[], "active ccd"=w1426:i32, "active man refs"=w1436:cluster{"Ref X":refnum<vi>, "Ref Y":refnum<vi>})
            n663 = Index Array(array=w1427, index=w1426) -> (element=w1424:string)
            n664 = property on="StepSize" class="DigNum (strict)"() -> ("Value"=w1429:dbl)  [unwired: 2 in, 2 out]
            n665 = Index Array(array=w1437, index=w1426) -> (element=w1439:T2)
            n666 = Unbundle By Name(w1436) -> ("Ref Y"=w1431:refnum<vi>, "Ref X"=w1430:refnum<vi>)
            n667 = Unbundle By Name(w1439) -> ("Invert Direction Y"=w1434:bool, "Invert Axis"=w1433:bool)
            n668 = call <vilib>:"Build State String with Arguments__jki_lib_state_machine.vi"("Arguments (\"\")"=w1424, "State"="Wait" ("State(s) in Front (\"\")")) -> ("State with Arguments"=w1423:string)  [unwired: 4 in]
            n669 = call <vilib>:"Add State(s) to Queue__jki_lib_state_machine.vi"("State(s) in Front (\"\")"=w1423, "State(s) in (\"\")"=w1442) -> ("States Out"=w1441:string)  [unwired: 13 in]
            n670 = case shown="True" w1432 {
              tunnel: w1434 -> [w1450 w1472]
              tunnel: w1429 -> [w1448 w1470]
              tunnel: w1433 -> [w1447 w1469]
              tunnel: w1433 -> [w1446 w1468]
              tunnel: w1431 -> [w1444 w1466]
              tunnel: w1430 -> [w1443 w1465]
              frame True {
                n671 = case shown="True" w1447 {
                  tunnel: [w1461 w1463] -> w1449
                  tunnel: w1444 -> [w1462 _]
                  tunnel: w1443 -> [_ w1464]
                  frame False {
                    n672 = property class="DigNum (strict)"(reference=w1462) -> ("Value"=w1461:dbl)  [unwired: 1 in, 2 out]
                  }
                  frame True {
                    n673 = property class="DigNum (strict)"(reference=w1464) -> ("Value"=w1463:dbl)  [unwired: 1 in, 2 out]
                  }
                }
                n674 = case shown="False" w1450 {
                  tunnel: w1449 -> [w1457 w1460]
                  tunnel: w1448 -> [w1456 w1459]
                  tunnel: [w1455 w1458] -> w1445
                  frame False {
                    n675 = Add(x=w1457, y=w1456) -> (x+y=w1455:dbl)
                  }
                  frame True {
                    n676 = Subtract(x=w1460, y=w1459) -> (x-y=w1458:dbl)
                  }
                }
                n677 = case shown="True" w1446 {
                  tunnel: w1445 -> [w1451 w1453]
                  tunnel: w1444 -> [w1452 _]
                  tunnel: w1443 -> [_ w1454]
                  frame False {
                    n678 = property class="DigNum (strict)"(reference=w1452, "Val(Sgnl)"=w1451) -> ()  [unwired: 1 in, 2 out]
                  }
                  frame True {
                    n679 = property class="DigNum (strict)"(reference=w1454, "Val(Sgnl)"=w1453) -> ()  [unwired: 1 in, 2 out]
                  }
                }
              }
              frame False {
                n680 = case shown="False" w1469 {
                  tunnel: [w1483 w1485] -> w1471
                  tunnel: w1466 -> [w1484 _]
                  tunnel: w1465 -> [_ w1486]
                  frame False {
                    n681 = property class="DigNum (strict)"(reference=w1484) -> ("Value"=w1483:dbl)  [unwired: 1 in, 2 out]
                  }
                  frame True {
                    n682 = property class="DigNum (strict)"(reference=w1486) -> ("Value"=w1485:dbl)  [unwired: 1 in, 2 out]
                  }
                }
                n683 = case shown="False" w1472 {
                  tunnel: w1471 -> [w1479 w1482]
                  tunnel: w1470 -> [w1478 w1481]
                  tunnel: [w1477 w1480] -> w1467
                  frame False {
                    n684 = Subtract(x=w1479, y=w1478) -> (x-y=w1477:dbl)
                  }
                  frame True {
                    n685 = Add(x=w1482, y=w1481) -> (x+y=w1480:dbl)
                  }
                }
                n686 = case shown="False" w1468 {
                  tunnel: w1467 -> [w1473 w1475]
                  tunnel: w1466 -> [w1474 _]
                  tunnel: w1465 -> [_ w1476]
                  frame False {
                    n687 = property class="DigNum (strict)"(reference=w1474, "Val(Sgnl)"=w1473) -> ()  [unwired: 1 in, 2 out]
                  }
                  frame True {
                    n688 = property class="DigNum (strict)"(reference=w1476, "Val(Sgnl)"=w1475) -> ()  [unwired: 1 in, 2 out]
                  }
                }
              }
            }
          }
          frame "Move Y" {
            # "Your code here.\n(You can make a copy of, or modify, this frame)"
            n689 = Unbundle By Name(w1488) -> ("Offset Y"=w1510:dbl[][])
            n690 = call-poly <userlib>:"Filter 1D Array__ogtk.vi"("items to filter"=w1497, "array"=w1514) -> ("filtered item indices"=w1502:i32[])  [unwired: 4 in, 1 out]
            n691 = Unbundle By Name(w1488) -> ("active axis refs 2"=w1513:T11, "move properties"=w1500:T2[])
            n692 = for {
              tunnel: w1502 -> [w1519] mode=indexing
              tunnel: w1500 -> [w1523]
              shift-right: [w1518] -> w1501
              shift-left: i32[] [] ("filtered item indices") -> [w1521]
              n693 = Index Array(array=w1523, index=w1519) -> (element=w1522:T2)
              n694 = Unbundle By Name(w1522) -> ("enable feedback"=w1520:bool)
              n695 = case shown="True" w1520 {
                tunnel: w1521 -> [w1524 w1527]
                tunnel: w1519 -> [_ w1526]
                tunnel: [w1524 w1525] -> w1518
                frame False {
                }
                frame True {
                  n696 = Build Array (concatenate)(w1527, w1526) -> (w1525:i32[])
                }
              }
            }
            n697 = Index Array(array=w1501) -> (element=w1490:i32)  [unwired: 1 in]
            n698 = Index Array(array=w1510, index (row)=w1490) -> (element=w1509:dbl[])  [unwired: 1 in]
            n699 = Reverse 1D Array(array=w1509) -> (reversed array=w1508:dbl[])
            n700 = Index Array(array=w1513, index=w1490) -> (element=w1512:cluster{"Ref X":refnum<vi>, "Ref Y":refnum<vi>})
            n701 = Index Array(array=w1508) -> (element=w1507:dbl)  [unwired: 1 in]
            n702 = Index Array(array=w1500, index=w1490) -> (element=w1511:T2)
            n703 = Unbundle By Name(w1512) -> ("Ref Y"=w1505:refnum<vi>, "Ref X"=w1504:refnum<vi>)
            n704 = Unbundle By Name(w1511) -> ("Invert Direction Y"=w1489:bool, "Invert Axis"=w1495:bool, "enable feedback"=w1503:bool)
            n705 = Greater Or Equal To 0?(x=w1507) -> (x >= 0?=w1506:bool)
            n706 = Unbundle By Name(w1488) -> ("steps speed X"=w1494:dbl[], "steps speed Y"=w1493:dbl[])
            n707 = Index Array(array=w1493, index=w1490) -> (element=w1491:dbl)
            n708 = Index Array(array=w1494, index=w1490) -> (element=w1492:dbl)
            n709 = Select(t=w1492, s=w1489, f=w1491) -> (s? t:f=w1487:dbl)
            n710 = case shown="True" w1503 {
              tunnel: w1495 -> [_ w1533]
              tunnel: w1506 -> [_ w1532]
              tunnel: w1487 -> [_ w1531]
              tunnel: w1489 -> [_ w1530]
              tunnel: w1505 -> [_ w1529]
              tunnel: w1504 -> [_ w1528]
              frame False {
              }
              frame True {
                n711 = case shown="False" w1532 {
                  tunnel: w1530 -> [w1541 w1563]
                  tunnel: w1531 -> [w1539 w1561]
                  tunnel: w1533 -> [w1538 w1560]
                  tunnel: w1533 -> [w1537 w1559]
                  tunnel: w1529 -> [w1535 w1557]
                  tunnel: w1528 -> [w1534 w1556]
                  frame True {
                    n712 = case shown="False" w1538 {
                      tunnel: [w1552 w1554] -> w1540
                      tunnel: w1535 -> [w1553 _]
                      tunnel: w1534 -> [_ w1555]
                      frame False {
                        n713 = property class="DigNum (strict)"(reference=w1553) -> ("Value"=w1552:dbl)  [unwired: 1 in, 2 out]
                      }
                      frame True {
                        n714 = property class="DigNum (strict)"(reference=w1555) -> ("Value"=w1554:dbl)  [unwired: 1 in, 2 out]
                      }
                    }
                    n715 = case shown="False" w1541 {
                      tunnel: w1540 -> [w1548 w1551]
                      tunnel: w1539 -> [w1547 w1550]
                      tunnel: [w1546 w1549] -> w1536
                      frame False {
                        n716 = Add(x=w1548, y=w1547) -> (x+y=w1546:dbl)
                      }
                      frame True {
                        n717 = Subtract(x=w1551, y=w1550) -> (x-y=w1549:dbl)
                      }
                    }
                    n718 = case shown="False" w1537 {
                      tunnel: w1536 -> [w1542 w1544]
                      tunnel: w1535 -> [w1543 _]
                      tunnel: w1534 -> [_ w1545]
                      frame False {
                        n719 = property class="DigNum (strict)"(reference=w1543, "Val(Sgnl)"=w1542) -> ()  [unwired: 1 in, 2 out]
                      }
                      frame True {
                        n720 = property class="DigNum (strict)"(reference=w1545, "Val(Sgnl)"=w1544) -> ()  [unwired: 1 in, 2 out]
                      }
                    }
                  }
                  frame False {
                    n721 = case shown="False" w1560 {
                      tunnel: [w1574 w1576] -> w1562
                      tunnel: w1557 -> [w1575 _]
                      tunnel: w1556 -> [_ w1577]
                      frame False {
                        n722 = property class="DigNum (strict)"(reference=w1575) -> ("Value"=w1574:dbl)  [unwired: 1 in, 2 out]
                      }
                      frame True {
                        n723 = property class="DigNum (strict)"(reference=w1577) -> ("Value"=w1576:dbl)  [unwired: 1 in, 2 out]
                      }
                    }
                    n724 = case shown="False" w1563 {
                      tunnel: w1562 -> [w1570 w1573]
                      tunnel: w1561 -> [w1569 w1572]
                      tunnel: [w1568 w1571] -> w1558
                      frame False {
                        n725 = Subtract(x=w1570, y=w1569) -> (x-y=w1568:dbl)
                      }
                      frame True {
                        n726 = Add(x=w1573, y=w1572) -> (x+y=w1571:dbl)
                      }
                    }
                    n727 = case shown="True" w1559 {
                      tunnel: w1558 -> [w1564 w1566]
                      tunnel: w1557 -> [w1565 _]
                      tunnel: w1556 -> [_ w1567]
                      frame False {
                        n728 = property class="DigNum (strict)"(reference=w1565, "Val(Sgnl)"=w1564) -> ()  [unwired: 1 in, 2 out]
                      }
                      frame True {
                        n729 = property class="DigNum (strict)"(reference=w1567, "Val(Sgnl)"=w1566) -> ()  [unwired: 1 in, 2 out]
                      }
                    }
                  }
                }
              }
            }
            n730 = call <vilib>:"Build State String with Arguments__jki_lib_state_machine.vi"("Arguments (\"\")"=w1497, "State"="Wait" ("State(s) in Front (\"\")")) -> ("State with Arguments"=w1496:string)  [unwired: 4 in]
            n731 = call <vilib>:"Add State(s) to Queue__jki_lib_state_machine.vi"("State(s) in Front (\"\")"=w1496, "State(s) in (\"\")"=w1517) -> ("States Out"=w1516:string)  [unwired: 13 in]
            "Moving Y" <- w1497
          }
          frame "Wait" {
            # "Your code here.\n(You can make a copy of, or modify, this frame)"
            n732 = flat-sequence {
              tunnel: T18."Disabled and Grayed Out" ("Disabled") -> [w1594]
              tunnel: w1584 -> [w1603]
              tunnel: w1583 -> [w1602]
              tunnel: [w1601] -> w1582
              tunnel: w1581 -> [w1600]
              tunnel: w1580 -> [w1599]
              tunnel: T18."Enabled" ("Disabled") -> [w1613]
              frame #0 {
                n733 = property on="Right" class="Bool (strict)"("DisabledEnum"=w1594) -> ()  [unwired: 2 in, 2 out]
                n734 = property on="Up" class="Bool (strict)"("DisabledEnum"=w1594) -> ()  [unwired: 2 in, 2 out]
                n735 = property on="Left" class="Bool (strict)"("DisabledEnum"=w1594) -> ()  [unwired: 2 in, 2 out]
                n736 = property on="Down" class="Bool (strict)"("DisabledEnum"=w1594) -> ()  [unwired: 2 in, 2 out]
                n737 = property on="StepSize" class="DigNum (strict)"("DisabledEnum"=w1594) -> ()  [unwired: 2 in, 2 out]
              }
              frame #1 {
                n738 = Wait (ms)(milliseconds to wait=u32 1500) -> ()  [unwired: 1 out]
              }
              frame #2 {
                n739 = property on="Moving Y" class="Str"("Value"="") -> ()  [unwired: 2 in, 2 out]
                n740 = property on="Moving X" class="Str"("Value"="") -> ()  [unwired: 2 in, 2 out]
              }
              frame #3 {
                n741 = Equal?(x=w1599, y=w1600) -> (x = y?=w1598:bool)
                n742 = case shown="True" w1598 {
                  tunnel: w1603 -> [_ w1610]
                  tunnel: w1602 -> [w1604 w1607]
                  tunnel: [w1604 w1605] -> w1601
                  frame False {
                  }
                  frame True {
                    n743 = Unbundle By Name(w1610) -> ("Ref X"=w1609:refnum<vi>, "Ref Y"=w1608:refnum<vi>)
                    n744 = property class="DigNum (strict)"(reference=w1609, error in=w1607) -> (error out=w1606:errorcluster, "Value"=w1612:dbl)  [unwired: 1 out]
                    n745 = property class="DigNum (strict)"(reference=w1608, error in=w1606) -> (error out=w1605:errorcluster, "Value"=w1611:dbl)  [unwired: 1 out]
                    n746 = property on="Position 1" class="DigNum (strict)"("Value"=w1612) -> ()  [unwired: 2 in, 2 out]
                    n747 = property on="Position 2" class="DigNum (strict)"("Value"=w1611) -> ()  [unwired: 2 in, 2 out]
                  }
                }
              }
              frame #4 {
                n748 = property on="Right" class="Bool (strict)"("DisabledEnum"=w1613) -> ()  [unwired: 2 in, 2 out]
                n749 = property on="Up" class="Bool (strict)"("DisabledEnum"=w1613) -> ()  [unwired: 2 in, 2 out]
                n750 = property on="Left" class="Bool (strict)"("DisabledEnum"=w1613) -> ()  [unwired: 2 in, 2 out]
                n751 = property on="Down" class="Bool (strict)"("DisabledEnum"=w1613) -> ()  [unwired: 2 in, 2 out]
                n752 = property on="StepSize" class="DigNum (strict)"("DisabledEnum"=w1613) -> ()  [unwired: 2 in, 2 out]
              }
            }
            n753 = call-poly <userlib>:"Filter 1D Array__ogtk.vi"("items to filter"=w1587, "array"=w1588) -> ("filtered item indices"=w1586:i32[])  [unwired: 4 in, 1 out]
            n754 = Index Array(array=w1586) -> (element=w1581:i32)  [unwired: 1 in]
            n755 = Unbundle By Name(w1589) -> ("active axis refs 2"=w1585:T11, "active ccd"=w1580:i32)
            n756 = Index Array(array=w1585, index=w1581) -> (element=w1584:cluster{"Ref X":refnum<vi>, "Ref Y":refnum<vi>})
            n757 = call <vilib>:"Add State(s) to Queue__jki_lib_state_machine.vi"("State(s) in (\"\")"=w1593) -> ("States Out"=w1592:string)  [unwired: 14 in]
            n758 = local read "Mean Centroid X"() -> (w1590:dbl[][])
            n759 = Bundle By Name(cluster=w1589, "Mean Centroid X"=w1590, "Mean Centroid Y"=w1590) -> (w1591:T35)
          }
          frame "---------------Statistics--------------" {
            # "Template Separator\n(You can make a copy of, or modify, this frame)"
            n760 = call <vilib>:"Add State(s) to Queue__jki_lib_state_machine.vi"("State(s) in (\"\")"=w1617) -> ("States Out"=w1616:string)  [unwired: 14 in]
          }
          frame "Save Stats" {
            # "Your code here.\n(You can make a copy of, or modify, this frame)"
            n761 = property on="CCD 1" class="XYGraph (strict)"() -> ("Value"=w1628:cluster{timestamp[], dbl[]}[])  [unwired: 2 in, 2 out]
            n762 = property on="CCD 2" class="XYGraph (strict)"() -> ("Value"=w1627:cluster{timestamp[], dbl[]}[])  [unwired: 2 in, 2 out]
            n763 = property on="CCD 3" class="XYGraph (strict)"() -> ("Value"=w1626:cluster{timestamp[], dbl[]}[])  [unwired: 2 in, 2 out]
            n764 = property on="CCD 4" class="XYGraph (strict)"() -> ("Value"=w1625:cluster{timestamp[], dbl[]}[])  [unwired: 2 in, 2 out]
            n765 = property on="CCD 5" class="XYGraph (strict)"() -> ("Value"=w1624:cluster{timestamp[], dbl[]}[])  [unwired: 2 in, 2 out]
            n766 = property on="CCD 6" class="XYGraph (strict)"() -> ("Value"=w1623:cluster{timestamp[], dbl[]}[])  [unwired: 2 in, 2 out]
            n767 = property on="CCD 7" class="XYGraph (strict)"() -> ("Value"=w1622:cluster{timestamp[], dbl[]}[])  [unwired: 2 in, 2 out]
            n768 = property on="CCD 8" class="XYGraph (strict)"() -> ("Value"=w1621:cluster{timestamp[], dbl[]}[])  [unwired: 2 in, 2 out]
            n769 = Build Array(w1628, w1627, w1626, w1625, w1624, w1623, w1622, w1621) -> (w1620:cluster{timestamp[], dbl[]}[][])
            n770 = disable-structure shown="Disabled" {
              disable-tunnel: w1632 -> [w1636 _]
              disable-tunnel: [w1635 _] -> w1631
              disable-tunnel: w1620 -> [w1634 _]
              disable-tunnel: w1619 -> [w1633 _]
              frame Disabled {
                n771 = for {
                  tunnel: w1634 -> [w1639] mode=indexing
                  tunnel: w1633 -> [w1638] mode=indexing
                  n772 = Empty String/Path?(string/path=w1638) -> (empty?=w1637:bool)
                  n773 = case shown="False" w1637 {
                    tunnel: w1639 -> [w1645 _]
                    tunnel: w1638 -> [w1643 _]
                    frame False {
                      n774 = Index Array(array=w1645, index #1=0 ("index"), index #2=1 ("index"), index #3=2 ("index"), index #4=3 ("index")) -> (element #1=w1680:cluster{timestamp[], dbl[]}, element #2=w1674:cluster{timestamp[], dbl[]}, element #3=w1673:cluster{timestamp[], dbl[]}, element #4=w1672:cluster{timestamp[], dbl[]})  [unwired: 1 in, 1 out]
                      n775 = Concatenate Strings(w1643, ".dat" ("string")) -> (w1641:string)
                      n776 = Unbundle(w1680) -> (w1679:timestamp[], w1657:dbl[])
                      n777 = Unbundle(w1674) -> (w1648:dbl[])  [unwired: 1 out]
                      n778 = Unbundle(w1673) -> (w1647:dbl[])  [unwired: 1 out]
                      n779 = Unbundle(w1672) -> (w1646:dbl[])  [unwired: 1 out]
                      n780 = Build Path(base path="save path", name or relative path=w1641) -> (appended path=w1640:path)
                      n781 = for {
                        tunnel: w1679 -> [w1682] mode=indexing
                        tunnel: [w1681] -> w1655 mode=indexing
                        n782 = Format Date/Time String(time format string (%c)="%Y%m%d%H%M%S", seconds (now)=w1682) -> (date/time string=w1681:string)  [unwired: 1 in]
                      }
                      n783 = Array Size(array=w1657) -> (size(s)=w1658:i32)
                      n784 = Number To Fractional String(number=w1657) -> (F-format string=w1654:string[])  [unwired: 3 in]
                      n785 = Number To Fractional String(number=w1648) -> (F-format string=w1651:string[])  [unwired: 3 in]
                      n786 = Number To Fractional String(number=w1647) -> (F-format string=w1650:string[])  [unwired: 3 in]
                      n787 = Number To Fractional String(number=w1646) -> (F-format string=w1649:string[])  [unwired: 3 in]
                      n788 = Initialize Array("", w1658, 5 ("dimension size")) -> (w1656:string[][])
                      n789 = Insert Into Array(array=w1656, index (col)=0 ("disabled index (col)"), new element=w1655) -> (w1666:string[][])  [unwired: 1 in]
                      n790 = Insert Into Array(array=w1666, index (col)=1 ("disabled index (col)"), new element=w1654) -> (w1665:string[][])  [unwired: 1 in]
                      n791 = Insert Into Array(array=w1665, index (col)=2 ("disabled index (col)"), new element=w1651) -> (w1669:string[][])  [unwired: 1 in]
                      n792 = Insert Into Array(array=w1669, index (col)=3 ("disabled index (col)"), new element=w1650) -> (w1670:string[][])  [unwired: 1 in]
                      n793 = Insert Into Array(array=w1670, index (col)=4 ("disabled index (col)"), new element=w1649) -> (w1671:string[][])  [unwired: 1 in]
                      n794 = Insert Into Array(array=w1671, index (row)=0, new element=string[] ["time", "Centroid X", "Centroid Y", "Motor Axis 1", "Motor Axis 2"] ("new element/subarray 2")) -> (w1653:string[][])  [unwired: 1 in]
                      n795 = call-poly <vilib>:"Write To Spreadsheet File.vi"("2D data"=w1653, "file path (dialog if empty)"=w1640) -> ()  [unwired: 6 in, 1 out]
                    }
                    frame True {
                    }
                  }
                }
                n796 = call <vilib>:"Add State(s) to Queue__jki_lib_state_machine.vi"("State(s) in (\"\")"=w1636) -> ("States Out"=w1635:string)  [unwired: 14 in]
              }
              frame Enabled {
              }
            }
            n797 = property on="Save Stats" class="Bool (strict)"("Value"=FALSE ("Save Stats")) -> ()  [unwired: 2 in, 2 out]
          }
          frame "tdms" {
            w1694 = 21600.0 ("new tdms")
            # "Your code here.\n(You can make a copy of, or modify, this frame)"
            n798 = Unbundle By Name(w1702) -> ("active cams"=w1687:string[], "Data Value Reference out"=w1684:refnum<k34>, "Offset X"=w1701:dbl[][], "Offset Y"=w1700:dbl[][], "active axis refs 2"=w1699:T11)
            n799 = for {
              tunnel: w1701 -> [w1749]
              tunnel: w1700 -> [w1748]
              tunnel: w1687 -> [w1712] mode=indexing
              tunnel: w1684 -> [w1713]
              tunnel: w1699 -> [w1734]
              tunnel: w1704 -> [w1718]
              tunnel: [w1716] -> w1703
              i -> [w1735]
              n800 = Index Array(array=w1749, index (row)=w1735) -> (element=w1747:dbl[])  [unwired: 1 in]
              n801 = Index Array(array=w1748, index (row)=w1735) -> (element=w1746:dbl[])  [unwired: 1 in]
              n802 = Index Array(array=w1734, index=w1735) -> (element=w1733:cluster{"Ref X":refnum<vi>, "Ref Y":refnum<vi>})
              n803 = Reverse 1D Array(array=w1746) -> (reversed array=w1744:dbl[])
              n804 = Reverse 1D Array(array=w1747) -> (reversed array=w1745:dbl[])
              n805 = Unbundle By Name(w1733) -> ("Ref X"=w1732:refnum<vi>, "Ref Y"=w1731:refnum<vi>)
              n806 = Index Array(array=w1745) -> (element=w1743:dbl)  [unwired: 1 in]
              n807 = Index Array(array=w1744) -> (element=w1742:dbl)  [unwired: 1 in]
              n808 = property class="DigNum (strict)"(reference=w1732, error in=w1718) -> (error out=w1717:errorcluster, "Value"=w1726:dbl)  [unwired: 1 out]
              n809 = Build Array(w1743) -> (w1715:dbl[])
              n810 = Build Array(w1742) -> (w1737:dbl[])
              n811 = Get Date/Time In Seconds() -> (seconds since 1Jan1904=w1714:timestamp)
              n812 = Build Array(w1714) -> (w1710:timestamp[])
              n813 = property class="DigNum (strict)"(reference=w1731, error in=w1717) -> (error out=w1708:errorcluster, "Value"=w1720:dbl)  [unwired: 1 out]
              n814 = Build Array(w1726) -> (w1725:dbl[])
              n815 = TDMS Write(0:w1713, 5:w1712, 7:"time", 9:w1710, 11:w1708) -> (4:w1709:refnum<k34>, 15:w1707:errorcluster)  [unwired: 1 in, 2 out]
              n816 = Build Array(w1720) -> (w1719:dbl[])
              n817 = TDMS Write(0:w1709, 5:w1712, 7:"centroid X", 9:w1715, 11:w1707) -> (4:w1740:refnum<k34>, 6:w1739:string, 15:w1738:errorcluster)  [unwired: 1 in, 1 out]
              n818 = TDMS Write(0:w1740, 5:w1739, 7:"centroid Y", 9:w1737, 11:w1738) -> (4:w1729:refnum<k34>, 6:w1728:string, 15:w1730:errorcluster)  [unwired: 1 in, 1 out]
              n819 = TDMS Write(0:w1729, 5:w1728, 7:"Motor Axis 1", 9:w1725, 11:w1730) -> (4:w1724:refnum<k34>, 6:w1723:string, 15:w1721:errorcluster)  [unwired: 1 in, 1 out]
              n820 = TDMS Write(0:w1724, 5:w1723, 7:"Motor Axis 2", 9:w1719, 11:w1721) -> (15:w1716:errorcluster)  [unwired: 1 in, 3 out]
            }
            n821 = property on="millisecond timer value" class="DigNum (strict)"() -> ("Value"=w1686:u32)  [unwired: 2 in, 2 out]
            n822 = Tick Count (ms)() -> (millisecond timer value=w1685:u32)
            n823 = Unbundle By Name(w1702) -> ()  [unwired: 1 out]
            n824 = Subtract(x=w1685, y=w1686) -> (x-y=w1689:u32)
            n825 = Divide(x=w1689, y=u32 1000) -> (x/y=w1691:dbl)
            n826 = Quotient & Remainder(x=w1691, y=w1694) -> (x-y*floor(x/y)=w1692:dbl)  [unwired: 1 out]
            n827 = Subtract(x=w1694, y=20.0) -> (x-y=w1696:dbl)
            n828 = Greater?(x=w1692, y=w1696) -> (0:w1693:bool)
            n829 = Select(t="newtdms", s=w1693, f="") -> (s? t:f=w1688:string)
            n830 = call <vilib>:"Add State(s) to Queue__jki_lib_state_machine.vi"("State(s) in (\"\")"=w1706, "State(s) at Back (\"\")"=w1688) -> ("States Out"=w1705:string)  [unwired: 13 in]
          }
          frame "Reset History" {
            # "Your code here.\n(You can make a copy of, or modify, this frame)"
            n831 = for {
              N: 1 -> [_]
              shift-right: [w1759] -> w1751
              shift-left: timestamp[][] [] ("Time") -> [w1761]
              n832 = for {
                N: 12 -> [_]
                tunnel: w1761 -> [w1764] mode=indexing
                tunnel: [w1762] -> w1759 mode=indexing
                n833 = Get Date/Time In Seconds() -> (seconds since 1Jan1904=w1763:timestamp)
                n834 = Build Array (concatenate)(w1764, w1763) -> (w1762:timestamp[])
              }
            }
            n835 = local read "Offset X"() -> (w1750:dbl[][])
            n836 = Bundle By Name(cluster=w1755, "Offset X"=w1750, "Offset Y"=w1750, "Time"=w1751, "Motor X"=w1750) -> (w1754:T35)
            n837 = call <vilib>:"Add State(s) to Queue__jki_lib_state_machine.vi"("State(s) in (\"\")"=w1758) -> ("States Out"=w1757:string)  [unwired: 14 in]
          }
          frame "New Category: 2" {
            # "Your code here.\n(You can make a copy of, or modify, this frame)"
            n838 = call <vilib>:"Add State(s) to Queue__jki_lib_state_machine.vi"("State(s) in (\"\")"=w1768) -> ("States Out"=w1767:string)  [unwired: 14 in]
          }
          frame "stats" {
            # "Your code here.\n(You can make a copy of, or modify, this frame)"
            n839 = Unbundle By Name(w1782) -> ("Offset X"=w1773:dbl[][], "Offset Y"=w1772:dbl[][], "Time"=w1771:timestamp[][], "Motor X"=w1770:dbl[][], "Motor Y"=w1769:dbl[][], "Data Value Reference out"=w1777:refnum<k34>)
            n840 = TDMS List Contents(4:w1776, 7:w1777) -> (0:w1778:errorcluster, 2:w1780:string[], 3:w1779:refnum<k34>)  [unwired: 1 in, 1 out]
            n841 = for {
              tunnel: w1778 -> [w1849]
              tunnel: [w1835] -> w1774 mode=indexing
              tunnel: [w1834] -> w1775
              tunnel: [w1833] -> _
              tunnel: w1779 -> [w1832]
              tunnel: w1780 -> [w1831] mode=indexing
              w1850 = dbl[] [] ("appended array")
              n842 = TDMS Read(0:w1832, 5:w1831, 7:"time", 11:w1849, 12:timestamp[] [] ("appended array")) -> (4:w1864:refnum<k34>, 6:w1860:string, 10:w1841:timestamp[], 15:w1848:errorcluster)  [unwired: 3 in, 2 out]
              n843 = TDMS Read(0:w1864, 5:w1860, 7:"centroid X", 11:w1848, 12:w1850) -> (4:w1863:refnum<k34>, 6:w1859:string, 10:w1844:dbl[], 15:w1847:errorcluster)  [unwired: 3 in, 2 out]
              n844 = TDMS Read(0:w1863, 5:w1859, 7:"centroid Y", 11:w1847, 12:w1850) -> (4:w1862:refnum<k34>, 6:w1858:string, 10:w1843:dbl[], 15:w1846:errorcluster)  [unwired: 3 in, 2 out]
              n845 = TDMS Read(0:w1862, 5:w1858, 7:"Motor Axis 1", 11:w1846, 12:w1850) -> (4:w1861:refnum<k34>, 6:w1857:string, 10:w1842:dbl[], 15:w1845:errorcluster)  [unwired: 3 in, 2 out]
              n846 = TDMS Read(0:w1861, 5:w1857, 7:"Motor Axis 2", 11:w1845, 12:w1850) -> (4:w1833:refnum<k34>, 10:w1840:dbl[], 15:w1834:errorcluster)  [unwired: 3 in, 3 out]
              n847 = Bundle("appended array"=w1841, "appended array"=w1844) -> (w1839:T37)  [unwired: 1 in]
              n848 = Bundle("appended array"=w1841, "appended array"=w1843) -> (w1838:T37)  [unwired: 1 in]
              n849 = Bundle("appended array"=w1841, "appended array"=w1842) -> (w1837:T37)  [unwired: 1 in]
              n850 = Bundle("appended array"=w1841, "appended array"=w1840) -> (w1836:T37)  [unwired: 1 in]
              n851 = Build Array(w1839, w1838, w1837, w1836) -> (w1835:T38)
            }
            n852 = disable-structure shown="Disabled" {
              disable-tunnel: w1781 -> [w1814 _]
              disable-tunnel: w1773 -> [w1813 _]
              disable-tunnel: w1772 -> [w1812 _]
              disable-tunnel: w1771 -> [w1811 _]
              disable-tunnel: w1770 -> [w1810 _]
              disable-tunnel: w1769 -> [w1809 _]
              frame Disabled {
                n853 = for {
                  tunnel: w1814 -> [_] mode=indexing
                  tunnel: w1813 -> [w1824]
                  tunnel: w1812 -> [w1823]
                  tunnel: w1811 -> [w1822]
                  tunnel: w1810 -> [w1818]
                  tunnel: w1809 -> [w1817]
                  tunnel: [w1826] -> _ mode=indexing
                  i -> [w1825]
                  n854 = Index Array(array=w1823, index (row)=w1825) -> (element=w1819:dbl[])  [unwired: 1 in]
                  n855 = Index Array(array=w1818, index (row)=w1825) -> (element=w1816:dbl[])  [unwired: 1 in]
                  n856 = Index Array(array=w1817, index (row)=w1825) -> (element=w1815:dbl[])  [unwired: 1 in]
                  n857 = Index Array(array=w1824, index (row)=w1825) -> (element=w1820:dbl[])  [unwired: 1 in]
                  n858 = Index Array(array=w1822, index (row)=w1825) -> (element=w1821:timestamp[])  [unwired: 1 in]
                  n859 = Bundle("Time"=w1821, "Motor X"=w1816) -> (w1829:cluster{"Time":timestamp[], "Motor X":dbl[]})  [unwired: 1 in]
                  n860 = Bundle("Time"=w1821, "Motor Y"=w1815) -> (w1830:cluster{"Time":timestamp[], "Motor Y":dbl[]})  [unwired: 1 in]
                  n861 = Bundle("Time"=w1821, "Offset X"=w1820) -> (w1828:cluster{"Time":timestamp[], "Offset X":dbl[]})  [unwired: 1 in]
                  n862 = Bundle("Time"=w1821, "Offset Y"=w1819) -> (w1827:cluster{"Time":timestamp[], "Offset Y":dbl[]})  [unwired: 1 in]
                  n863 = Build Array(w1827, w1828, w1829, w1830) -> (w1826:cluster{"Time":timestamp[], "Motor Y":dbl[]}[])
                }
              }
              frame Enabled {
              }
            }
            n864 = Index Array(array=w1774, index (row) #1=0 ("index (row)"), index (row) #2=1 ("index (row)"), index (row) #3=2 ("index (row)"), index (row) #4=3 ("index (row)"), index (row) #5=4 ("index (row)"), index (row) #6=5 ("index (row)"), index (row) #7=6 ("index (row)"), index (row) #8=7 ("index (row)"), index (row) #9=8 ("index (row)"), index (row) #10=9 ("index (row)"), index (row) #11=10 ("index (row)"), index (row) #12=11 ("index (row)")) -> (element #1=→"CCD 1":T38, element #2=→"CCD 2":T38, element #3=→"CCD 3":T38, element #4=→"CCD 4":T38, element #5=→"CCD 5":T38, element #6=→"CCD 6":T38, element #7=→"CCD 7":T38, element #8=→"CCD 8":T38, element #9=→"CCD 9":T38, element #10=→"CCD 10":T38, element #11=→"CCD 11":T38, element #12=→"CCD 12":T38)  [unwired: 12 in]
            n865 = call <vilib>:"Add State(s) to Queue__jki_lib_state_machine.vi"("State(s) in (\"\")"=w1808) -> ("States Out"=w1807:string)  [unwired: 14 in]
          }
          frame "newtdms" {
            # "Your code here.\n(You can make a copy of, or modify, this frame)"
            n866 = Unbundle By Name(w1901) -> ("Data Value Reference out"=w1889:refnum<k34>, "active cams"=w1884:string[])
            n867 = TDMS Close(8:w1899, 11:w1889) -> (0:w1883:errorcluster)  [unwired: 1 out]
            n868 = Get Date/Time In Seconds() -> (seconds since 1Jan1904=w1877:timestamp)
            n869 = call <vilib>:"Clear Errors.vi"("error in (no error)"=w1883) -> ("error out"=w1870:errorcluster)  [unwired: 6 in]
            n870 = Format Date/Time String(time format string (%c)="%Y%m%d", seconds (now)=w1877) -> (date/time string=w1878:string)  [unwired: 1 in]
            n871 = Format Date/Time String(time format string (%c)="%Y%m%d%H%M", seconds (now)=w1877) -> (date/time string=w1875:string)  [unwired: 1 in]
            n872 = property on="new tdms" class="Bool (strict)"("Value"=FALSE ("new tdms")) -> ()  [unwired: 2 in, 2 out]
            n873 = Get Date/Time In Seconds() -> (seconds since 1Jan1904=w1898:timestamp)
            n874 = Format Date/Time String(time format string (%c)="%Y%m%d%H%M", seconds (now)=w1898) -> (date/time string=w1890:string)  [unwired: 1 in]
            n875 = Build Path(base path=w1871, name or relative path=w1878) -> (appended path=w1879:path)
            n876 = Concatenate Strings(w1890, "BeampointingBELLABTL_TRA.tdms" ("string")) -> (w1896:string)
            n877 = String To Path(string=w1896) -> ()  [unwired: 1 out]
            n878 = Concatenate Strings(w1875, "BeampointingBELLABTL_TRA.tdms" ("string")) -> (w1873:string)
            n879 = String To Path(string=w1873) -> (path=w1868:path)
            n880 = call <vilib>:"Check if File or Folder Exists.vi"("error in (no error)"=w1870, "path"=w1879) -> ("error out"=w1882:errorcluster, "file or folder exists?"=w1880:bool, "dup path"=w1881:path)  [unwired: 7 in]
            n881 = case shown="False" w1880 {
              tunnel: w1881 -> [w1907 w1909]
              tunnel: [w1906 w1909] -> w1867
              tunnel: w1882 -> [w1905 w1908]
              tunnel: [w1904 w1908] -> w1869
              frame False {
                n882 = Create Folder(path (use dialog)=w1907, error in=w1905) -> (created path=w1906:path, error out=w1904:errorcluster)  [unwired: 1 in, 1 out]
              }
              frame True {
              }
            }
            n883 = call <vilib>:"Add State(s) to Queue__jki_lib_state_machine.vi"("State(s) in (\"\")"=w1903) -> ("States Out"=w1902:string)  [unwired: 14 in]
            n884 = Build Path(base path=w1867, name or relative path=w1868) -> (appended path=w1891:path)
            n885 = TDMS Open(6:FALSE ("disable buffering (T)"), 7:enum16{"1.0", "2.0"}."2.0" ("file format version (2.0)"), 8:w1869, 10:T15."create or replace" ("operation"), 11:w1891) -> (0:w1887:errorcluster, 3:w1886:refnum<k34>)  [unwired: 2 in]
            n886 = call "TDMSbuffersize.vi"("error in (no error)"=w1887, "group names"=w1884, "Data Value Reference in"=w1886) -> ("error out"=w1866:errorcluster, "Data Value Reference out"=w1885:refnum<k34>)  [unwired: 7 in]
            n887 = Bundle By Name(cluster=w1901, "Data Value Reference out"=w1885) -> (w1900:T35)
            n888 = call <vilib>:"Clear Errors.vi"("error in (no error)"=w1866) -> ("error out"=w1865:errorcluster)  [unwired: 6 in]
          }
          frame "Center" {
            # "Your code here.\n(You can make a copy of, or modify, this frame)"
            n889 = control-ref of="image::1"() -> (w1924:refnum<vi>)
            n890 = control-ref of="image::2"() -> (w1923:refnum<vi>)
            n891 = control-ref of="image::3"() -> (w1922:refnum<vi>)
            n892 = control-ref of="image::4"() -> (w1921:refnum<vi>)
            n893 = control-ref of="image::5"() -> (w1920:refnum<vi>)
            n894 = control-ref of="image::6"() -> (w1919:refnum<vi>)
            n895 = control-ref of="image::7"() -> (w1918:refnum<vi>)
            n896 = control-ref of="image::8"() -> (w1917:refnum<vi>)
            n897 = control-ref of="image::9"() -> (w1916:refnum<vi>)
            n898 = control-ref of="image::10"() -> (w1915:refnum<vi>)
            n899 = control-ref of="image::11"() -> (w1914:refnum<vi>)
            n900 = control-ref of="image::12"() -> (w1913:refnum<vi>)
            n901 = for {
              tunnel: [w1933] -> w1912 mode=indexing
              tunnel: w1911 -> [w1932] mode=indexing
              n902 = Unbundle By Name(w1932) -> ("Target.X::12"=w1931:refnum<vi>, "Target.Y::12"=w1930:refnum<vi>)
              n903 = property class="DigNum (strict)"(reference=w1931) -> ("Value"=w1934:dbl)  [unwired: 1 in, 2 out]
              n904 = property class="DigNum (strict)"(reference=w1930) -> ("Value"=w1935:dbl)  [unwired: 1 in, 2 out]
              n905 = Bundle("Value"=w1934, "Value"=w1935) -> (w1933:cluster{"Value":dbl, "Value":dbl})  [unwired: 1 in]
            }
            n906 = call <vilib>:"Add State(s) to Queue__jki_lib_state_machine.vi"("State(s) in (\"\")"=w1929) -> ("States Out"=w1928:string)  [unwired: 14 in]
            n907 = Build Array(w1924, w1923, w1922, w1921, w1920, w1919, w1918, w1917, w1916, w1915, w1914, w1913) -> (w1925:refnum<vi>[])
            n908 = for {
              tunnel: w1925 -> [w1937] mode=indexing
              tunnel: w1912 -> [w1936] mode=indexing
              n909 = property class="ImageControl"(reference=w1937, "Image Center Position"=w1936) -> ()  [unwired: 1 in, 2 out]
            }
            n910 = property on="Center" class="Bool (strict)"("Value"=FALSE ("Center")) -> ()  [unwired: 2 in, 2 out]
          }
          frame "ImgToAvg" {
            n911 = Decimal String To Number(string=w1947) -> (number=w1944:i32)  [unwired: 2 in, 1 out]
            n912 = Bundle By Name(cluster=w1946, "img to avg"=w1944) -> (w1945:T35)
            n913 = call <vilib>:"Build State String with Arguments__jki_lib_state_machine.vi"("Arguments (\"\")"="T" ("Arguments (\"\")"), "State"=" Device Ini") -> ("State with Arguments"=w1938:string)  [unwired: 4 in]
            n914 = call <vilib>:"Add State(s) to Queue__jki_lib_state_machine.vi"("State(s) in Front (\"\")"=w1938, "State(s) in (\"\")"=w1943) -> ("States Out"=w1942:string)  [unwired: 13 in]
          }
          frame "history" {
            # "Your code here.\n(You can make a copy of, or modify, this frame)"
            n915 = Unbundle By Name(w1957) -> ("Offset X"=w1963:dbl[][], "Offset Y"=w1962:dbl[][], "Mean Centroid X"=w1961:dbl[][], "Mean Centroid Y"=w1960:dbl[][], "Motor X"=w1959:dbl[][], "Motor Y"=w1958:dbl[][], "Time"=w1949:timestamp[][])
            n916 = for {
              tunnel: w1963 -> [w1981] mode=indexing
              tunnel: w1962 -> [w1979] mode=indexing
              tunnel: w1961 -> [w1978] mode=indexing
              tunnel: w1960 -> [w1977] mode=indexing
              tunnel: w1959 -> [w1976] mode=indexing
              tunnel: w1958 -> [w1975] mode=indexing
              tunnel: [w1980] -> w1955 mode=indexing
              tunnel: [w1974] -> w1954 mode=indexing
              tunnel: [w1970] -> w1953 mode=indexing
              tunnel: [w1973] -> w1952 mode=indexing
              tunnel: [w1972] -> w1951 mode=indexing
              tunnel: [w1971] -> w1950 mode=indexing
              tunnel: w1949 -> [w1969] mode=indexing
              tunnel: [w1967] -> w1948 mode=indexing
              w1968 = 0
              n917 = Delete From Array(array=w1976, index=w1968) -> (array with subset deleted=w1972:dbl[])  [unwired: 1 in, 1 out]
              n918 = Delete From Array(array=w1975, index=w1968) -> (array with subset deleted=w1971:dbl[])  [unwired: 1 in, 1 out]
              n919 = Delete From Array(array=w1969, index=w1968) -> (array with subset deleted=w1967:timestamp[])  [unwired: 1 in, 1 out]
              n920 = Delete From Array(array=w1978, index=w1968) -> (array with subset deleted=w1970:dbl[])  [unwired: 1 in, 1 out]
              n921 = Delete From Array(array=w1977, index=w1968) -> (array with subset deleted=w1973:dbl[])  [unwired: 1 in, 1 out]
              n922 = Delete From Array(array=w1979, index=w1968) -> (array with subset deleted=w1974:dbl[])  [unwired: 1 in, 1 out]
              n923 = Delete From Array(array=w1981, index=w1968) -> (array with subset deleted=w1980:dbl[])  [unwired: 1 in, 1 out]
            }
            n924 = call <vilib>:"Add State(s) to Queue__jki_lib_state_machine.vi"("State(s) in (\"\")"=w1966) -> ("States Out"=w1965:string)  [unwired: 14 in]
            n925 = Bundle By Name(cluster=w1957, "Offset X"=w1955, "Offset Y"=w1954, "Mean Centroid X"=w1953, "Mean Centroid Y"=w1952, "Motor X"=w1951, "Motor Y"=w1950, "Time"=w1948) -> (w1956:T35)
          }
        }
        n926 = property on="Box" class="Arr (strict)"() -> ("Value"=w152:T6)  [unwired: 2 in, 2 out]
        n927 = for {
          tunnel: w154 -> [w200]
          tunnel: w153 -> [w208]
          tunnel: w150 -> [w206] mode=indexing
          tunnel: w152 -> [w169] mode=indexing
          tunnel: w147 -> [w198]
          tunnel: w146 -> [w197]
          tunnel: w145 -> [w180]
          i -> [w179]
          w193 = T39 {"Draw"=TRUE, "Target"={"x"=20.0, "y"=20.0}, "Size"={"x"=20.0, "y"=20.0}, "Angle"=1250067.0, "Color"=1250067, "Thickness"=0, "CrosshairLabel"=""} ("Crosshair")
          w188 = T40 {"Left"=0, "Top"=0, "Right"=0, "Bottom"=0} ("Bounding Rectangle")
          n928 = call-poly <userlib>:"Filter 1D Array__ogtk.vi"("items to filter"=w206, "array"=w208) -> ("filtered item indices"=w209:i32[])  [unwired: 4 in, 1 out]
          n929 = Index Array(array=w209) -> (element=w199:i32)  [unwired: 1 in]
          n930 = Index Array(array=w180, index (row)=w179) -> (element=w177:dbl[])  [unwired: 1 in]
          n931 = Index Array(array=w198, index (row)=w179) -> (element=w187:dbl[])  [unwired: 1 in]
          n932 = Index Array(array=w197, index (row)=w179) -> (element=w185:dbl[])  [unwired: 1 in]
          n933 = Index Array(array=w200, index=w199) -> (element=w207:T29)
          n934 = Reverse 1D Array(array=w177) -> (reversed array=w176:dbl[])
          n935 = Unbundle By Name(w207) -> ("Target.X::12"=w211:refnum<vi>, "Target.Y::12"=w210:refnum<vi>)
          n936 = Reverse 1D Array(array=w187) -> (reversed array=w186:dbl[])
          n937 = Reverse 1D Array(array=w185) -> (reversed array=w184:dbl[])
          n938 = Index Array(array=w176) -> (element=w174:dbl)  [unwired: 1 in]
          n939 = Square Root(x=w174) -> (sqrt(x)=w173:dbl)
          n940 = Index Array(array=w184) -> (element=w181:dbl)  [unwired: 1 in]
          n941 = Index Array(array=w186) -> (element=w182:dbl)  [unwired: 1 in]
          n942 = Divide(x=w173, y=2.0) -> (x/y=w171:dbl)
          n943 = property class="DigNum (strict)"(reference=w211) -> ("Value"=w204:dbl)  [unwired: 1 in, 2 out]
          n944 = property class="DigNum (strict)"(reference=w210) -> ("Value"=w203:dbl)  [unwired: 1 in, 2 out]
          n945 = Bundle(cluster=cluster{"xhair size":dbl, "xhair size 2":dbl} {"xhair size"=25.0, "xhair size 2"=25.0} ("size"), "xhair size"=w171, "xhair size 2"=w171) -> (w175:cluster{"xhair size":dbl, "xhair size 2":dbl})
          n946 = Bundle By Name(cluster=w193, "Draw"=TRUE, "Target.x"=w204, "Target.y"=w203, "Size"=w175, "Color"=u32 16774656, "Angle"=0.0, "Thickness"=u8 1) -> (w166:T39)
          n947 = call "draw crosshair imaq.vi"("clear overlay"=TRUE, "Crosshair"=w166, "Bounding Rectangle"=w188, "image in"=w206) -> ("error out"=w191:errorcluster, "image out"=w190:T9)  [unwired: 6 in]
          n948 = Bundle By Name(cluster=w193, "Draw"=TRUE, "Target.x"=w182, "Target.y"=w181, "Size"=w175, "Color"=u32 8322834, "Angle"=0.0, "Thickness"=u8 1) -> (w167:T39)
          n949 = case shown="False" "average centroid" {
            tunnel: w167 -> [_ w216]
            tunnel: w191 -> [_ w221]
            tunnel: w190 -> [w213 w220]
            tunnel: w188 -> [_ w219]
            tunnel: w169 -> [w214 _]
            tunnel: [w212 w218] -> w168
            frame False {
              n950 = call "draw box imaq.vi"("Color"=u32 1244928, "Rectangle"=w214, "image in"=w213) -> ("error out"=w212:errorcluster)  [unwired: 7 in, 1 out]
            }
            frame True {
              n951 = call "draw crosshair imaq.vi"("clear overlay"=FALSE, "error in (no error)"=w221, "Crosshair"=w216, "Bounding Rectangle"=w219, "image in"=w220) -> ("error out"=w218:errorcluster)  [unwired: 5 in, 1 out]
            }
          }
          "error out 3" <- w168
        }
      }
      n952 = control-ref of="This Application"() -> (w136:refnum<vi>)
      n953 = control-ref of="This VI"() -> (w140:refnum<vi>)
      n954 = Current VI's Menubar() -> (w139:refnum<k9>)
      n955 = call "supergui create stop queue.vi"() -> ("STOP Queue out"=w42:refnum<queue>)  [unwired: 11 in]
      n956 = call "GUI_Master_subvi_reentrant_queues.vi"("STOP Queue in"=w42, "This Application"=w136, "error in (no error)"=w137, "tcp data event"=w135, "Caller menu reference"=w139, "Caller VI ref"=w140) -> ("error out"=→"error IO 2":errorcluster)  [unwired: 5 in]
      n957 = Unbundle By Name(w83) -> ("Data Value Reference out"=w82:refnum<k34>)
      n958 = for {
        tunnel: w112 -> [w144] mode=indexing
        tunnel: w111 -> [w143]
        tunnel: [w142] -> w81
        n959 = call "IMAQ Dispose"("Image"=w144, "error in (no error)"=w143) -> ("error out"=w142:errorcluster)  [unwired: 4 in]
      }
      n960 = TDMS Close(8:w81, 11:w82) -> (0:w43:errorcluster)  [unwired: 1 out]
      "error out 2" <- w43
      n961 = Release Queue(queue=w42, error in (no error)=w43) -> ()  [unwired: 1 in, 3 out]
      "Names" <- w52
    }
  }
